vi "TLB Native Dynamic Events ver 0.22.vi"() -> ()   [LabVIEW 2018]
uses:
  Labview Training Phase 2/Enum Controls/States for Action Engine.ctl
  TLB Type Definitions/State Type Definitions.ctl
  TLB Type Definitions/Intruction Type Definitions.ctl
  TLB Type Definitions/Encoder cluster.ctl
  TLB Type Definitions/PING CLUSTER.ctl
  <vilib>/Studica/Studica Toolkit/NavX/NavX.lvlib
  <vilib>/Studica/Studica Toolkit/Background/DIO Channel.ctl
  Underlying VI's/NavX VI/navX type def.ctl
  <vilib>/Studica/Studica Toolkit/Background/I2C Channel.ctl
  TLB Type Definitions/Vision cluster.ctl
  <vilib>/NI_Real-Time Target Support.lvlib
  TLB Type Definitions/Stepper cluster.ctl
  Experimental VI's/Archived VI's/MOTOR CONTROL NO PID Type Def.ctl
  Underlying VI's/I2C Master VI/I2C MASTER Type Def.ctl
  Underlying VI's/I2C Master VI/I2C_MASTER_WRITE_NEW Type Def.ctl
  <vilib>/userdefined/High Color/IMAQdx.ctl
  Underlying VI's/I2C Master VI/Arduino_Interfacing.ctl
  TLB Type Definitions/Yaw Cluster.ctl
  TLB Type Definitions/Time cluster.ctl
  TLB Type Definitions/Y Stepper cluster.ctl
  Underlying VI's/Modified webcam FGV/Webcam AE.ctl
  Underlying VI's/Elasped Timer/Elapsed timer control.ctl
  Underlying VI's/Motor Control VI with PID/MOTOR CONTROL WITH PID AE DATA MODE TYPE DEF.ctl
  Underlying VI's/Motor Control VI with PID/MOTOR CONTROL WITH PID AE DIRECTION TYPE DEF.ctl
  TLB Type Definitions/IR Sensor Type Def.ctl
  <vilib>/myRIO/Common/Instrument Driver Framework/myRIO v1.0/AI/typedefs/AI Channels Enum.ctl
  <vilib>/myRIO/Common/Instrument Driver Framework/myRIO v1.0/AI/typedefs/AI Channels List.ctl
  TLB Type Definitions/Motor Speed Cluster.ctl
  Underlying VI's/IMAQ Create Reference AE/IMAQ Reference AE.ctl
  TLB Type Definitions/Line Sensor Cluster.ctl
  Underlying VI's/Line Sensor AE/Line Sensor AE Type Def.ctl
  <vilib>/Studica/Studica Toolkit/NavX/TypeDefs/Flags/Z900_navX_Flags_CalibrationStatusTypeDef.ctl
  <vilib>/Studica/Studica Toolkit/NavX/TypeDefs/Flags/Z900_navX_Flags_OpStatusTypeDef.ctl
panel:
  out "Front Wall detected":bool
  out "CPU 1 Usage":dbl
  out "CPU 0 Usage":dbl
  out "Line sensors":T1
  out "IR Sensors":T2
  out "Time up":T3
  out "NAVX Values":T4
  out "Stepper position values":T5
  out "Encoder values":T6
  out "Ultrasonic sensors":T7
  out "Stop?":bool
  out "Selected Task":T8=enum."Start Task 9"
  out "Object recognition mode":enum16{"Ball", "Soap", "Gel", "Pipe", "None"}(ring)
  out "Correcte stepper":u8
  out "Image Processing Error":errorcluster
  out "Object Detection":T9
  out "Status":T12 {"OP Status" items=["INITIALIZING", "SELFTEST_IN_PROGRESS", "ERROR", "IMU_AUTOCAL_IN_PROGRESS", "NORMAL"]; "Calibration Status" items=["IMU_CAL_STATE_MASK"=3, "IMU_CAL_STATE_INPROGRESS"=0, "IMU_CAL_STATE_ACCUMULATE"=1, "IMU_CAL_STATE_COMPLETE"=2]}
  out "General Errors":errorcluster
  in  "Red LED":bool
  out "Table obstruct":bool
  out "x-y":dbl
  out "Obstacle detected":bool
  out "Speed & distance":T13
  out "Task selection":u8
  out "NavX Readings":T14
  out "Arduino Data":T15
  out "TASK ENABLE":bool
  out "Rising Edge":bool
  in  "Green LED":bool
  out "State Logic":T16=enum."Startup"
  out "elements":T8[](array[typedef])
  in  "STOP TASK":bool
  in  "OK Button":bool
  in  "STOP":bool
  out "Queue Errors":errorcluster
  out "Action Queue Items":i32
  out "State Logic Queue Items":i32
  out "Action Queues items":string[](array[string])=["Hardware reset", "Software reset", ""]
  out "Action State":string
  # "VISION"
  # "TLB FRAMEWORK STATUS"
  # "System Health Status Update"
  # "Test Programme written by Calvin Loke    Dated: 28 Aug 2019\nTest Programme revised by Dr Alex See   Dated 30 Aug 2019\n\nRevision date: 20/03/2020\nProgramme version:   TLB Native Dynamic Events ver 0.19a"
  # "0: Task 1\n1: Task 2\n2: Task 3\n3: Task 4\n4: Task 5\n5: Task 6\n6: Task 7\n7: Task 8 Ball\n8: Task 8 Soap\n9: Task 8 Gel\n10: Task 8 Pipe\n11: Task 9 Blue\n12: Task 9 Black\n13: Task 9 Green\n14: Task 9 Red\n15: Task 9 Yellow"
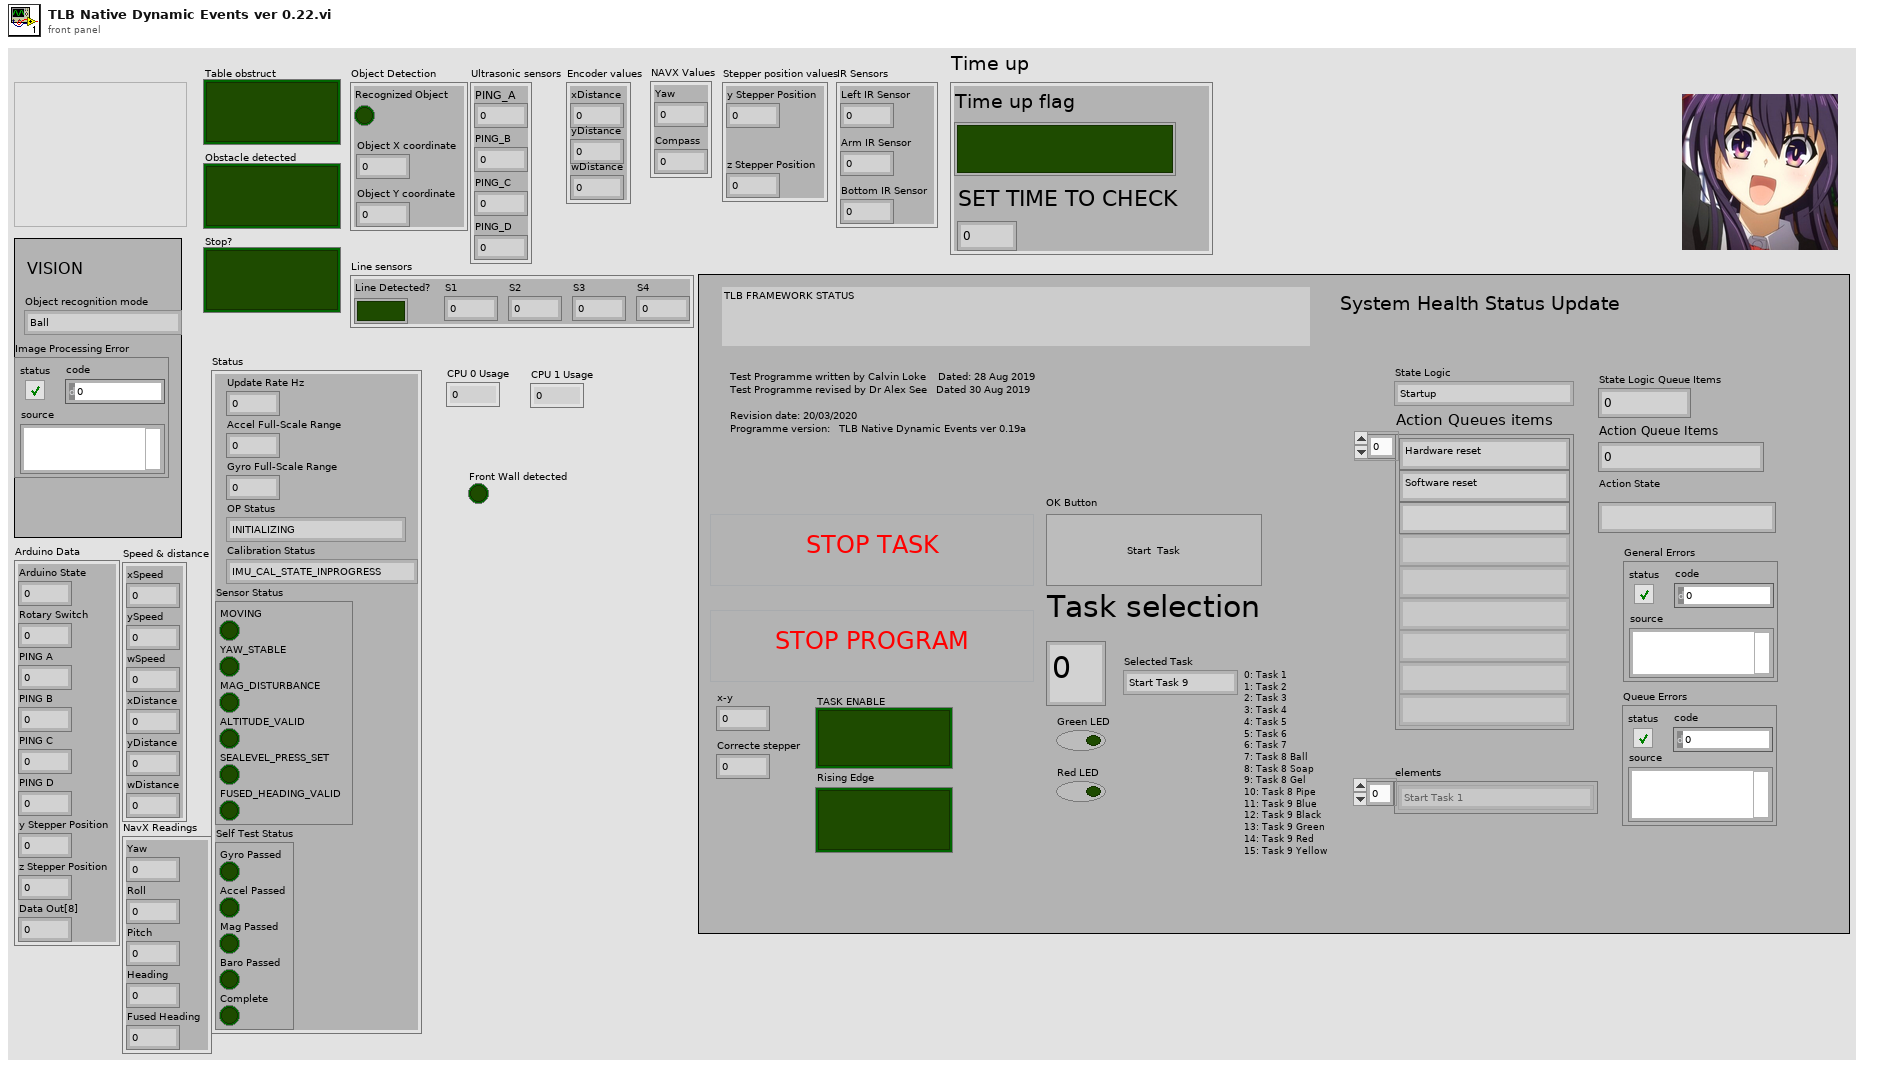
[diagram p1: front panel]
types:
  T1 = typedef "Line Sensor Cluster.ctl" = cluster{"Line Detected?":bool, "S1":dbl, "S2":dbl, "S3":dbl, "S4":dbl}
  T2 = typedef "IR Sensor Type Def.ctl" = cluster{"Left IR Sensor":dbl, "Arm IR Sensor":dbl, "Bottom IR Sensor":dbl}
  T3 = typedef "Time cluster.ctl" = cluster{"Time up flag":bool, "SET TIME TO CHECK":dbl}
  T4 = typedef "Yaw Cluster.ctl" = cluster{"Yaw":dbl, "Compass":dbl}
  T5 = typedef "Stepper cluster.ctl" = cluster{"y Stepper Position":u8, "z Stepper Position":u8}
  T6 = typedef "Encoder cluster.ctl" = cluster{"xDistance":dbl, "yDistance":dbl, "wDistance":dbl}
  T7 = typedef "PING CLUSTER.ctl" = cluster{"PING_A":u8, "PING_B":u8, "PING_C":u8, "PING_D":u8}
  T8 = typedef "Intruction Type Definitions.ctl" = enum16{"None", "Start Task 1", "Start Task 2", "Start Task 3", "Start Task 4", "Start Task 5", "Start Task 6", "Start Task 7", "Start Task 8 - BALL", "Start Task 8 - Gel", "Start Task 8 - Pipe", "Start Task 8 - Soap", "Start Task 9", "Start Task A", "Start Task B", "Exit"}
  T9 = typedef "Vision cluster.ctl" = cluster{"Recognized Object":bool, "Object X coordinate":dbl, "Object Y coordinate":dbl}
  T10 = typedef "NavX.lvlib/Z900_navX_Flags_OpStatusTypeDef.ctl" = u8
  T11 = typedef "NavX.lvlib/Z900_navX_Flags_CalibrationStatusTypeDef.ctl" = u8
  T12 = cluster{"Update Rate Hz":u8, "Accel Full-Scale Range":u8, "Gyro Full-Scale Range":u16, "OP Status":T10, "Calibration Status":T11, "Sensor Status":cluster{"MOVING":bool, "YAW_STABLE":bool, "MAG_DISTURBANCE":bool, "ALTITUDE_VALID":bool, "SEALEVEL_PRESS_SET":bool, "FUSED_HEADING_VALID":bool}, "Self Test Status":cluster{"Gyro Passed":bool, "Accel Passed":bool, "Mag Passed":bool, "Baro Passed":bool, "Complete":bool}}
  T13 = cluster{"xSpeed":dbl, "ySpeed":dbl, "wSpeed":dbl, "xDistance":dbl, "yDistance":dbl, "wDistance":dbl}
  T14 = cluster{"Yaw":dbl, "Roll":dbl, "Pitch":dbl, "Heading":dbl, "Fused Heading":dbl}
  T15 = cluster{"Arduino State":u8, "Rotary Switch":u8, "PING A":u8, "PING B":u8, "PING C":u8, "PING D":u8, "y Stepper Position":u8, "z Stepper Position":u8, "Data Out[8]":u8}
  T16 = typedef "State Type Definitions.ctl" = enum16{"None", "Startup", "Move to Angle", "True Stop", "Idle", "Shutdown", "Task 1A", "Task 1B", "Task 2:Raise Arm", "Task 2:Sensor Mode", "Task 2:Reverse Mode", "Task 3", "Task 4_A", "Task 4_B", "Task 4_C", "Task 4_D", "Task 5A", "Task 5B", "Task 5C", "Task 5D", "Task 5E: POSITION ARM", "Task 5F: ARM GRAB HEIGHT", "Task 5G: CLOSE CLAW", "Task 5H: RAISE ARM", "Task 6_A", "Task 6_B", "Task 7", "Task 8A: RAISE ARM", "Task 8B: MOVE TO BOX", "Task 8C: CAM BURST", "Task 8D: PROCESS IMAGE", "Task 8E: ROBOT ADJUST", "Task 8F: CAM BURST 2", "Task 8G: PROCESS IMAGE 2", "Task 8H: ARM ADJUST", "Task 8I: ARM GRAB HEIGHT", "Task 8J: CLOSE CLAW", "Task 8K: RAISE MY SWORD", "Task 9A: Raise Arm", "Task 9B: Rotate to Angle", "Task 9C: Detect Box", "Task 9D: MOVE FORWARD", "Task 9E: MOVE LEFT", "Task 9F: SCAN IMAGE", "Task 9G: PROCESS COLOUR", "Task 9H: MOVE RIGHT", "Task 9I: SCAN IMAGE", "Task 9J: PROCESS COLOUR", "Task 9K: ROTATE 90 CW", "Task 9L: MOVE FORWARD", "Task 9M: MOVE RIGHT", "Task 9N: SCAN IMAGE", "Task 9O: PROCESS COLOUR", "Task 9P: MOVE RIGHT", "Task 9Q: SCAN IMAGE", "Task 9R: PROCESS COLOUR", "Task A1: Raise Arm", "Task A2: Rotate to Angle", "Task A3: Move Forward", "Task A4: Rotate CW 90"}
  T17 = typedef "Motor Speed Cluster.ctl" = cluster{"ySpeed":dbl, "xSpeed":dbl, "wSpeed":dbl}
  T18 = typedef "Y Stepper cluster.ctl" = cluster{"yStepper desired":u8}
  T19 = typedef "DIO Channel.ctl" = enum16{"Not Connected", "A/DIO1", "A/DIO2", "A/DIO3", "A/DIO4", "A/DIO5", "A/DIO6", "A/DIO7", "A/DIO13", "B/DIO1", "B/DIO2", "B/DIO3", "B/DIO4", "B/DIO5", "B/DIO6", "B/DIO7", "B/DIO13", "C/DIO0", "C/DIO1", "C/DIO2", "C/DIO3", "C/DIO4", "C/DIO5", "C/DIO6", "C/DIO7"}
  T20 = cluster{"DIO Channel":T19, "FPGA VI Reference Out":refnum<k20>}
  T21 = typedef "States for Action Engine.ctl" = enum16{"Initialize", "Write", "Read"}
  T22 = typedef "NI_Real-Time Target Support.lvlib/RT CPU Load.ctl" = cluster{"Total (%)":dbl, "Time Critical (%)":dbl, "Timed Structures (%)":dbl, "High (%)":dbl, "Above Normal (%)":dbl, "Normal (%)":dbl, "Background (%)":dbl, "Idle (%)":dbl, "ISR (%)":dbl}
  T23 = cluster{"CPU loads[0]":T22, "CPU loads[1]":T22, "CPU loads[2]":T22, "CPU loads[3]":T22, "CPU loads[4]":T22, "CPU loads[5]":T22, "CPU loads[6]":T22, "CPU loads[7]":T22, "CPU loads[8]":T22}
  T24 = typedef "navX type def.ctl" = enum16{"Get i2C reference", "Read Values", "Zero Yaw"}
  T25 = typedef "Arduino_Interfacing.ctl" = enum16{"Initialize", "Write to Arduino", "Read From Arduino"}
  T26 = typedef "I2C Channel.ctl" = enum16{"Not Connected", "A", "B"}
  T27 = cluster{"I2C Ref Out":cluster{"I2C Channel":T26, "FPGA VI Reference Out":refnum<k20>}, "Connected":bool, "Slave Address (7-bit)":u8, "Registry":u8[]}
  T28 = typedef "State Type Definitions.ctl" = enum16{"None", "Startup", "Move to Angle", "True Stop", "Idle", "Shutdown", "Task 1", "Task 2:Raise Arm", "Task 2:Sensor Mode", "Task 2:Reverse Mode", "Task 3", "Task 4_A", "Task 4_B", "Task 4_C", "Task 4_D", "Task 5A: ARM CAM HEIGHT", "Task 5B: MOVE TO BOX", "Task 5C: CAM BURST", "Task 5D: PROCESS IMAGE", "Task 5E: POSITION ARM", "Task 5F: ARM GRAB HEIGHT", "Task 5G: CLOSE CLAW", "Task 5H: RAISE ARM", "Task 6_A", "Task 6_B", "Task 7", "Task 8A: RAISE ARM", "Task 8B: MOVE TO BOX", "Task 8C: CAM BURST", "Task 8D: PROCESS IMAGE", "Task 8E: ROBOT ADJUST", "Task 8F: CAM BURST 2", "Task 8G: PROCESS IMAGE 2", "Task 8H: ARM ADJUST", "Task 8I: ARM GRAB HEIGHT", "Task 8J: CLOSE CLAW", "Task 8K: RAISE MY SWORD", "Task 9A: Raise Arm", "Task 9B: Rotate to Angle", "Task 9C: Detect Box", "Task 9D: MOVE FORWARD", "Task 9E: MOVE LEFT", "Task 9F: SCAN IMAGE", "Task 9G: PROCESS COLOUR", "Task 9H: MOVE RIGHT", "Task 9I: SCAN IMAGE", "Task 9J: PROCESS COLOUR", "Task 9K: ROTATE 90 CW", "Task 9L: MOVE FORWARD", "Task 9M: MOVE RIGHT", "Task 9N: SCAN IMAGE", "Task 9O: PROCESS COLOUR", "Task 9P: MOVE RIGHT", "Task 9Q: SCAN IMAGE", "Task 9R: PROCESS COLOUR"}
  T29 = typedef "MOTOR CONTROL WITH PID AE DIRECTION TYPE DEF.ctl" = enum16{"y-axis movement", "x-axis movement", "rotation", "stop", "reset encoders"}
  T30 = typedef "MOTOR CONTROL WITH PID AE DATA MODE TYPE DEF.ctl" = enum16{"Init AE", "Write to AE", "Read from AE"}
  T31 = typedef "Line Sensor AE Type Def.ctl" = enum16{"INIT AE", "READ FROM LINE SENSORS"}
  T32 = typedef "IMAQ Reference AE.ctl" = enum16{"Initialize AE", "Get IMAQ Reference", "Dispose Processing Buffer"}
  T33 = typedef "Elapsed timer control.ctl" = enum16{"Start", "Pause", "Initialize"}
  T34 = typedef "I2C_MASTER_WRITE_NEW Type Def.ctl" = enum16{"Ultrasonic sensors", "Stepper origin", "zStepper 13.3k", "zStepper 13k", "zStepper 12k", "zStepper 11k", "zStepper 10k", "zStepper 9k", "zStepper 8k", "zStepper 7k", "zStepper 6k", "zStepper 5k", "zStepper 4k", "zStepper 3k", "zStepper 2k", "zStepper 1k", "zStepper 900", "zStepper 800", "zStepper 700", "zStepper 600", "zStepper 500", "zStepper 400", "zStepper 300", "zStepper 200", "zStepper 100", "zStepper 0", "yStepper control", "Open Claw", "Close Claw", "Soft Reset"}
  T35 = typedef "Webcam AE.ctl" = enum16{"Initialize Camera", "Open Camera", "Continuous Acquisition", "Close Camera", "Retrieve Image", "Dispose Camera Image Buffer"}
  T36 = typedef "IMAQdx.ctl" = refnum<k21>
  T37 = typedef "MOTOR CONTROL NO PID Type Def.ctl" = enum16{"Init", "Front Back", "Left Right", "Rotate", "Stop", "Latch"}
  T38 = typedef "AI Channels List.ctl" = T39[]
  T39 = typedef "AI Channels Enum.ctl" = enum16{"Not Connected", "AudioIn/Left", "AudioIn/Right", "C/AI0", "C/AI1", "A/AI0", "A/AI1", "A/AI2", "A/AI3", "A/AI4", "A/AI5", "A/AI6", "A/AI7", "B/AI0", "B/AI1", "B/AI2", "B/AI3", "B/AI4", "B/AI5", "B/AI6", "B/AI7", "AI/AI0", "AI/AI1", "AI/AI2", "AI/AI3", "A/AI0 (DIFF)", "A/AI1 (DIFF)", "A/AI2 (DIFF)", "A/AI3 (DIFF)", "B/AI0 (DIFF)", "B/AI1 (DIFF)", "B/AI2 (DIFF)", "B/AI3 (DIFF)"}
  T40 = cluster{"S1":dbl, "S2":dbl, "S3":dbl, "S4":dbl, "Array[4]":dbl, "Array[5]":dbl, "Array[6]":dbl, "Array[7]":dbl, "Array[8]":dbl}
  T41 = typedef "I2C MASTER Type Def.ctl" = enum16{"Last State", "Mode 0", "Mode 1", "Mode 2", "Mode 3", "Mode 4", "Mode 5", "Mode 6", "Mode 7", "Mode 8", "Mode 9", "Mode 10"}
  T42 = typedef "IMAQ Image.ctl" = refnum<image>
  T43 = cluster{"Number of Matches":i32, "Object detected?":bool}
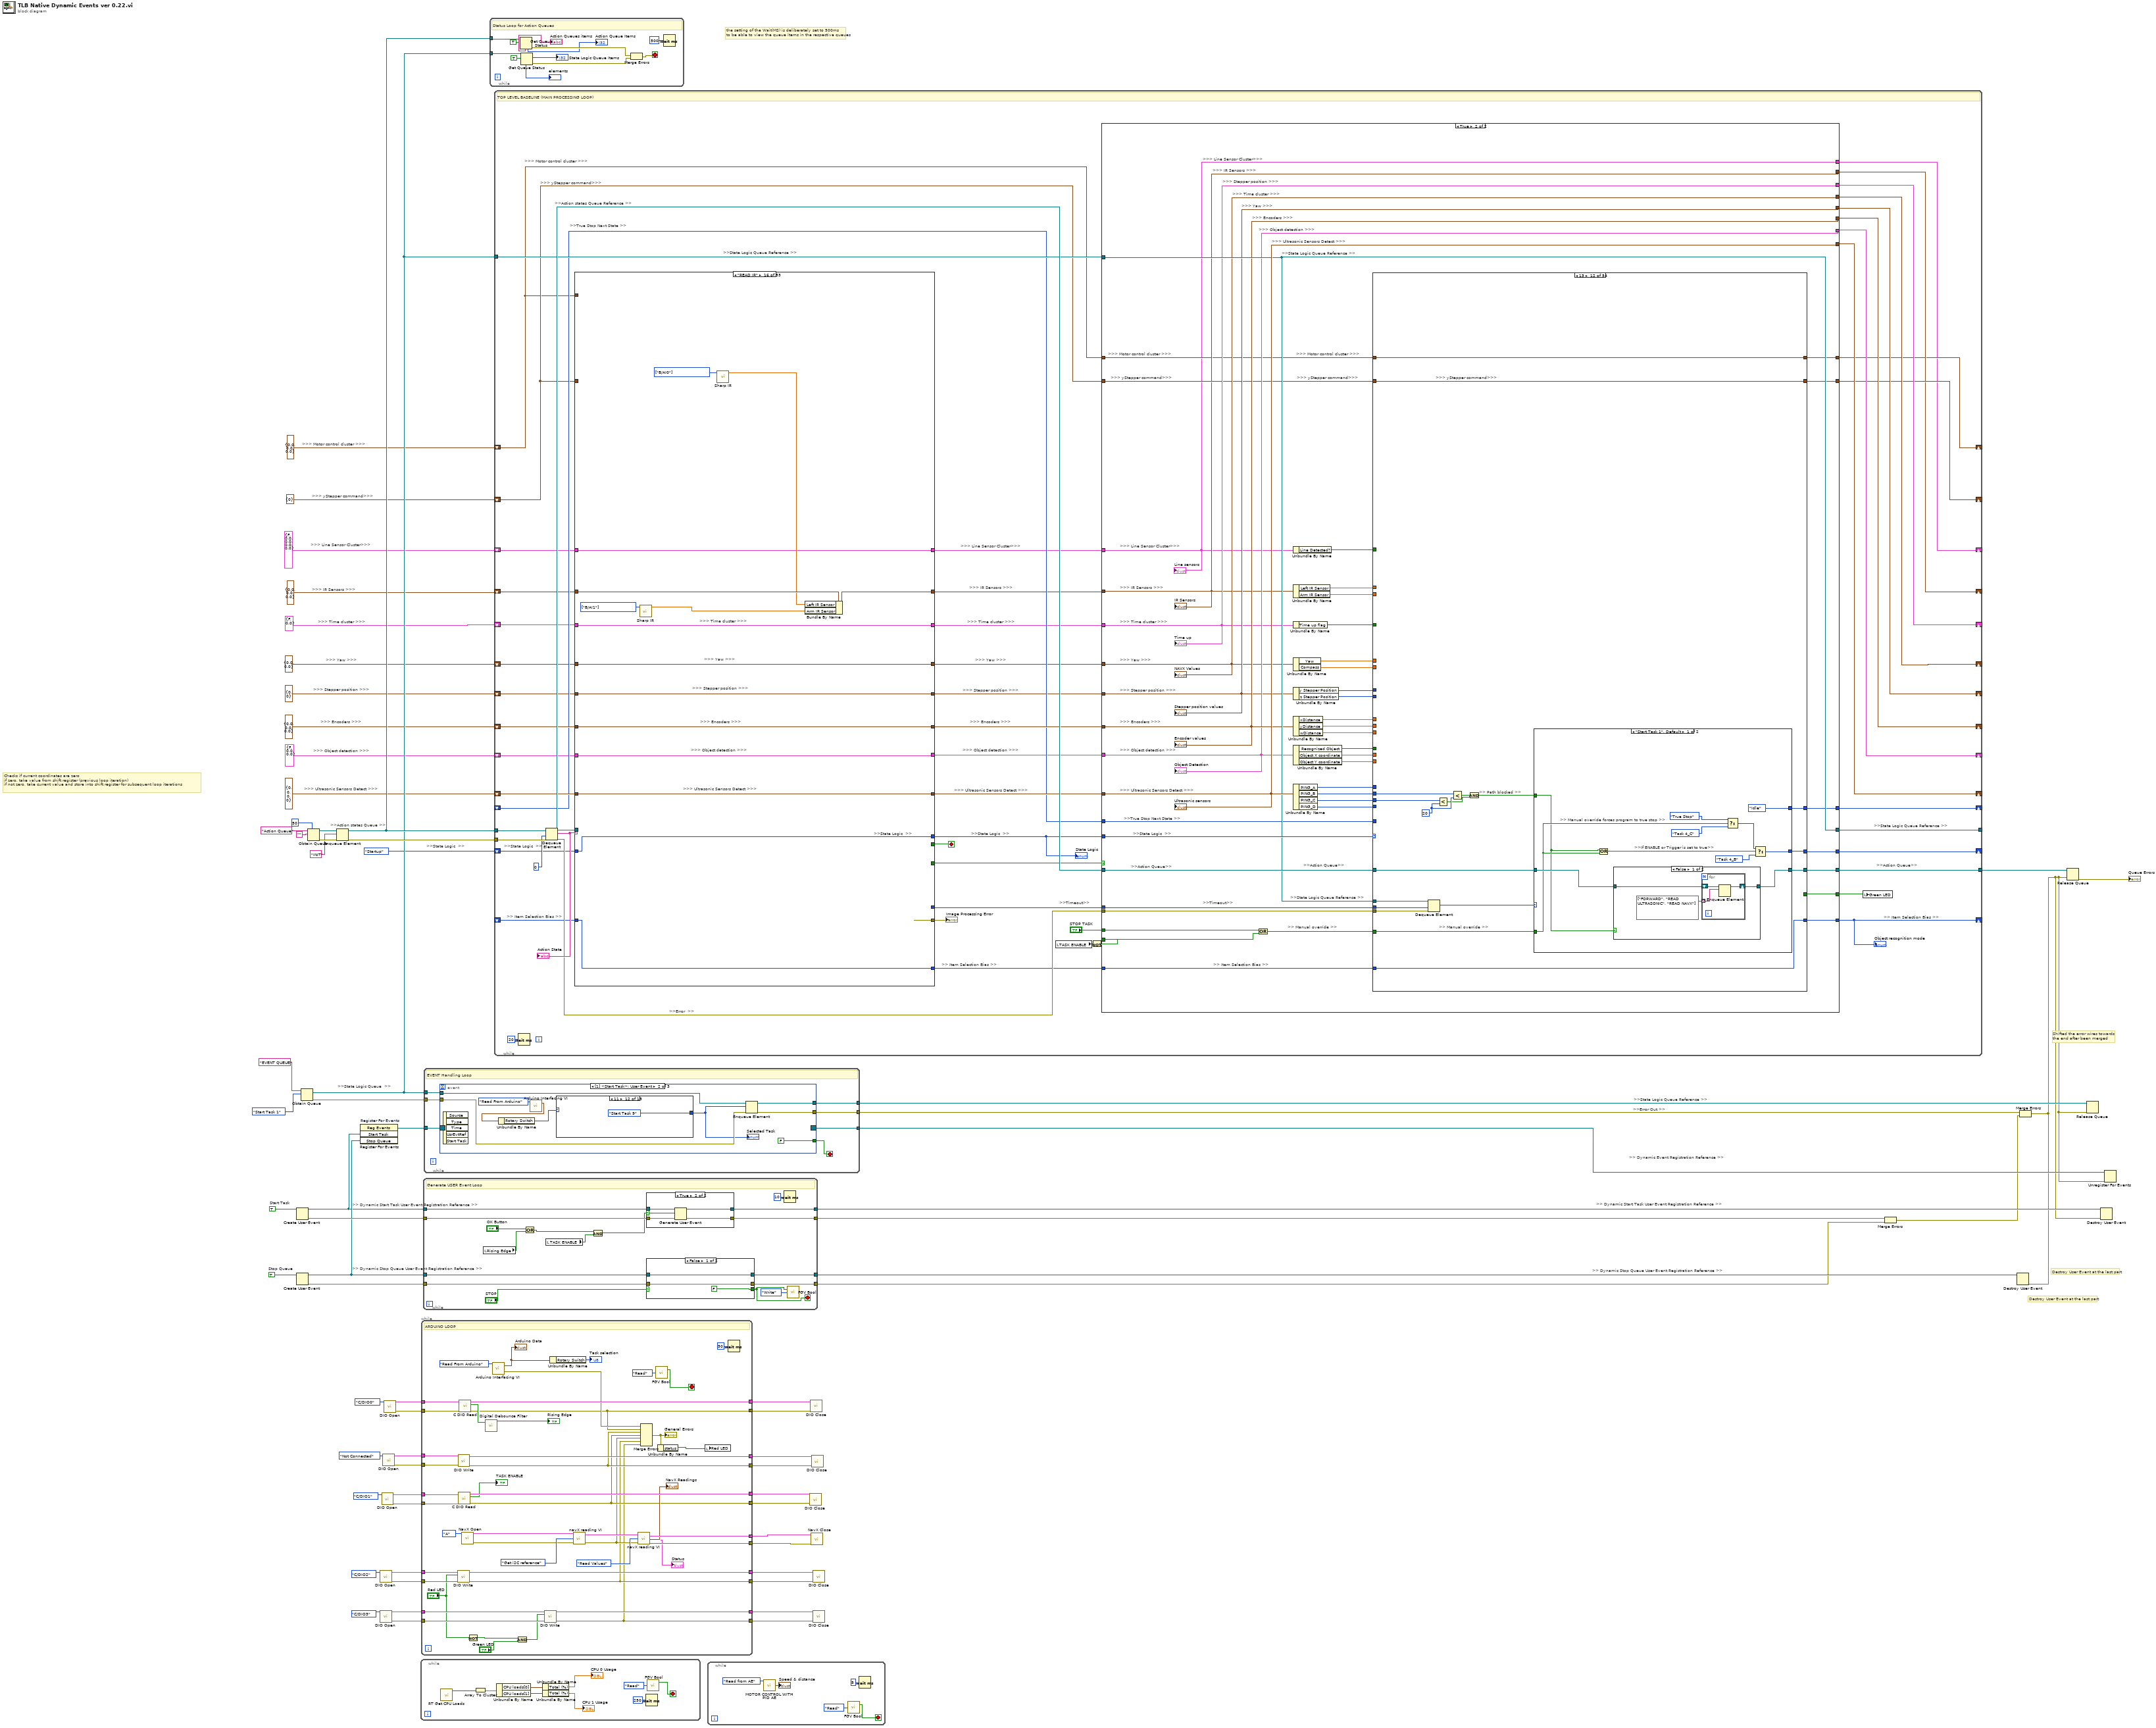
[diagram p0: block diagram]
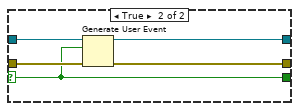
[diagram p2: hidden frame]
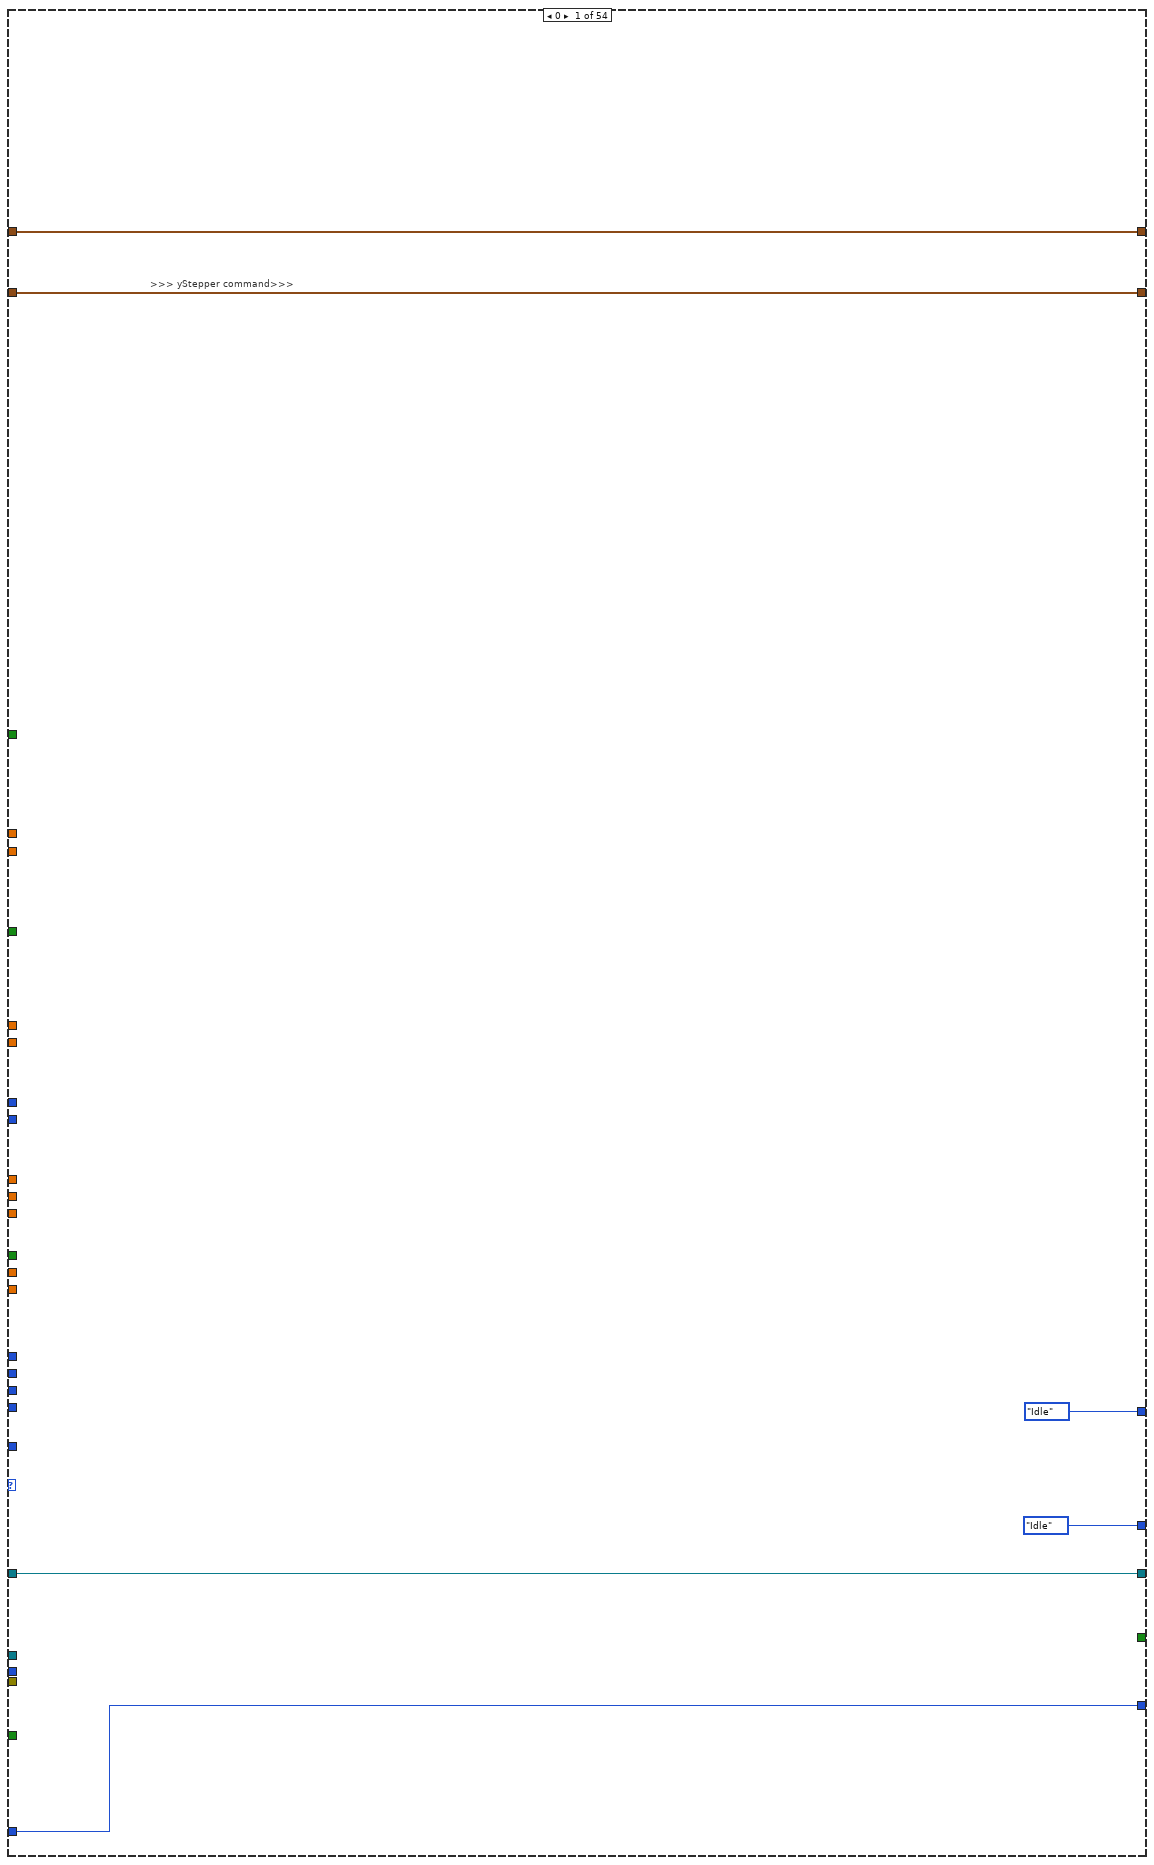
[diagram p5: hidden frame]
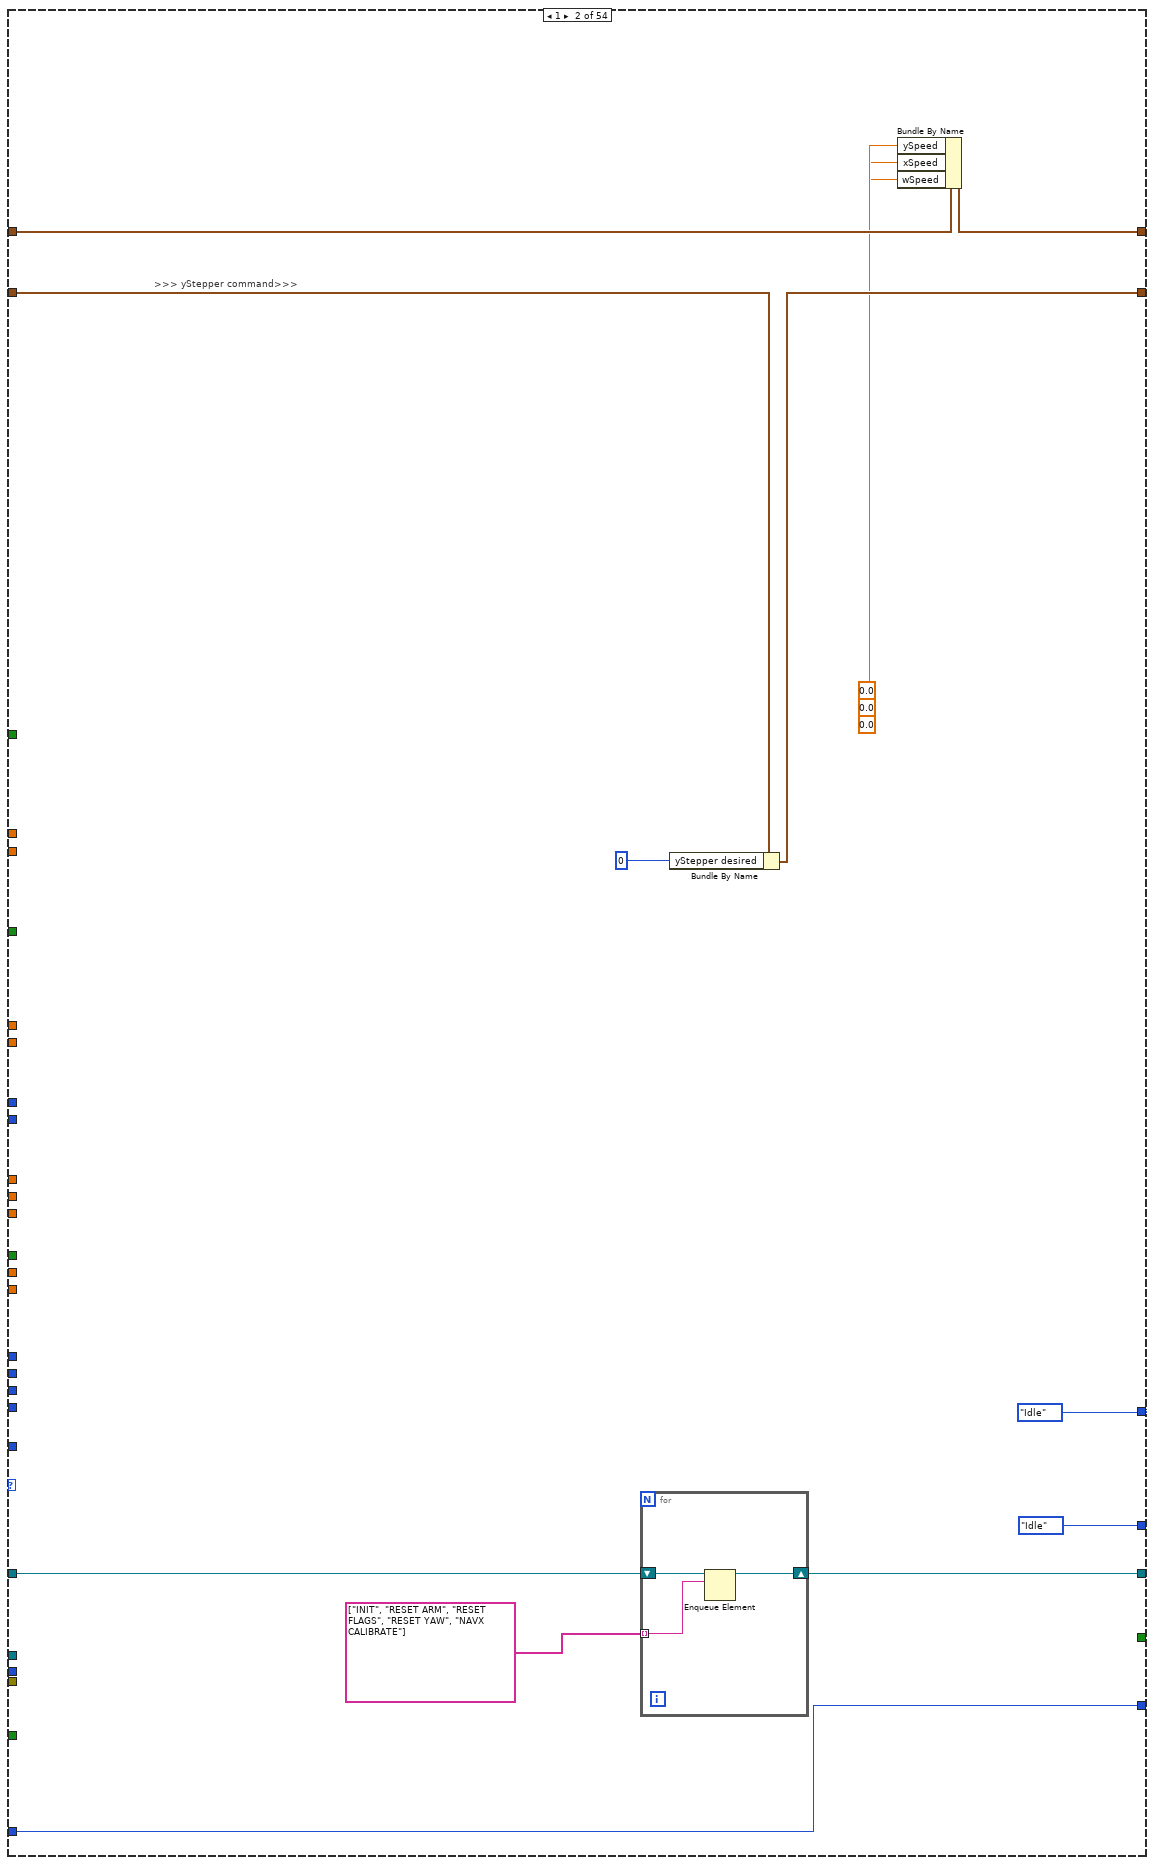
[diagram p6: hidden frame]
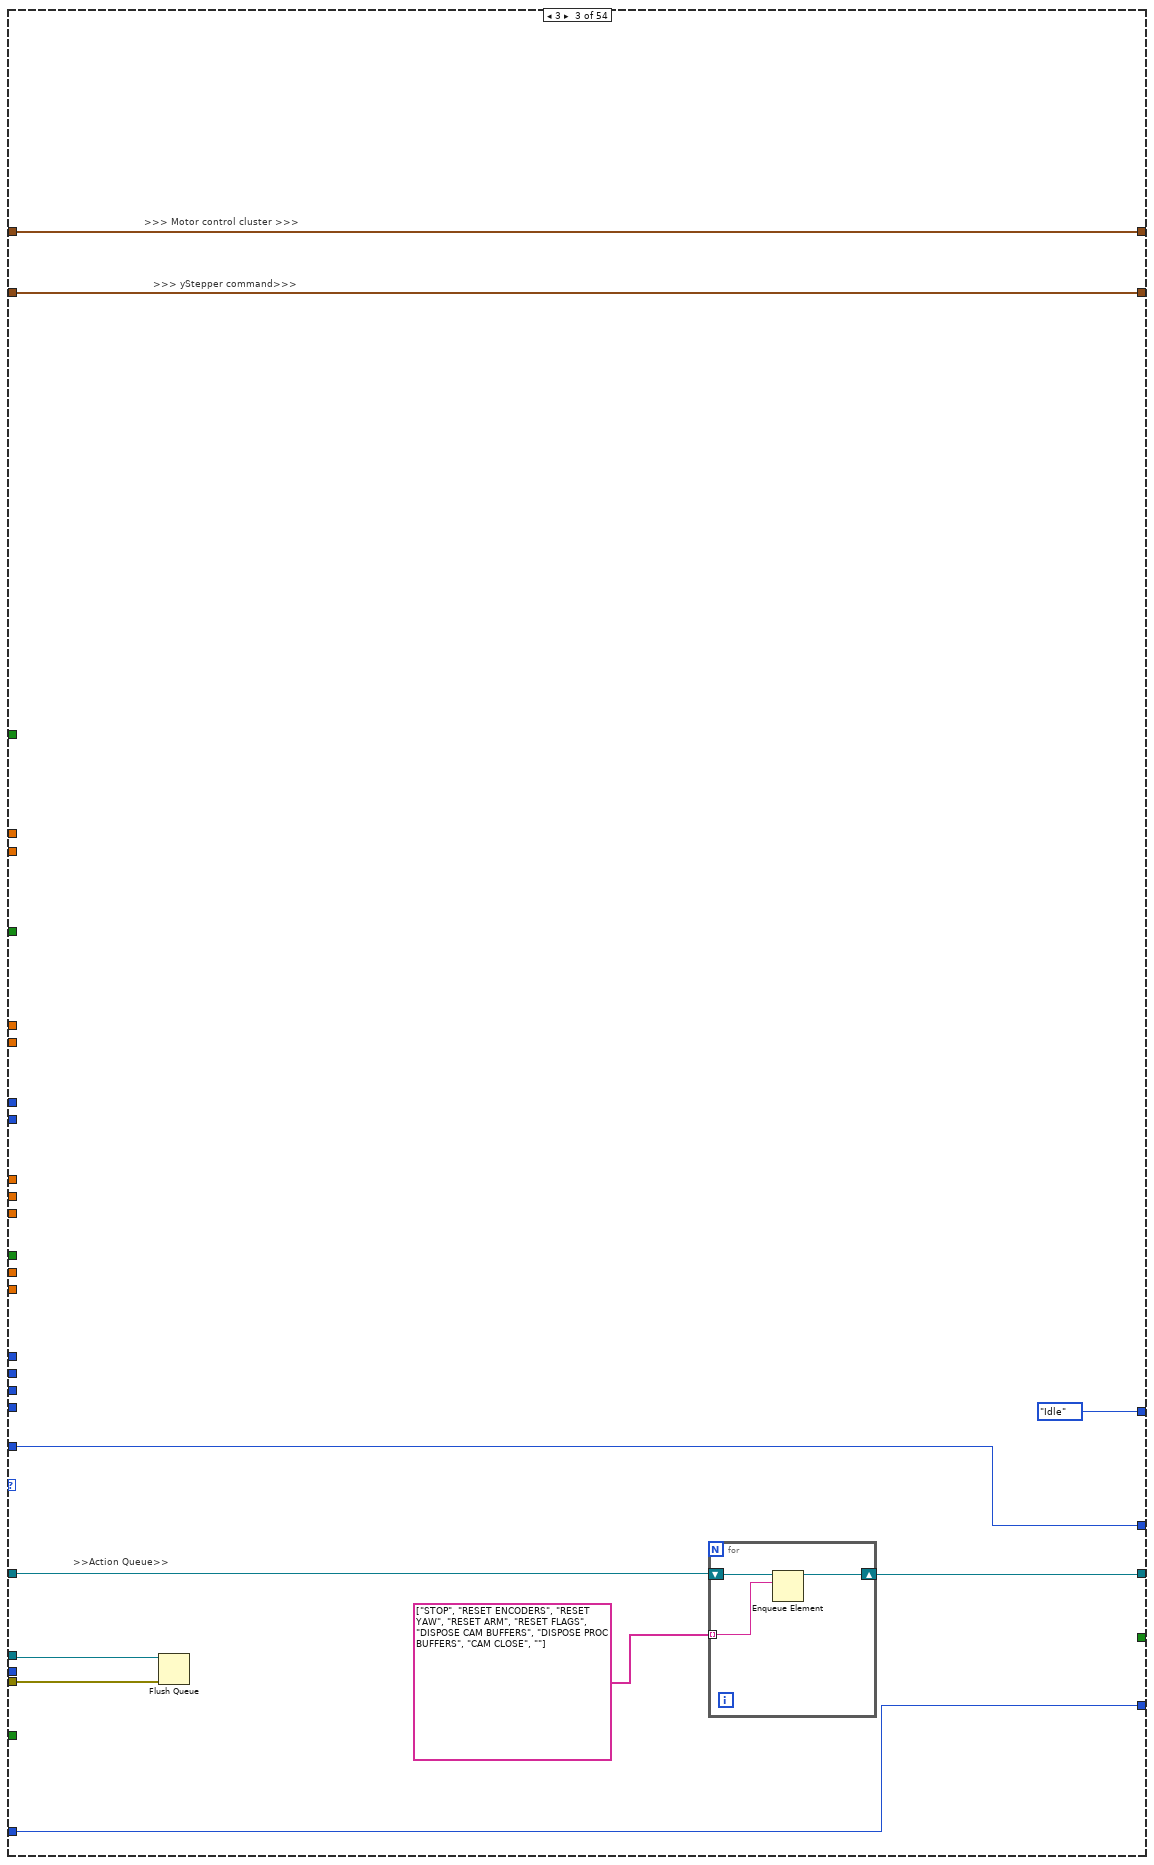
[diagram p7: hidden frame]
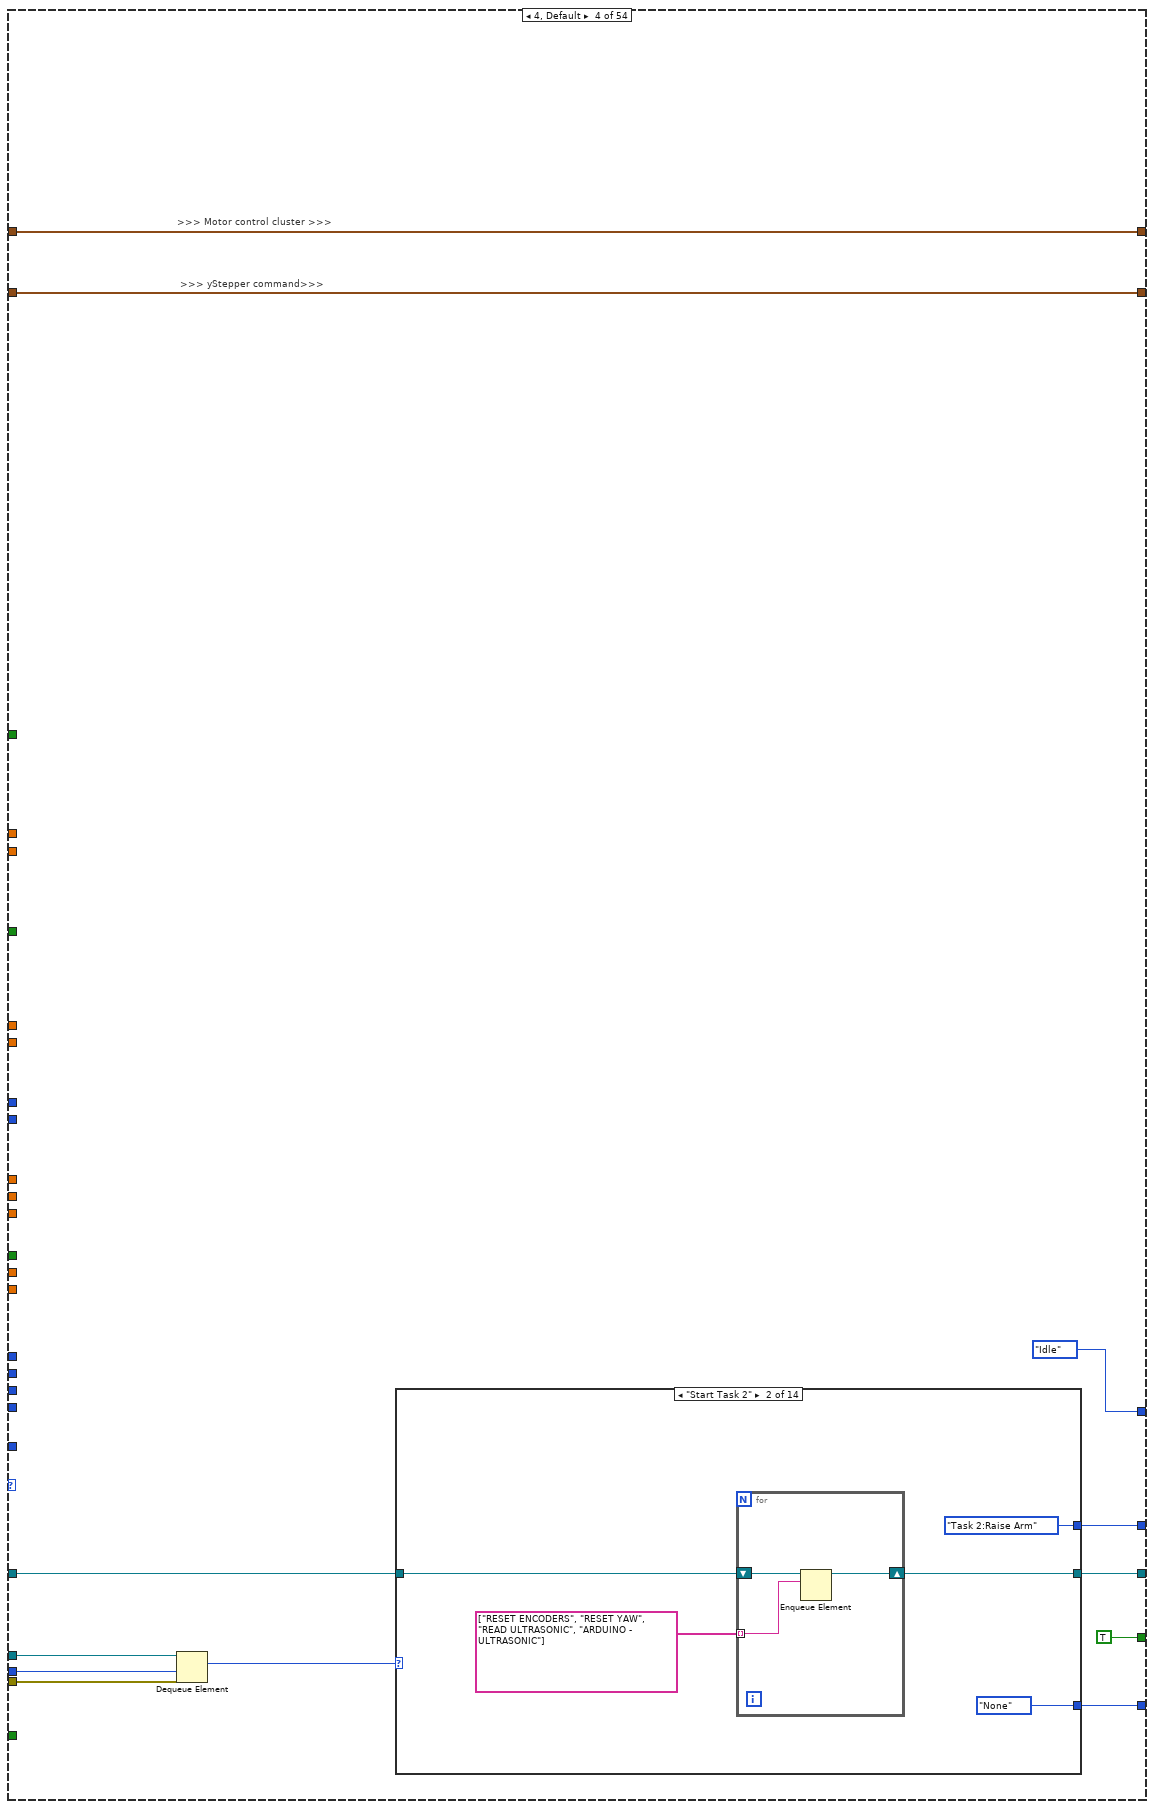
[diagram p8: hidden frame]
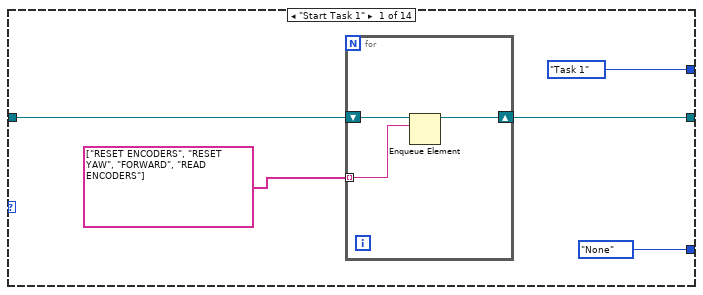
[diagram p9: hidden frame]
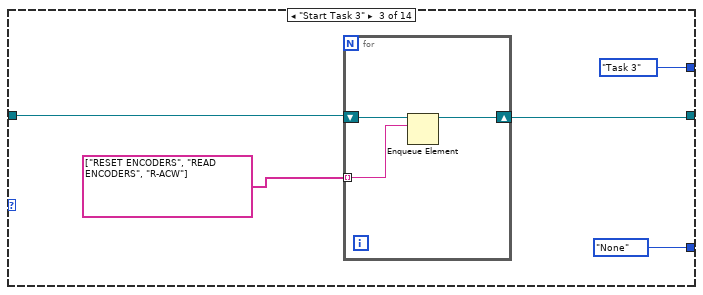
[diagram p10: hidden frame]
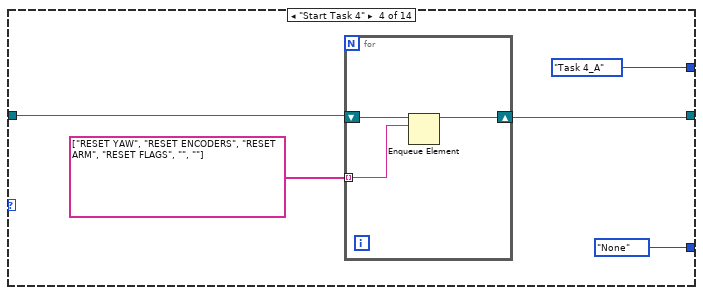
[diagram p11: hidden frame]
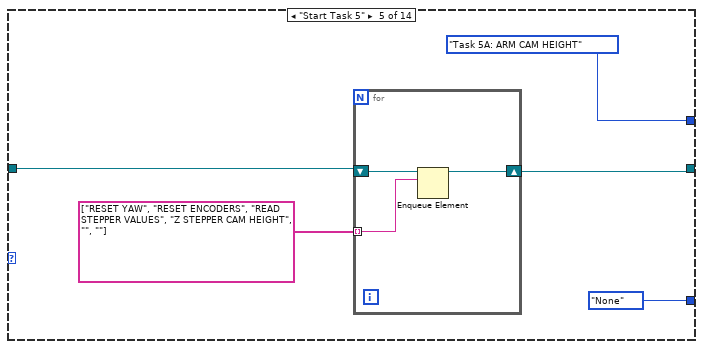
[diagram p12: hidden frame]
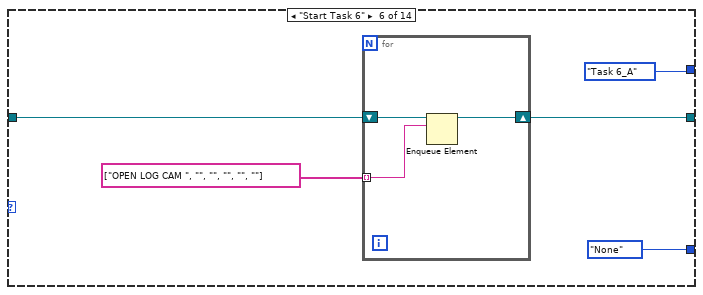
[diagram p13: hidden frame]
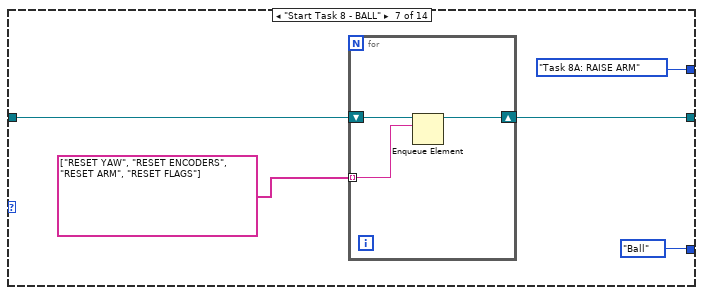
[diagram p14: hidden frame]
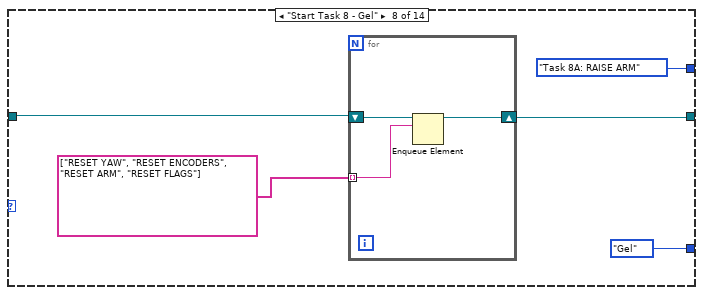
[diagram p15: hidden frame]
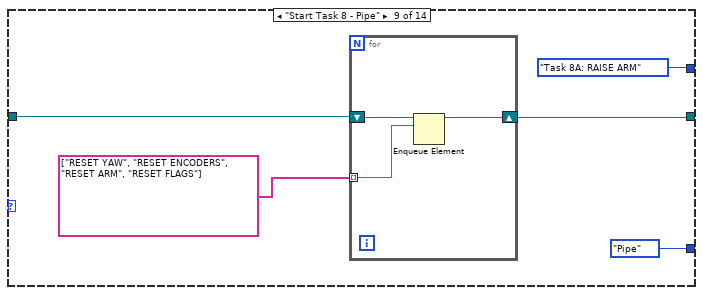
[diagram p16: hidden frame]
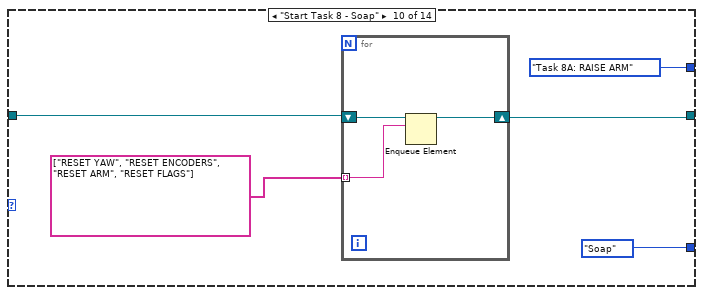
[diagram p17: hidden frame]
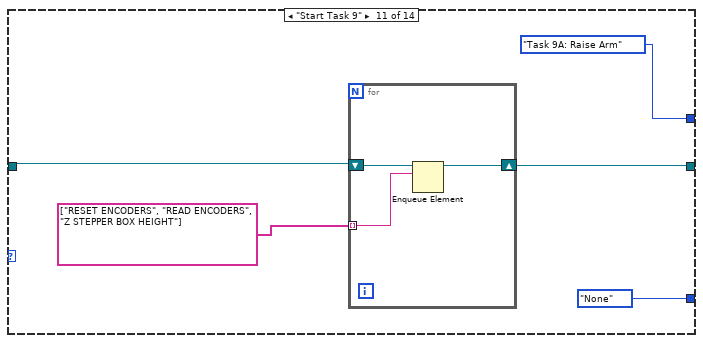
[diagram p18: hidden frame]
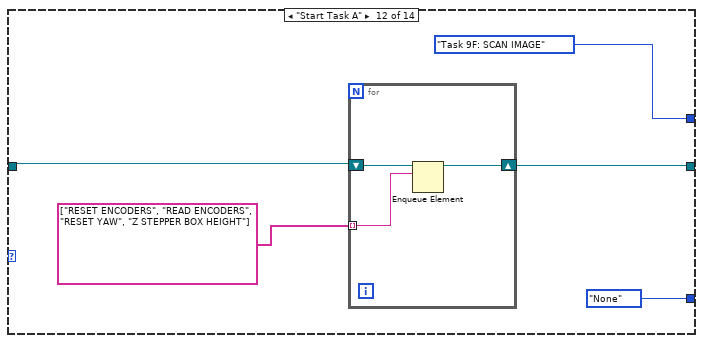
[diagram p19: hidden frame]
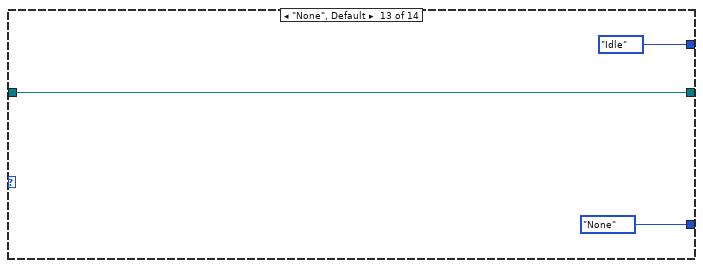
[diagram p20: hidden frame]
diagram:
  w68 = TRUE  # Stop Queue
  w67 = TRUE  # Start Task
  # ">>State Logic  >>"
  # ">>> Line Sensor Cluster>>>"
  # ">>> Motor control cluster >>>"
  # ">>> IR Sensors >>>"
  # "Checks if current coordinates are zero\nif zero, take value from shift register (previous loop iteration)\nif not zero, take current value and store into shift register for subsequent loop iterations"
  # ">>> yStepper command>>>"
  # ">>> Time cluster >>>"
  # ">>> Yaw >>>"
  # ">>> Stepper position >>>"
  # ">>> Encoders >>>"
  # ">>> Object detection >>>"
  # ">>> Ultrasonic Sensors Detect >>>"
  # "the setting of the Wait(MS) is deliberately set to 500ms\nto be able to view the queue items in the respective queues"
  # ">>Error Out >>"
  # ">> Dynamic Stop Queue User Event Registration Reference >>"
  # ">> Dynamic Start Task User Event Registration Reference >>"
  # ">> Dynamic Stop Queue User Event Registration Reference >>"
  # ">> Dynamic Start Task User Event Registration Reference >>"
  # ">> Dynamic Event Registration Reference >>"
  # ">>Action states Queue >>"
  # ">>State Logic Queue  >>"
  # ">>State Logic Queue Reference >>"
  # "Destroy User Event at the last part"
  # "Destroy User Event at the last part"
  # "Shifted the error wires towards\nthe end after been merged"
  n1 = Create User Event(user event datatype=w67) -> (user event=w59:refnum<user-event>, error out=w64:errorcluster)  [unwired: 1 in]
  n2 = Create User Event(user event datatype=w68) -> (user event=w60:refnum<user-event>, error out=w63:errorcluster)  [unwired: 1 in]
  n3 = Obtain Queue(name (unnamed)="EVENT QUEUE", element data type=Intruction_Type_Definitions."Start Task 1" ("Enum")) -> (queue out=w45:refnum<queue>, error out=w51:errorcluster)  [unwired: 3 in, 1 out]
  n4 = Obtain Queue(max queue size (-1, unlimited)=50, name (unnamed)="Action Queue", element data type="") -> (queue out=w54:refnum<queue>, error out=w50:errorcluster)  [unwired: 2 in, 1 out]
  n5 = Enqueue Element(queue=w54, element="INIT", error in (no error)=w50) -> (queue out=w46:refnum<queue>, error out=w49:errorcluster)  [unwired: 1 in, 1 out]
  n6 = register-events "Register For Events"(w59, w60) -> (reference out=w58:refnum<event-registration>)  [unwired: 2 in, 1 out]
  n7 = call <vilib>:"DIO Open.vi"("DIO Channel"=DIO_Channel."C/DIO2") -> ("error out"=w18:errorcluster, "DIO Info Out"=w19:T20)  [unwired: 9 in]
  n8 = call <vilib>:"DIO Open.vi"("DIO Channel"=DIO_Channel."C/DIO3") -> ("error out"=w13:errorcluster, "DIO Info Out"=w14:T20)  [unwired: 9 in]
  n9 = call <vilib>:"DIO Open.vi"("DIO Channel"=DIO_Channel."C/DIO1") -> ("error out"=w23:errorcluster, "DIO Info Out"=w24:T20)  [unwired: 9 in]
  n10 = call <vilib>:"DIO Open.vi"("DIO Channel"=DIO_Channel."Not Connected") -> ("error out"=w28:errorcluster, "DIO Info Out"=w30:T20)  [unwired: 9 in]
  n11 = call <vilib>:"DIO Open.vi"("DIO Channel"=DIO_Channel."C/DIO0") -> ("error out"=w33:errorcluster, "DIO Info Out"=w36:T20)  [unwired: 9 in]
  n12 = while {
    stop <- w75 stop-if-true
    n13 = call <vilib>:"RT Get CPU Loads.vi"() -> ("CPU loads"=w74:T22[])  [unwired: 10 in, 1 out]
    n14 = Array To Cluster(array=w74) -> (cluster=w73:T23)
    n15 = Unbundle By Name(w73) -> ("CPU loads[0]"=w72:T22, "CPU loads[1]"=w71:T22)
    n16 = Unbundle By Name(w72) -> ("Total (%)"=→"CPU 0 Usage":dbl)
    n17 = Unbundle By Name(w71) -> ("Total (%)"=→"CPU 1 Usage":dbl)
    n18 = Wait (ms)(milliseconds to wait=u32 250) -> ()  [unwired: 1 out]
    n19 = call "FGV Bool.vi"("Init/Read/Write State"=States_for_Action_Engine."Read") -> ("Output node"=w75:bool)  [unwired: 2 in, 1 out]
  }
  n20 = while {
    tunnel: w36 -> [w121]
    tunnel: [w120] -> w34
    tunnel: w33 -> [w119]
    tunnel: [w90] -> w32
    tunnel: w30 -> [w116]
    tunnel: [w115] -> w29
    tunnel: w28 -> [w114]
    tunnel: [w89] -> w27
    tunnel: [w113] -> w25
    tunnel: w24 -> [w112]
    tunnel: w23 -> [w111]
    tunnel: [w88] -> w22
    tunnel: w19 -> [w105]
    tunnel: w18 -> [w104]
    tunnel: [w103] -> w17
    tunnel: [w86] -> w16
    tunnel: w14 -> [w102]
    tunnel: w13 -> [w101]
    tunnel: [w100] -> w12
    tunnel: [w85] -> w11
    tunnel: [w97] -> w8
    tunnel: [w96] -> w9
    stop <- w123 stop-if-true
    # "ARDUINO LOOP"
    n21 = call <vilib>:"DIO Write.vi"("error in (no error)"=w104, "Input"="Red LED", "DIO Info In"=w105) -> ("error out"=w86:errorcluster, "DIO Info Out"=w103:T20)  [unwired: 7 in]
    n22 = call <vilib>:"DIO Write.vi"("error in (no error)"=w114, "DIO Info In"=w116) -> ("error out"=w89:errorcluster, "DIO Info Out"=w115:T20)  [unwired: 8 in]
    n23 = call <vilib>:"C DIO Read.vi"("error in (no error)"=w111, "DIO Info In in"=w112) -> ("error out"=w88:errorcluster, "IN"=→"TASK ENABLE":bool, "DIO Info In out"=w113:T20)  [unwired: 7 in]
    n24 = call <vilib>:"C DIO Read.vi"("error in (no error)"=w119, "DIO Info In in"=w121) -> ("error out"=w90:errorcluster, "IN"=w118:bool, "DIO Info In out"=w120:T20)  [unwired: 7 in]
    n25 = call <vilib>:"NavX Open.vi"("I2C Channel"=I2C_Channel."A") -> ("error out"=w107:errorcluster, "NavX Info"=w109:T27)  [unwired: 9 in]
    n26 = Not(x="Red LED") -> (.not. x?=w79:bool)
    n27 = call "Digital Debounce Filter.vi"("Boolean input"=w118) -> ("Rising Edge"=→"Rising Edge":bool)  [unwired: 1 in, 2 out]
    n28 = call "Arduino Interfacing VI.vi"("AE Mode"=Arduino_Interfacing."Read From Arduino") -> ("error out"=w91:errorcluster, "Arduino Data"=w93:T15)  [unwired: 3 in]
    "Arduino Data" <- w93
    n29 = And(x=w79, y="Green LED") -> (x .and. y?=w82:bool)
    n30 = call <vilib>:"DIO Write.vi"("error in (no error)"=w101, "Input"=w82, "DIO Info In"=w102) -> ("error out"=w85:errorcluster, "DIO Info Out"=w100:T20)  [unwired: 7 in]
    n31 = Unbundle By Name(w93) -> ("Rotary Switch"=→"Task selection":u8)
    n32 = call "navX reading VI.vi"("NavX Info In"=w109, "Mode"=navX_type_def."Get i2C reference", "error in (no error)"=w107) -> ("NavX Info Out"=w98:T27, "Error Out"=w87:errorcluster)  [unwired: 2 out]
    n33 = call "navX reading VI.vi"("NavX Info In"=w98, "Mode"=navX_type_def."Read Values", "error in (no error)"=w87) -> ("NavX Info Out"=w97:T27, "NavX Readings"=→"NavX Readings":T14, "Status"=→"Status":T12, "Error Out"=w96:errorcluster)
    n34 = Merge Errors(w91, w90, w89, w88, w87, w86, w85) -> (w83:errorcluster)
    "General Errors" <- w83
    n35 = call "FGV Bool.vi"("Init/Read/Write State"=States_for_Action_Engine."Read") -> ("Output node"=w123:bool)  [unwired: 2 in, 1 out]
    n36 = Unbundle By Name(w83) -> ("status"=w80:bool)
    n37 = local write "Red LED"(w80) -> ()
    n38 = Wait (ms)(milliseconds to wait=u32 50) -> ()  [unwired: 1 out]
  }
  n39 = while {
    tunnel: w59 -> [w141]
    tunnel: w60 -> [w140]
    tunnel: [w139] -> w66
    tunnel: [w138] -> w65
    tunnel: w64 -> [w137]
    tunnel: [w136] -> w62
    tunnel: w63 -> [w135]
    tunnel: [w134] -> w61
    stop <- w132 stop-if-true
    # "Generate USER Event Loop"
    n40 = local read "Rising Edge"() -> (w129:bool)
    n41 = Or(x="OK Button", y=w129) -> (x .or. y?=w128:bool)
    n42 = local read "TASK ENABLE"() -> (w127:bool)
    n43 = And(x=w128, y=w127) -> (x .and. y?=w126:bool)
    n44 = case shown="True" w126 {
      selector: w126 -> [_ w152]
      tunnel: w141 -> [w151 w156]
      tunnel: [w151 w155] -> w138
      tunnel: w137 -> [w150 w154]
      tunnel: [w150 w153] -> w136
      frame False {
      }
      frame True {
        n45 = Generate User Event(user event=w156, event data cluster=w152, error in=w154) -> (user event out=w155:refnum<user-event>, error out=w153:errorcluster)  [unwired: 1 in]
      }
    }
    n46 = case shown="False" "STOP" {
      selector: "STOP" -> [_ w145]
      tunnel: w140 -> [w144 w149]
      tunnel: [w144 w148] -> w139
      tunnel: w135 -> [w143 w147]
      tunnel: [w143 w146] -> w134
      tunnel: [FALSE w145] -> w132
      frame False {
      }
      frame True {
        n47 = Generate User Event(user event=w149, event data cluster=w145, error in=w147) -> (user event out=w148:refnum<user-event>, error out=w146:errorcluster)  [unwired: 1 in]
      }
    }
    n48 = Wait (ms)(milliseconds to wait=u32 10) -> ()  [unwired: 1 out]
    n49 = call "FGV Bool.vi"("Init/Read/Write State"=States_for_Action_Engine."Write", "Input Node"=w132) -> ()  [unwired: 1 in, 2 out]
  }
  n50 = while {
    tunnel: w58 -> [w163]
    tunnel: [w162] -> w57
    tunnel: w45 -> [w160]
    tunnel: [w159] -> w56
    tunnel: w51 -> [w158]
    tunnel: [w157] -> w48
    stop <- w161 stop-if-true
    # "EVENT Handling Loop"
    n51 = event shown="[1] <Start Task>: User Event" {
      selector: w163 -> [_ _ _]
      dyn-events: [_ _ _] -> w162
      timeout: _ -> [_ _ _]
      tunnel: [FALSE FALSE w197] -> w161
      tunnel: w160 -> [w168 w177 w195]
      tunnel: [w167 w176 w196] -> w159
      tunnel: w158 -> [w166 w175 w194]
      tunnel: [w165 w174 w193] -> w157
      event Timeout {
        n52 = event-data() -> ()  [unwired: 1 in, 3 out]
        n53 = Enqueue Element(queue=w168, element=Intruction_Type_Definitions."Start Task 1" ("Enum"), error in (no error)=w166) -> (queue out=w167:refnum<queue>, error out=w165:errorcluster)  [unwired: 1 in, 1 out]
      }
      event User Event {
        n54 = event-data() -> ()  [unwired: 1 in, 5 out]
        n55 = call "Arduino Interfacing VI.vi"("AE Mode"=Arduino_Interfacing."Read From Arduino") -> ("Arduino Data"=w171:T15)  [unwired: 3 in, 1 out]
        n56 = Unbundle By Name(w171) -> ("Rotary Switch"=w170:u8)
        n57 = case shown="11" w170 {
          tunnel: [Intruction_Type_Definitions."Start Task 1" ("Enum") Intruction_Type_Definitions."Start Task 2" ("Enum") Intruction_Type_Definitions."Start Task 3" ("Enum") Intruction_Type_Definitions."Start Task 4" ("Enum") Intruction_Type_Definitions."Start Task 5" ("Enum") Intruction_Type_Definitions."Start Task 6" ("Enum") Intruction_Type_Definitions."Start Task 7" ("Enum") Intruction_Type_Definitions."Start Task 8 - BALL" ("Enum") Intruction_Type_Definitions."Start Task 8 - Soap" ("Enum") Intruction_Type_Definitions."Start Task 8 - Gel" ("Enum") Intruction_Type_Definitions."Start Task 8 - Pipe" ("Enum") Intruction_Type_Definitions."Start Task 9" ("Enum") Intruction_Type_Definitions."None" ("Enum")] -> w173
          frame 0, Default {
          }
          frame 1 {
          }
          frame 2 {
          }
          frame 3 {
          }
          frame 4 {
          }
          frame 5 {
          }
          frame 6 {
          }
          frame 7 {
          }
          frame 8 {
          }
          frame 9 {
          }
          frame 10 {
          }
          frame 11 {
          }
          frame 12 {
          }
        }
        "Selected Task" <- w173
        n58 = Enqueue Element(queue=w177, element=w173, error in (no error)=w175) -> (queue out=w176:refnum<queue>, error out=w174:errorcluster)  [unwired: 1 in, 1 out]
      }
      event User Event {
        n59 = event-data() -> ("Stop Queue"=w197:bool)  [unwired: 1 in, 4 out]
        n60 = Enqueue Element At Opposite End(queue=w195, element=Intruction_Type_Definitions."Exit" ("Enum"), error in (no error)=w194) -> (queue out=w196:refnum<queue>, error out=w193:errorcluster)  [unwired: 1 in, 1 out]
      }
    }
  }
  n61 = while {
    tunnel: w46 -> [w207]
    tunnel: w45 -> [w204]
    stop <- w201 stop-if-true
    # "Status Loop for Action Queues"
    n62 = Get Queue Status(queue=w207, return elements? (F)=TRUE) -> (error out=w203:errorcluster, # elements in queue=→"Action Queue Items":i32, elements=→"Action Queues items":string[])  [unwired: 1 in, 5 out]
    n63 = Get Queue Status(queue=w204, return elements? (F)=TRUE) -> (# pending remove=→"State Logic Queue Items":i32, error out=w202:errorcluster, elements=→"elements":T8[])  [unwired: 1 in, 5 out]
    n64 = Merge Errors(w203, w202) -> (w201:errorcluster)
    n65 = Wait (ms)(milliseconds to wait=u32 500) -> ()  [unwired: 1 out]
  }
  n66 = while {
    tunnel: w45 -> [w251]
    tunnel: w46 -> [w263]
    tunnel: w49 -> [w261]
    tunnel: [w260] -> _
    tunnel: [w259] -> w39
    shift-right: [w252] -> _
    shift-left: T7 {"PING_A"=0, "PING_B"=0, "PING_C"=0, "PING_D"=0} -> [w254]
    shift-right: [w245] -> _
    shift-left: State_Type_Definitions."Startup" ("Enum") -> [w248]
    shift-right: [w241] -> _
    shift-left: T6 {"xDistance"=0.0, "yDistance"=0.0, "wDistance"=0.0} -> [w243]
    shift-right: [w238] -> _
    shift-left: _ -> [w237]
    shift-right: [w234] -> _
    shift-left: T9 {"Recognized Object"=FALSE, "Object X coordinate"=0.0, "Object Y coordinate"=0.0} -> [w236]
    shift-right: [w231] -> _
    shift-left: T5 {"y Stepper Position"=0, "z Stepper Position"=0} -> [w233]
    shift-right: [w228] -> _
    shift-left: T4 {"Yaw"=0.0, "Compass"=0.0} -> [w230]
    shift-right: [w225] -> _
    shift-left: T3 {"Time up flag"=FALSE, "SET TIME TO CHECK"=0.0} -> [w227]
    shift-right: [w223] -> _
    shift-left: T18 {"yStepper desired"=0} -> [w224]
    shift-right: [w219] -> _
    shift-left: T2 {"Left IR Sensor"=0.0, "Arm IR Sensor"=0.0, "Bottom IR Sensor"=0.0} -> [w221]
    shift-right: [w217] -> _
    shift-left: T17 {"ySpeed"=0.0, "xSpeed"=0.0, "wSpeed"=0.0} -> [w218]
    shift-right: [w214] -> _
    shift-left: T1 {"Line Detected?"=FALSE, "S1"=0.0, "S2"=0.0, "S3"=0.0, "S4"=0.0} -> [w216]
    shift-right: [w212] -> _
    shift-left: _ -> [w211]
    stop <- w250 stop-if-true
    # ">>Action Queue>>"
    # ">>State Logic Queue Reference >>"
    # ">>> Line Sensor Cluster>>>"
    # ">>> IR Sensors >>>"
    # ">>> Time cluster >>>"
    # ">>> Object detection >>>"
    # ">>> Yaw >>>"
    # ">>> Ultrasonic Sensors Detect >>>"
    # ">>> Encoders >>>"
    # ">>> Stepper position >>>"
    # ">>State Logic  >>"
    # ">> Item Selection Bias >>"
    # ">> Item Selection Bias >>"
    # ">> Item Selection Bias >>"
    # ">>State Logic  >>"
    # ">>> Motor control cluster >>>"
    # ">>> yStepper command>>>"
    # ">>True Stop Next State >>"
    # ">>Error  >>"
    # ">>Timeout>>"
    # ">>Action states Queue Reference >>"
    # ">>State Logic Queue Reference >>"
    # "TOP LEVEL BASELINE (MAIN PROCESSING LOOP)"
    n67 = Wait (ms)(milliseconds to wait=u32 20) -> ()  [unwired: 1 out]
    n68 = Dequeue Element(queue=w263, timeout in ms (-1)=0, error in (no error)=w261) -> (queue out=w255:refnum<queue>, element=w262:string, error out=w256:errorcluster)  [unwired: 1 out]
    "Action State" <- w262
    n69 = case shown="\"READ IR\"" w262 {
      tunnel: [_ _ _ _ _ _ _ _ _ _ _ _ _ _ _ _ _ _ _ _ 0 w3028 _ _ _ _ _ _ _ _ _ _ _ _ _ _ _ _ _ _ _ _ _ _ _ _ _ _ _ _ _ _ _] -> w258
      tunnel: w255 -> [_ _ _ _ _ _ _ _ _ _ _ _ _ _ _ _ _ _ _ _ _ _ _ _ _ _ _ _ _ _ _ _ _ _ _ _ _ _ _ _ _ _ _ _ _ _ _ _ _ _ _ _ _]
      tunnel: w254 -> [w2724 w2735 w2749 w2762 w2781 w2795 w2808 w2821 w2836 w2850 w2863 w2872 w2889 w2905 w2919 w2931 w2954 w2963 w2992 w3004 w3017 w3029 w3040 w3052 w3069 w3103 w3139 w3152 w3162 w3173 w3185 w3199 w3214 w3225 w3236 w3255 w3265 w3280 w3289 w3301 w3313 w3325 w3334 w3351 w3360 w3378 w3386 w3400 w3414 w3428 w3442 w3456 w3469]
      tunnel: [w2724 w2735 w2749 w2762 w2781 w2795 w2808 w2821 w2836 w2850 w2863 w2872 w2889 w2906 w2919 w2931 w2954 w2963 w2993 w3004 w3017 w3029 w3040 w3052 w3069 w3102 w3138 w3152 w3162 w3173 w3185 w3199 w3214 w3225 w3236 w3255 w3265 w3280 w3289 w3301 w3313 w3325 w3334 w3351 w3360 w3378 w3386 w3400 w3414 w3428 w3442 w3456 w3469] -> w253
      tunnel: [TRUE TRUE _ _ _ _ _ _ _ _ _ _ _ _ _ _ _ _ _ _ _ _ _ _ _ _ _ _ _ _ _ _ _ _ _ _ _ _ _ _ _ _ _ _ _ _ _ _ _ _ _ _ _] -> w250
      tunnel: w248 -> [w2722 w2733 w2748 w2761 w2780 w2794 w2807 w2820 w2835 w2849 w2862 w2871 w2888 w2904 w2918 w2929 w2947 w2962 w2991 w3003 w3014 w3026 w3039 w3051 w3068 w3101 w3137 w3151 w3161 w3172 w3177 w3198 w3213 w3224 w3235 w3254 w3264 w3274 w3288 w3300 w3312 w3324 w3333 w3342 w3359 w3377 w3385 w3399 w3413 w3427 w3441 w3455 w3468]
      tunnel: [_ _ _ _ _ _ _ _ _ _ _ _ _ _ _ _ _ _ _ _ _ TRUE _ _ _ _ _ _ _ _ _ _ _ _ _ _ _ _ _ _ _ _ _ _ _ _ _ _ _ _ _ _ _] -> w247
      tunnel: [w2722 w2733 w2748 w2761 w2780 w2794 w2807 w2820 w2835 w2849 w2862 w2871 w2888 w2904 w2918 w2929 w2947 w2962 w2991 w3003 w3014 w3026 w3039 w3051 w3068 w3101 w3137 w3151 w3161 w3172 w3177 w3198 w3213 w3224 w3235 w3254 w3264 w3274 w3288 w3300 w3312 w3324 w3333 w3342 w3359 w3377 w3385 w3399 w3413 w3427 w3441 w3455 w3468] -> w246
      tunnel: w243 -> [w2721 w2732 w2747 w2764 w2779 w2793 w2806 w2819 w2834 w2848 w2861 w2873 w2887 w2903 w2920 w2933 w2949 w2964 w2990 w3005 w3013 w3025 w3041 w3053 w3064 w3092 w3127 w3150 w3164 w3174 w3182 w3200 w3215 w3226 w3237 w3256 w3267 w3278 w3291 w3303 w3315 w3327 w3336 w3346 w3362 w3380 w3388 w3402 w3416 w3430 w3444 w3458 w3471]
      tunnel: [w2721 w2732 w2747 w2764 w2779 w2793 w2806 w2819 w2834 w2848 w2861 w2873 w2886 w2903 w2920 w2933 w2949 w2964 w2989 w3005 w3013 w3025 w3041 w3053 w3064 w3091 w3126 w3150 w3164 w3174 w3182 w3200 w3215 w3226 w3237 w3256 w3267 w3278 w3291 w3303 w3315 w3327 w3336 w3346 w3362 w3380 w3388 w3402 w3416 w3430 w3444 w3458 w3471] -> w242
      tunnel: w236 -> [w2720 w2731 w2746 w2763 w2778 w2792 w2805 w2818 w2833 w2847 w2859 w2870 w2885 w2902 w2913 w2932 w2948 w2961 w2981 w3002 w3012 w3024 w3038 w3050 w3067 w3096 w3132 w3148 w3163 w3171 w3183 w3197 w3212 w3220 w3234 w3250 w3266 w3279 w3290 w3302 w3314 w3326 w3335 w3345 w3361 w3379 w3387 w3401 w3415 w3429 w3443 w3457 w3470]
      tunnel: [w2720 w2731 w2746 w2763 w2778 w2792 w2805 w2818 w2833 w2847 w2859 w2870 w2885 w2902 w2913 w2932 w2948 w2961 w2980 w3002 w3012 w3024 w3038 w3050 w3066 w3095 w3131 w3148 w3163 w3171 w3183 w3197 w3212 w3220 w3234 w3249 w3266 w3279 w3290 w3302 w3314 w3326 w3335 w3345 w3361 w3379 w3387 w3401 w3415 w3429 w3443 w3457 w3470] -> w235
      tunnel: w233 -> [w2719 w2730 w2745 w2765 w2777 w2791 w2804 w2817 w2832 w2846 w2858 w2869 w2884 w2901 w2921 w2934 w2950 w2960 w2986 w3001 w3011 w3023 w3037 w3049 w3063 w3087 w3122 w3147 w3160 w3170 w3181 w3196 w3211 w3223 w3233 w3257 w3268 w3277 w3287 w3299 w3311 w3323 w3337 w3347 w3363 w3376 w3389 w3403 w3417 w3431 w3445 w3459 w3472]
      tunnel: [w2719 w2730 w2745 w2765 w2777 w2791 w2804 w2817 w2832 w2846 w2858 w2869 w2884 w2901 w2921 w2934 w2950 w2960 w2985 w3001 w3011 w3023 w3037 w3049 w3063 w3086 w3121 w3147 w3160 w3170 w3181 w3196 w3211 w3223 w3233 w3257 w3268 w3277 w3287 w3299 w3311 w3323 w3337 w3347 w3363 w3375 w3389 w3403 w3417 w3431 w3445 w3459 w3472] -> w232
      tunnel: w230 -> [w2718 w2729 w2743 w2766 w2775 w2789 w2802 w2816 w2830 w2844 w2857 w2868 w2883 w2894 w2916 w2935 w2951 w2959 w2976 w3000 w3010 w3022 w3036 w3048 w3062 w3083 w3118 w3146 w3157 w3169 w3180 w3195 w3210 w3222 w3232 w3258 w3269 w3276 w3286 w3296 w3308 w3320 w3338 w3348 w3364 w3370 w3390 w3404 w3418 w3432 w3446 w3460 w3473]
      tunnel: [w2718 w2729 w2743 w2766 w2775 w2789 w2802 w2816 w2830 w2844 w2857 w2868 w2883 w2894 w2915 w2935 w2951 w2959 w2975 w3000 w3010 w3022 w3036 w3048 w3062 w3082 w3117 w3146 w3157 w3169 w3180 w3195 w3210 w3222 w3232 w3258 w3269 w3276 w3286 w3296 w3308 w3320 w3338 w3348 w3364 w3370 w3390 w3404 w3418 w3432 w3446 w3460 w3473] -> w229
      tunnel: w227 -> [w2716 w2728 w2744 w2767 w2776 w2790 w2803 w2815 w2831 w2845 w2856 w2867 w2882 w2893 w2912 w2936 w2952 w2958 w2972 w2997 w3009 w3021 w3035 w3047 w3061 w3080 w3115 w3144 w3156 w3168 w3179 w3194 w3209 w3221 w3231 w3259 w3270 w3275 w3285 w3295 w3307 w3319 w3339 w3349 w3365 w3369 w3384 w3398 w3412 w3426 w3440 w3454 w3467]
      tunnel: [w2716 w2728 w2744 w2767 w2776 w2790 w2803 w2815 w2831 w2845 w2856 w2867 w2882 w2893 w2912 w2936 w2952 w2958 w2972 w2997 w3009 w3021 w3035 w3047 w3060 w3079 w3114 w3144 w3156 w3168 w3179 w3194 w3209 w3221 w3231 w3259 w3270 w3275 w3285 w3295 w3307 w3319 w3339 w3349 w3365 w3369 w3384 w3396 w3410 w3424 w3438 w3452 w3466] -> w226
      tunnel: w224 -> [_ _ _ _ _ _ _ _ _ _ _ _ _ _ _ _ _ _ _ _ _ _ _ _ _ _ _ _ _ _ _ _ _ _ _ _ _ _ _ _ _ _ _ _ w3356 _ _ _ _ _ _ _ _]
      tunnel: [w2715 w2727 w2738 w2757 w2770 w2784 w2798 w2811 w2826 w2839 w2853 w2866 w2876 w2892 w2909 w2927 w2953 w2957 w2969 w2996 w3008 w3020 w3034 w3044 w3054 w3073 w3106 w3143 w3155 w3167 w3184 w3188 w3203 w3218 w3229 w3243 w3262 w3281 w3284 w3294 w3306 w3318 w3330 w3350 w3354 w3368 w3383 w3393 w3407 w3421 w3435 w3449 w3463] -> w220
      tunnel: w221 -> [w2715 w2727 w2738 w2757 w2770 w2784 w2798 w2811 w2826 w2839 w2853 w2866 w2876 w2892 w2909 w2928 w2953 w2957 w2969 w2996 w3008 w3020 w3034 w3044 w3054 w3074 w3107 w3143 w3155 w3167 w3184 w3188 w3203 w3218 w3229 w3243 w3262 w3281 w3284 w3294 w3306 w3318 w3330 w3350 w3354 w3368 w3383 w3393 w3407 w3421 w3435 w3449 w3463]
      tunnel: w218 -> [_ _ _ _ _ _ _ _ w2825 _ _ _ _ _ _ _ _ _ _ _ _ _ _ _ _ _ _ _ _ _ _ _ _ _ _ _ _ _ _ _ _ _ _ _ _ _ _ _ _ _ _ _ _]
      tunnel: w216 -> [w2714 w2726 w2737 w2751 w2769 w2783 w2797 w2810 w2823 w2838 w2852 w2865 w2875 w2891 w2908 w2923 w2946 w2956 w2967 w2995 w3007 w3019 w3033 w3043 w3057 w3076 w3110 w3142 w3154 w3166 w3176 w3187 w3202 w3217 w3228 w3240 w3261 w3272 w3283 w3293 w3305 w3317 w3329 w3341 w3353 w3367 w3382 w3392 w3406 w3420 w3434 w3448 w3462]
      tunnel: [w2714 w2726 w2737 w2751 w2769 w2783 w2797 w2810 w2823 w2838 w2852 w2865 w2875 w2891 w2908 w2923 w2945 w2956 w2967 w2995 w3007 w3019 w3033 w3043 w3056 w3075 w3109 w3142 w3154 w3166 w3176 w3187 w3202 w3217 w3228 w3240 w3261 w3272 w3283 w3293 w3305 w3317 w3329 w3341 w3353 w3367 w3382 w3392 w3406 w3420 w3434 w3448 w3462] -> w215
      tunnel: [_ _ _ _ _ _ _ _ _ _ _ _ _ _ _ _ _ _ _ _ _ _ _ _ _ _ _ _ _ _ _ _ _ _ _ w3239 _ _ _ _ _ _ _ _ _ _ _ _ _ _ _ _ _] -> w213
      tunnel: w211 -> [w2713 w2725 w2736 w2750 w2768 w2782 w2796 w2809 w2822 w2837 w2851 w2864 w2874 w2890 w2907 w2922 w2937 w2955 w2965 w2994 w3006 w3018 w3032 w3042 w3058 w3077 w3111 w3141 w3153 w3165 w3175 w3186 w3201 w3216 w3227 w3238 w3260 w3271 w3282 w3292 w3304 w3316 w3328 w3340 w3352 w3366 w3381 w3391 w3405 w3419 w3433 w3447 w3461]
      tunnel: [w2713 w2725 w2736 w2750 w2768 w2782 w2796 w2809 w2822 w2837 w2851 w2864 w2874 w2890 w2907 w2922 w2937 w2955 w2965 w2994 w3006 w3018 w3032 w3042 w3058 w3077 w3111 w3141 w3153 w3165 w3175 w3186 w3201 w3216 w3227 w3238 w3260 w3271 w3282 w3292 w3304 w3316 w3328 w3340 w3352 w3366 w3381 w3391 w3405 w3419 w3433 w3447 w3461] -> w210
      frame "Exit" {
        # ">>State Logic  >>"
        # ">>> Time cluster >>>"
        # ">>> Yaw >>>"
        # ">>> Stepper position >>>"
        # ">>> Encoders >>>"
        # ">>> Object detection >>>"
        # ">>> Ultrasonic Sensors Detect >>>"
        n70 = call "Imaq Dispose"("All Images? (No)"=TRUE) -> ()  [unwired: 5 in, 1 out]
      }
      frame "----Movement States----" {
        # ">>State Logic  >>"
        # ">>> Time cluster >>>"
        # ">>> Yaw >>>"
        # ">>> Stepper position >>>"
        # ">>> Encoders >>>"
        # ">>> Object detection >>>"
        # ">>> Ultrasonic Sensors Detect >>>"
      }
      frame "FORWARD" {
        # ">>State Logic  >>"
        # ">>> Time cluster >>>"
        # ">>> Yaw >>>"
        # ">>> Stepper position >>>"
        # ">>> Encoders >>>"
        # ">>> Object detection >>>"
        # ">>> Ultrasonic Sensors Detect >>>"
        n71 = Unbundle By Name(w2743) -> ("Yaw"=w2739:dbl)
        n72 = call "MOTOR CONTROL WITH PID AE.vi"("Yaw"=w2739, "Speed"=30.0, "Direction"=MOTOR_CONTROL_WITH_PID_AE_DIRECTION_TYPE_DEF."y-axis movement", "AE Mode"=MOTOR_CONTROL_WITH_PID_AE_DATA_MODE_TYPE_DEF."Write to AE") -> ()  [unwired: 1 out]
      }
      frame "FORWARD - IR ASSIST" {
        # ">>State Logic  >>"
        # ">>> Time cluster >>>"
        # ">>> Yaw >>>"
        # ">>> Stepper position >>>"
        # ">>> Encoders >>>"
        # ">>> Object detection >>>"
        # ">>> Ultrasonic Sensors Detect >>>"
        n73 = Unbundle By Name(w2757) -> ("Left IR Sensor"=w2756:dbl)
        n74 = Subtract(x=w2756, y=20.0) -> (x-y=w2754:dbl)
        n75 = Multiply(x=w2754, y=0.25) -> (x*y=w2752:dbl)
        n76 = call "MOTOR CONTROL WITH PID AE.vi"("Yaw"=w2752, "Speed"=30.0, "Direction"=MOTOR_CONTROL_WITH_PID_AE_DIRECTION_TYPE_DEF."y-axis movement", "AE Mode"=MOTOR_CONTROL_WITH_PID_AE_DATA_MODE_TYPE_DEF."Write to AE") -> ()  [unwired: 1 out]
      }
      frame "LEFT" {
        # ">>State Logic  >>"
        # ">>> Time cluster >>>"
        # ">>> Yaw >>>"
        # ">>> Stepper position >>>"
        # ">>> Encoders >>>"
        # ">>> Object detection >>>"
        # ">>> Ultrasonic Sensors Detect >>>"
        n77 = Unbundle By Name(w2775) -> ("Yaw"=w2772:dbl)
        n78 = call "MOTOR CONTROL WITH PID AE.vi"("Yaw"=w2772, "Speed"=-20.0, "Direction"=MOTOR_CONTROL_WITH_PID_AE_DIRECTION_TYPE_DEF."x-axis movement", "AE Mode"=MOTOR_CONTROL_WITH_PID_AE_DATA_MODE_TYPE_DEF."Write to AE") -> ()  [unwired: 1 out]
      }
      frame "RIGHT" {
        # ">>> Time cluster >>>"
        # ">>> Yaw >>>"
        # ">>> Stepper position >>>"
        # ">>> Encoders >>>"
        # ">>> Object detection >>>"
        # ">>> Ultrasonic Sensors Detect >>>"
        n79 = Unbundle By Name(w2789) -> ("Yaw"=w2785:dbl)
        n80 = call "MOTOR CONTROL WITH PID AE.vi"("Yaw"=w2785, "Speed"=20.0, "Direction"=MOTOR_CONTROL_WITH_PID_AE_DIRECTION_TYPE_DEF."x-axis movement", "AE Mode"=MOTOR_CONTROL_WITH_PID_AE_DATA_MODE_TYPE_DEF."Write to AE") -> ()  [unwired: 1 out]
      }
      frame "R-ACW" {
        # ">>> IR Sensors >>>"
        # ">>> Time cluster >>>"
        # ">>> Yaw >>>"
        # ">>> Stepper position >>>"
        # ">>> Encoders >>>"
        # ">>> Object detection >>>"
        # ">>> Ultrasonic Sensors Detect >>>"
        n81 = call "MOTOR CONTROL WITH PID AE.vi"("Speed"=10.0, "Direction"=MOTOR_CONTROL_WITH_PID_AE_DIRECTION_TYPE_DEF."rotation", "AE Mode"=MOTOR_CONTROL_WITH_PID_AE_DATA_MODE_TYPE_DEF."Write to AE") -> ()  [unwired: 1 in, 1 out]
      }
      frame "R-CW" {
        (unwired) -0.2 ("Speed")
        # ">>> Time cluster >>>"
        # ">>> Yaw >>>"
        # ">>> Stepper position >>>"
        # ">>> Encoders >>>"
        # ">>> Object detection >>>"
        # ">>> Ultrasonic Sensors Detect >>>"
        n82 = call "MOTOR CONTROL WITH PID AE.vi"("Speed"=-10.0, "Direction"=MOTOR_CONTROL_WITH_PID_AE_DIRECTION_TYPE_DEF."rotation", "AE Mode"=MOTOR_CONTROL_WITH_PID_AE_DATA_MODE_TYPE_DEF."Write to AE") -> ()  [unwired: 1 in, 1 out]
      }
      frame "X AXIS - SLOW" {
        # ">>> Line Sensor Cluster>>>"
        # ">>> IR Sensors >>>"
        # ">>> Time cluster >>>"
        # ">>> Yaw >>>"
        # ">>> Stepper position >>>"
        # ">>> Encoders >>>"
        # ">>> Object detection >>>"
        # ">>> Ultrasonic Sensors Detect >>>"
        n83 = Unbundle By Name(w2825) -> ("xSpeed"=w2824:dbl)
        n84 = Unbundle By Name(w2830) -> ("Yaw"=w2827:dbl)
        n85 = call "MOTOR CONTROL WITH PID AE.vi"("Yaw"=w2827, "Speed"=w2824, "Direction"=MOTOR_CONTROL_WITH_PID_AE_DIRECTION_TYPE_DEF."x-axis movement", "AE Mode"=MOTOR_CONTROL_WITH_PID_AE_DATA_MODE_TYPE_DEF."Write to AE") -> ()  [unwired: 1 out]
      }
      frame "REVERSE" {
        # ">>> Time cluster >>>"
        # ">>> Yaw >>>"
        # ">>> Stepper position >>>"
        # ">>> Encoders >>>"
        # ">>> Object detection >>>"
        # ">>> Ultrasonic Sensors Detect >>>"
        n86 = Unbundle By Name(w2844) -> ("Yaw"=w2840:dbl)
        n87 = call "MOTOR CONTROL WITH PID AE.vi"("Yaw"=w2840, "Speed"=-50.0, "Direction"=MOTOR_CONTROL_WITH_PID_AE_DIRECTION_TYPE_DEF."y-axis movement", "AE Mode"=MOTOR_CONTROL_WITH_PID_AE_DATA_MODE_TYPE_DEF."Write to AE") -> ()  [unwired: 1 out]
      }
      frame "STOP" {
        n88 = Wait (ms)(milliseconds to wait=u32 100) -> ()  [unwired: 1 out]
        n89 = call "MOTOR CONTROL WITH PID AE.vi"("Direction"=MOTOR_CONTROL_WITH_PID_AE_DIRECTION_TYPE_DEF."stop", "AE Mode"=MOTOR_CONTROL_WITH_PID_AE_DATA_MODE_TYPE_DEF."Write to AE") -> ()  [unwired: 2 in, 1 out]
      }
      frame "----SENSOR READING---- " {
      }
      frame "READ ENCODERS" {
        # ">>> Time cluster >>>"
        # ">>> Yaw >>>"
        # ">>> Stepper position >>>"
        # ">>> Object detection >>>"
        # ">>> Current encoder distance >>>"
        # ">>> Ultrasonic Sensors Detect >>>"
        n90 = call "MOTOR CONTROL WITH PID AE.vi"("AE Mode"=MOTOR_CONTROL_WITH_PID_AE_DATA_MODE_TYPE_DEF."Read from AE") -> ("Speed & distance"=w2880:T13)  [unwired: 3 in]
        n91 = Unbundle By Name(w2880) -> ("xDistance"=w2879:dbl, "yDistance"=w2878:dbl, "wDistance"=w2877:dbl)
        n92 = Bundle By Name(cluster=w2887, "xDistance"=w2879, "yDistance"=w2878, "wDistance"=w2877) -> (w2886:T6)
      }
      frame "READ ULTRASONIC" {
        (unwired) navX_type_def."Read Values" ("Mode")
        (unwired) MOTOR_CONTROL_NO_PID_Type_Def."Latch" ("Direction")
        # ">>> Line Sensor Cluster>>>"
        # ">>> IR Sensors >>>"
        # ">>State Logic  >>"
        # ">>> Time cluster >>>"
        # ">>> Ultrasonic Sensors Detect >>>"
        # ">>> Object detection >>>"
        # ">>> Encoders >>>"
        # ">>> Stepper position >>>"
        # ">>> Yaw >>>"
        n93 = call "Arduino Interfacing VI.vi"("AE Mode"=Arduino_Interfacing."Read From Arduino") -> ("Arduino Data"=w2899:T15)  [unwired: 3 in, 1 out]
        n94 = Unbundle By Name(w2899) -> ("PING A"=w2898:u8, "PING B"=w2897:u8, "PING C"=w2896:u8, "PING D"=w2895:u8)
        n95 = Bundle By Name(cluster=w2905, "PING_A"=w2898, "PING_B"=w2897, "PING_C"=w2896, "PING_D"=w2895) -> (w2906:T7)
      }
      frame "READ NAVX" {
        # ">> Item Selection Bias >>"
        # ">>State Logic  >>"
        # ">>> Line Sensor Cluster>>>"
        # ">>> IR Sensors >>>"
        # ">>> Time cluster >>>"
        # ">>> Yaw >>>"
        # ">>> Ultrasonic Sensors Detect >>>"
        # ">>> Object detection >>>"
        # ">>> Encoders >>>"
        # ">>> Stepper position >>>"
        n96 = call "navX reading VI.vi"("Mode"=navX_type_def."Read Values") -> ("NavX Readings"=w2911:T14)  [unwired: 2 in, 3 out]
        n97 = Unbundle By Name(w2911) -> ("Heading"=w2910:dbl)
        n98 = Unbundle By Name(w2911) -> ("Yaw"=w2914:dbl)
        n99 = Bundle By Name(cluster=w2916, "Yaw"=w2914, "Compass"=w2910) -> (w2915:T4)
      }
      frame "READ IR" {
        w2925 = T38 [enum."B/AI1"] items=["Not Connected", "AudioIn/Left", "AudioIn/Right", "C/AI0", "C/AI1", "A/AI0", "A/AI1", "A/AI2", "A/AI3", "A/AI4", "A/AI5", "A/AI6", "A/AI7", "B/AI0", "B/AI1", "B/AI2", "B/AI3", "B/AI4", "B/AI5", "B/AI6", "B/AI7", "AI/AI0", "AI/AI1", "AI/AI2", "AI/AI3", "A/AI0 (DIFF)", "A/AI1 (DIFF)", "A/AI2 (DIFF)", "A/AI3 (DIFF)", "B/AI0 (DIFF)", "B/AI1 (DIFF)", "B/AI2 (DIFF)", "B/AI3 (DIFF)"] ("AI Channel")
        w2930 = T38 [enum."B/AI0"] items=["Not Connected", "AudioIn/Left", "AudioIn/Right", "C/AI0", "C/AI1", "A/AI0", "A/AI1", "A/AI2", "A/AI3", "A/AI4", "A/AI5", "A/AI6", "A/AI7", "B/AI0", "B/AI1", "B/AI2", "B/AI3", "B/AI4", "B/AI5", "B/AI6", "B/AI7", "AI/AI0", "AI/AI1", "AI/AI2", "AI/AI3", "A/AI0 (DIFF)", "A/AI1 (DIFF)", "A/AI2 (DIFF)", "A/AI3 (DIFF)", "B/AI0 (DIFF)", "B/AI1 (DIFF)", "B/AI2 (DIFF)", "B/AI3 (DIFF)"] ("AI Channel")
        # ">>State Logic  >>"
        # ">>> Time cluster >>>"
        # ">>> Ultrasonic Sensors Detect >>>"
        # ">>> Object detection >>>"
        # ">>> Encoders >>>"
        # ">>> Stepper position >>>"
        # ">>> Yaw >>>"
        n100 = call <vilib>:"Sharp IR.vi"("AI Channel"=w2925) -> ("Sharp IR Distance"=w2924:dbl)  [unwired: 8 in, 2 out]
        n101 = call <vilib>:"Sharp IR.vi"("AI Channel"=w2930) -> ("Sharp IR Distance"=w2926:dbl)  [unwired: 8 in, 2 out]
        n102 = Bundle By Name(cluster=w2928, "Left IR Sensor"=w2926, "Arm IR Sensor"=w2924) -> (w2927:T2)
      }
      frame "READ LINE SENSOR" {
        # ">>> IR Sensors >>>"
        # ">>> Line Sensor Cluster>>>"
        # ">>State Logic  >>"
        # ">>> Time cluster >>>"
        # ">>> Object detection >>>"
        # ">>> Yaw >>>"
        # ">>> Ultrasonic Sensors Detect >>>"
        # ">>> Encoders >>>"
        # ">>> Stepper position >>>"
        n103 = call "Line Sensor AE.vi"("AE State"=Line_Sensor_AE_Type_Def."READ FROM LINE SENSORS") -> ("Line Detected?"=w2943:bool, "Line Sensor Raw Values"=w2942:T40)
        n104 = Unbundle By Name(w2942) -> ("S1"=w2941:dbl, "S2"=w2940:dbl, "S3"=w2939:dbl, "S4"=w2938:dbl)
        n105 = Bundle By Name(cluster=w2946, "Line Detected?"=w2943, "S1"=w2941, "S2"=w2940, "S3"=w2939, "S4"=w2938) -> (w2945:T1)
      }
      frame "----SYSTEM MODES----" {
        (unwired) I2C_MASTER_Type_Def."Last State" ("Arduino Mode")
        # ">>> Object detection >>>"
        # ">>> Yaw >>>"
        # ">>> Ultrasonic Sensors Detect >>>"
        # ">>> Encoders >>>"
        # ">>> Stepper position >>>"
      }
      frame "INIT" {
        w2987 = u8 0
        w2988 = 0.0
        # ">>> IR Sensors >>>"
        # ">>> IR Sensors >>>"
        # ">>> Line Sensor Cluster>>>"
        # ">>> Time cluster >>>"
        # ">>> Object detection >>>"
        # ">>> Yaw >>>"
        # ">>> Ultrasonic Sensors Detect >>>"
        # ">>> Encoders >>>"
        # ">>> Stepper position >>>"
        # ">>State Logic  >>"
        n106 = call "Arduino Interfacing VI.vi"("AE Mode"=Arduino_Interfacing."Initialize") -> ()  [unwired: 3 in, 2 out]
        n107 = call "FGV Bool.vi"("Init/Read/Write State"=States_for_Action_Engine."Initialize") -> ()  [unwired: 2 in, 2 out]
        n108 = call "Elasped Timer.vi"("Action"=Elapsed_timer_control."Initialize") -> ()  [unwired: 7 in, 4 out]
        n109 = call "MOTOR CONTROL WITH PID AE.vi"("AE Mode"=MOTOR_CONTROL_WITH_PID_AE_DATA_MODE_TYPE_DEF."Init AE") -> ()  [unwired: 3 in, 1 out]
        n110 = call "IMAQ Reference AE.vi"("IMAQ AE States"=IMAQ_Reference_AE."Initialize AE") -> ()  [unwired: 1 in, 2 out]
        n111 = call "Line Sensor AE.vi"("AE State"=Line_Sensor_AE_Type_Def."INIT AE") -> ()  [unwired: 2 out]
        n112 = Bundle By Name(cluster=w2981, "Recognized Object"=FALSE, "Object X coordinate"=0.0, "Object Y coordinate"=0.0) -> (w2980:T9)
        n113 = Bundle By Name(cluster=w2986, "y Stepper Position"=u8 0, "z Stepper Position"=u8 0) -> (w2985:T5)
        n114 = Bundle By Name(cluster=w2990, "xDistance"=w2988, "yDistance"=w2988, "wDistance"=w2988) -> (w2989:T6)
        n115 = Bundle By Name(cluster=w2992, "PING_A"=w2987, "PING_B"=w2987, "PING_C"=w2987, "PING_D"=w2987) -> (w2993:T7)
        n116 = Bundle By Name(cluster=w2976, "Yaw"=0.0) -> (w2975:T4)
      }
      frame "ARDUINO - ULTRASONIC" {
        # ">>> Time cluster >>>"
        # ">>> Line Sensor Cluster>>>"
        # ">>> Object detection >>>"
        # ">>> Yaw >>>"
        # ">>> Ultrasonic Sensors Detect >>>"
        # ">>> Encoders >>>"
        # ">>> Stepper position >>>"
        # ">>State Logic  >>"
        n117 = call "Arduino Interfacing VI.vi"("Data to Write"=I2C_MASTER_WRITE_NEW_Type_Def."Ultrasonic sensors", "AE Mode"=Arduino_Interfacing."Write to Arduino") -> ()  [unwired: 2 in, 2 out]
      }
      frame "NAVX CALIBRATE" {
        # ">>> Object detection >>>"
        # ">>> Yaw >>>"
        # ">>> Ultrasonic Sensors Detect >>>"
        # ">>> Encoders >>>"
        # ">>> Stepper position >>>"
        # ">>State Logic  >>"
        # "Adds a 15 second delay to the startup process \nfor the NavX to calibrate"
        n118 = Wait (ms)(milliseconds to wait=u32 1000) -> ()  [unwired: 1 out]
      }
      frame "NO ACTION", Default {
        (unwired) u8 0 ("y Stepper value")
        (unwired) TRUE ("Latch")
        (unwired) navX_type_def."Read Values" ("Mode")
        (unwired) MOTOR_CONTROL_NO_PID_Type_Def."Latch" ("Direction")
        # ">>> Object detection >>>"
        # ">>> Yaw >>>"
        # ">>> Ultrasonic Sensors Detect >>>"
        # ">>> Encoders >>>"
        # ">>> Stepper position >>>"
        # ">>State Logic  >>"
        n119 = case shown="4" w3026 {
          tunnel: [0 100] -> w3028
          frame 1, Default {
          }
          frame 4 {
          }
        }
      }
      frame "----RESET CASES----" {
        (unwired) I2C_MASTER_Type_Def."Last State" ("Arduino Mode")
        # ">>> Object detection >>>"
        # ">>> Yaw >>>"
        # ">>> Ultrasonic Sensors Detect >>>"
        # ">>> Encoders >>>"
        # ">>> Stepper position >>>"
        # ">>State Logic  >>"
      }
      frame "RESET ENCODERS" {
        # ">>> Object detection >>>"
        # ">>> Yaw >>>"
        # ">>> Ultrasonic Sensors Detect >>>"
        # ">>> Encoders >>>"
        # ">>> Stepper position >>>"
        # ">>State Logic  >>"
        n120 = call "MOTOR CONTROL WITH PID AE.vi"("Direction"=MOTOR_CONTROL_WITH_PID_AE_DIRECTION_TYPE_DEF."reset encoders", "AE Mode"=MOTOR_CONTROL_WITH_PID_AE_DATA_MODE_TYPE_DEF."Write to AE") -> ()  [unwired: 2 in, 1 out]
      }
      frame "RESET FLAGS" {
        # ">>> Line Sensor Cluster>>>"
        # ">>> IR Sensors >>>"
        # ">>> Time cluster >>>"
        # ">>> Object detection >>>"
        # ">>> Yaw >>>"
        # ">>> Ultrasonic Sensors Detect >>>"
        # ">>> Encoders >>>"
        # ">>> Stepper position >>>"
        # ">>> Line Sensor Cluster>>>"
        # ">>> IR Sensors >>>"
        # ">>> Time cluster >>>"
        # ">>> Object detection >>>"
        # ">>> Yaw >>>"
        # ">>> Ultrasonic Sensors Detect >>>"
        # ">>> Encoders >>>"
        # ">>> Stepper position >>>"
        # "Resets BOOLEAN FLAGS only"
        n121 = Wait (ms)(milliseconds to wait=u32 20) -> ()  [unwired: 1 out]
        n122 = Bundle By Name(cluster=w3067, "Recognized Object"=FALSE) -> (w3066:T9)
        n123 = Bundle By Name(cluster=w3057, "Line Detected?"=FALSE) -> (w3056:T1)
        n124 = Bundle By Name(cluster=w3061, "Time up flag"=FALSE) -> (w3060:T3)
      }
      frame "RESET SENSOR VALUES" {
        w3071 = 0.0 ("S4")
        w3072 = 0.0 ("S4")
        # "Resets SENSOR VALUES only"
        # ">>> Line Sensor Cluster>>>"
        # ">>> IR Sensors >>>"
        # ">>> Time cluster >>>"
        # ">>> Object detection >>>"
        # ">>> Yaw >>>"
        # ">>> Ultrasonic Sensors Detect >>>"
        # ">>> Encoders >>>"
        # ">>> Stepper position >>>"
        # ">>> Line Sensor Cluster>>>"
        # ">>> IR Sensors >>>"
        # ">>> Time cluster >>>"
        # ">>> Object detection >>>"
        # ">>> Yaw >>>"
        # ">>> Ultrasonic Sensors Detect >>>"
        # ">>> Encoders >>>"
        # ">>> Stepper position >>>"
        # "Resets any software variables\nand/or non-critical states"
        n125 = Wait (ms)(milliseconds to wait=u32 20) -> ()  [unwired: 1 out]
        n126 = Bundle By Name(cluster=w3080, "SET TIME TO CHECK"=0.0) -> (w3079:T3)
        n127 = Bundle By Name(cluster=w3096, "Object X coordinate"=0.0, "Object Y coordinate"=0.0) -> (w3095:T9)
        n128 = Bundle By Name(cluster=w3087, "y Stepper Position"=u8 0, "z Stepper Position"=u8 0) -> (w3086:T5)
        n129 = Bundle By Name(cluster=w3074, "Left IR Sensor"=w3071, "Arm IR Sensor"=w3071) -> (w3073:T2)
        n130 = Bundle By Name(cluster=w3092, "xDistance"=0.0, "yDistance"=0.0, "wDistance"=0.0) -> (w3091:T6)
        n131 = Bundle By Name(cluster=w3103, "PING_A"=u8 0, "PING_B"=u8 0, "PING_C"=u8 0, "PING_D"=u8 0) -> (w3102:T7)
        n132 = Bundle By Name(cluster=w3083, "Yaw"=0.0) -> (w3082:T4)
        n133 = Bundle By Name(cluster=w3076, "S1"=w3072, "S2"=w3072, "S3"=w3072, "S4"=w3072) -> (w3075:T1)
      }
      frame "RESET ALL SENSORS" {
        w3105 = 0.0 ("SET TIME TO CHECK")
        # ">>> Line Sensor Cluster>>>"
        # ">>> IR Sensors >>>"
        # ">>> Time cluster >>>"
        # ">>> Object detection >>>"
        # ">>> Yaw >>>"
        # ">>> Ultrasonic Sensors Detect >>>"
        # ">>> Encoders >>>"
        # ">>> Stepper position >>>"
        # ">>> Line Sensor Cluster>>>"
        # ">>> IR Sensors >>>"
        # ">>> Time cluster >>>"
        # ">>> Object detection >>>"
        # ">>> Yaw >>>"
        # ">>> Ultrasonic Sensors Detect >>>"
        # ">>> Encoders >>>"
        # ">>> Stepper position >>>"
        # "Resets ALL SENSOR PARAMTERS"
        n134 = Wait (ms)(milliseconds to wait=u32 20) -> ()  [unwired: 1 out]
        n135 = Bundle By Name(cluster=w3115, "Time up flag"=FALSE, "SET TIME TO CHECK"=0.0) -> (w3114:T3)
        n136 = Bundle By Name(cluster=w3132, "Recognized Object"=FALSE, "Object X coordinate"=0.0, "Object Y coordinate"=0.0) -> (w3131:T9)
        n137 = Bundle By Name(cluster=w3122, "y Stepper Position"=u8 0, "z Stepper Position"=u8 0) -> (w3121:T5)
        n138 = Bundle By Name(cluster=w3110, "Line Detected?"=FALSE) -> (w3109:T1)
        n139 = Bundle By Name(cluster=w3107, "Left IR Sensor"=w3105, "Arm IR Sensor"=w3105) -> (w3106:T2)
        n140 = Bundle By Name(cluster=w3127, "xDistance"=0.0, "yDistance"=0.0, "wDistance"=0.0) -> (w3126:T6)
        n141 = Bundle By Name(cluster=w3139, "PING_A"=u8 0, "PING_B"=u8 0, "PING_C"=u8 0, "PING_D"=u8 0) -> (w3138:T7)
        n142 = Bundle By Name(cluster=w3118, "Yaw"=0.0) -> (w3117:T4)
      }
      frame "RESET YAW" {
        n143 = Wait (ms)(milliseconds to wait=u32 100) -> ()  [unwired: 1 out]
        n144 = call "navX reading VI.vi"("Mode"=navX_type_def."Zero Yaw") -> ()  [unwired: 2 in, 4 out]
      }
      frame "RESET ARM" {
        n145 = call "Arduino Interfacing VI.vi"("Data to Write"=I2C_MASTER_WRITE_NEW_Type_Def."Soft Reset", "AE Mode"=Arduino_Interfacing."Write to Arduino") -> ()  [unwired: 2 in, 2 out]
      }
      frame "--------CAM STATES-------" {
      }
      frame "OPEN IMAQ REF" {
        # ">>> Line Sensor Cluster>>>"
        # ">>State Logic  >>"
        # ">>> Time cluster >>>"
        # ">>> Object detection >>>"
        # ">>> Yaw >>>"
        # ">>> Ultrasonic Sensors Detect >>>"
        # ">>> Encoders >>>"
        # ">>> Stepper position >>>"
        # ">>> IR Sensors >>>"
        n146 = call "IMAQ Reference AE.vi"("IMAQ AE States"=IMAQ_Reference_AE."Initialize AE") -> ()  [unwired: 1 in, 2 out]
      }
      frame "OPEN LOG CAM" {
        n147 = call "Webcam AE.vi"("Session In"=T36 "cam0", "Camera states"=Webcam_AE."Initialize Camera") -> ("error out"=w3191:errorcluster, "Session Out"=w3190:T36)  [unwired: 1 in, 1 out]
        n148 = call "Webcam AE.vi"("error in (no error)"=w3191, "Session In"=w3190, "Camera states"=Webcam_AE."Open Camera") -> ()  [unwired: 3 out]
      }
      frame "OPEN LIFE CAM" {
        n149 = call "Webcam AE.vi"("Session In"=T36 "cam1", "Camera states"=Webcam_AE."Initialize Camera") -> ("error out"=w3206:errorcluster, "Session Out"=w3205:T36)  [unwired: 1 in, 1 out]
        n150 = call "Webcam AE.vi"("error in (no error)"=w3206, "Session In"=w3205, "Camera states"=Webcam_AE."Open Camera") -> ()  [unwired: 3 out]
      }
      frame "CAM ACQ" {
        # ">>State Logic  >>"
        # ">>> Time cluster >>>"
        # ">>> Yaw >>>"
        # ">>> Stepper position >>>"
        # ">>> Encoders >>>"
        # ">>> Object detection >>>"
        # ">>> Ultrasonic Sensors Detect >>>"
        n151 = call "Webcam AE.vi"("Camera states"=Webcam_AE."Continuous Acquisition") -> ()  [unwired: 2 in, 3 out]
      }
      frame "CAM CLOSE" {
        # ">>State Logic  >>"
        # ">>> Time cluster >>>"
        # ">>> Yaw >>>"
        # ">>> Stepper position >>>"
        # ">>> Encoders >>>"
        # ">>> Object detection >>>"
        # ">>> Ultrasonic Sensors Detect >>>"
        n152 = call "Webcam AE.vi"("Camera states"=Webcam_AE."Close Camera") -> ()  [unwired: 2 in, 3 out]
      }
      frame "PROCESS IMAGE" {
        # ">>> Line Sensor Cluster>>>"
        # ">>> IR Sensors >>>"
        # ">> Item Selection Bias >>"
        # ">> Item Selection Bias >>"
        # ">>State Logic  >>"
        # ">>> Time cluster >>>"
        # ">>> Yaw >>>"
        # ">>> Stepper position >>>"
        # ">>> Encoders >>>"
        # ">>> Object detection >>>"
        # ">>> Ultrasonic Sensors Detect >>>"
        n153 = call "Webcam AE.vi"("Camera states"=Webcam_AE."Retrieve Image") -> ("error out"=w3251:errorcluster, "Image Out"=w3252:T42)  [unwired: 2 in, 1 out]
        n154 = call "IMAQ Reference AE.vi"("IMAQ AE States"=IMAQ_Reference_AE."Get IMAQ Reference") -> ("Image Out"=w3241:T42)  [unwired: 1 in, 1 out]
        n155 = call "Object Detection SubVI.vi"("Error In"=w3251, "Mode"=w3238, "Image Dest"=w3241, "Image in"=w3252) -> ("Error out"=w3239:errorcluster, "Object Center Coordinates"=w3248:cluster{"x":sgl, "y":sgl}, "Object detection cluster"=w3244:T43)  [unwired: 1 out]
        n156 = Unbundle By Name(w3244) -> ("Object detected?"=w3245:bool)
        n157 = Unbundle By Name(w3248) -> ("x"=w3247:sgl, "y"=w3246:sgl)
        n158 = Bundle By Name(cluster=w3250, "Recognized Object"=w3245, "Object X coordinate"=w3247, "Object Y coordinate"=w3246) -> (w3249:T9)
      }
      frame "DISPOSE CAM BUFFERS" {
        # ">> Item Selection Bias >>"
        # ">>> Line Sensor Cluster>>>"
        # ">>> IR Sensors >>>"
        # ">>State Logic  >>"
        # ">>> Time cluster >>>"
        # ">>> Yaw >>>"
        # ">>> Stepper position >>>"
        # ">>> Encoders >>>"
        # ">>> Object detection >>>"
        # ">>> Ultrasonic Sensors Detect >>>"
        n159 = call "Webcam AE.vi"("Camera states"=Webcam_AE."Dispose Camera Image Buffer") -> ()  [unwired: 2 in, 3 out]
      }
      frame "DISPOSE PROC BUFFERS" {
        # ">>> Line Sensor Cluster>>>"
        # ">>State Logic  >>"
        # ">>> IR Sensors >>>"
        # ">>> Time cluster >>>"
        # ">>> Object detection >>>"
        # ">>> Yaw >>>"
        # ">>> Ultrasonic Sensors Detect >>>"
        # ">>> Encoders >>>"
        # ">>> Stepper position >>>"
        n160 = call "IMAQ Reference AE.vi"("IMAQ AE States"=IMAQ_Reference_AE."Dispose Processing Buffer") -> ()  [unwired: 1 in, 2 out]
      }
      frame "-----ARM ACTIONS-----" {
      }
      frame "CLOSE CLAW" {
        n161 = call "Arduino Interfacing VI.vi"("Data to Write"=I2C_MASTER_WRITE_NEW_Type_Def."Close Claw", "AE Mode"=Arduino_Interfacing."Write to Arduino") -> ()  [unwired: 2 in, 2 out]
      }
      frame "OPEN CLAW" {
        n162 = call "Arduino Interfacing VI.vi"("Data to Write"=I2C_MASTER_WRITE_NEW_Type_Def."Open Claw", "AE Mode"=Arduino_Interfacing."Write to Arduino") -> ()  [unwired: 2 in, 2 out]
      }
      frame "Z STEPPER CAM HEIGHT" {
        n163 = call "Arduino Interfacing VI.vi"("Data to Write"=I2C_MASTER_WRITE_NEW_Type_Def."zStepper 6k", "AE Mode"=Arduino_Interfacing."Write to Arduino") -> ()  [unwired: 2 in, 2 out]
      }
      frame "Z STEPPER GRAB HEIGHT" {
        # ">>State Logic  >>"
        # ">>> Time cluster >>>"
        # ">>> Yaw >>>"
        # ">>> Stepper position >>>"
        # ">>> Encoders >>>"
        # ">>> Object detection >>>"
        # ">>> Ultrasonic Sensors Detect >>>"
        n164 = call "Arduino Interfacing VI.vi"("Data to Write"=I2C_MASTER_WRITE_NEW_Type_Def."zStepper 100", "AE Mode"=Arduino_Interfacing."Write to Arduino") -> ()  [unwired: 2 in, 2 out]
      }
      frame "Z STEPPER BOX HEIGHT" {
        # ">>> IR Sensors >>>"
        # ">>> Time cluster >>>"
        # ">>> Yaw >>>"
        # ">>> Stepper position >>>"
        # ">>> Encoders >>>"
        # ">>> Object detection >>>"
        # ">>> Ultrasonic Sensors Detect >>>"
        n165 = call "Arduino Interfacing VI.vi"("Data to Write"=I2C_MASTER_WRITE_NEW_Type_Def."zStepper 4k", "AE Mode"=Arduino_Interfacing."Write to Arduino") -> ()  [unwired: 2 in, 2 out]
      }
      frame "Y STEPPER CONTROL" {
        # ">>State Logic  >>"
        # ">>> yStepper command>>>"
        # ">>> Time cluster >>>"
        # ">>> Yaw >>>"
        # ">>> Stepper position >>>"
        # ">>> Encoders >>>"
        # ">>> Object detection >>>"
        # ">>> Ultrasonic Sensors Detect >>>"
        n166 = Unbundle By Name(w3356) -> ("yStepper desired"=w3355:u8)
        n167 = call "Arduino Interfacing VI.vi"("y Stepper value"=w3355, "Data to Write"=I2C_MASTER_WRITE_NEW_Type_Def."yStepper control", "AE Mode"=Arduino_Interfacing."Write to Arduino") -> ()  [unwired: 1 in, 2 out]
      }
      frame "READ STEPPER VALUES" {
        # ">>State Logic  >>"
        # ">>> Time cluster >>>"
        # ">>> Yaw >>>"
        # ">>> Stepper position >>>"
        # ">>> Encoders >>>"
        # ">>> Object detection >>>"
        # ">>> Ultrasonic Sensors Detect >>>"
        n168 = call "Arduino Interfacing VI.vi"("AE Mode"=Arduino_Interfacing."Read From Arduino") -> ("Arduino Data"=w3373:T15)  [unwired: 3 in, 1 out]
        n169 = Unbundle By Name(w3373) -> ("y Stepper Position"=w3372:u8, "z Stepper Position"=w3371:u8)
        n170 = Bundle By Name(cluster=w3376, "y Stepper Position"=w3372, "z Stepper Position"=w3371) -> (w3375:T5)
      }
      frame " -----TIMING-----" {
        # ">>State Logic  >>"
        # ">>> Time cluster >>>"
        # ">>> Yaw >>>"
        # ">>> Stepper position >>>"
        # ">>> Encoders >>>"
        # ">>> Object detection >>>"
        # ">>> Ultrasonic Sensors Detect >>>"
      }
      frame "SET TIMER 1" {
        # ">>State Logic  >>"
        # ">>> Time cluster >>>"
        # ">>> Yaw >>>"
        # ">>> Stepper position >>>"
        # ">>> Encoders >>>"
        # ">>> Object detection >>>"
        # ">>> Ultrasonic Sensors Detect >>>"
        n171 = call "Elasped Timer.vi"("Time Setting"=1.0, "Action"=Elapsed_timer_control."Initialize") -> ()  [unwired: 6 in, 4 out]
        n172 = Bundle By Name(cluster=w3398, "Time up flag"=FALSE) -> (w3396:T3)
      }
      frame "SET TIMER 2" {
        # ">>State Logic  >>"
        # ">>> Time cluster >>>"
        # ">>> Yaw >>>"
        # ">>> Stepper position >>>"
        # ">>> Encoders >>>"
        # ">>> Object detection >>>"
        # ">>> Ultrasonic Sensors Detect >>>"
        n173 = call "Elasped Timer.vi"("Time Setting"=2.0, "Action"=Elapsed_timer_control."Initialize") -> ()  [unwired: 6 in, 4 out]
        n174 = Bundle By Name(cluster=w3412, "Time up flag"=FALSE) -> (w3410:T3)
      }
      frame "SET TIMER 3" {
        # ">>State Logic  >>"
        # ">>> Time cluster >>>"
        # ">>> Yaw >>>"
        # ">>> Stepper position >>>"
        # ">>> Encoders >>>"
        # ">>> Object detection >>>"
        # ">>> Ultrasonic Sensors Detect >>>"
        n175 = call "Elasped Timer.vi"("Time Setting"=3.0, "Action"=Elapsed_timer_control."Initialize") -> ()  [unwired: 6 in, 4 out]
        n176 = Bundle By Name(cluster=w3426, "Time up flag"=FALSE) -> (w3424:T3)
      }
      frame "SET TIMER 4" {
        # ">>State Logic  >>"
        # ">>> Time cluster >>>"
        # ">>> Yaw >>>"
        # ">>> Stepper position >>>"
        # ">>> Encoders >>>"
        # ">>> Object detection >>>"
        # ">>> Ultrasonic Sensors Detect >>>"
        n177 = call "Elasped Timer.vi"("Time Setting"=4.0, "Action"=Elapsed_timer_control."Initialize") -> ()  [unwired: 6 in, 4 out]
        n178 = Bundle By Name(cluster=w3440, "Time up flag"=FALSE) -> (w3438:T3)
      }
      frame "SET TIMER 5" {
        # ">>State Logic  >>"
        # ">>> Time cluster >>>"
        # ">>> Yaw >>>"
        # ">>> Stepper position >>>"
        # ">>> Encoders >>>"
        # ">>> Object detection >>>"
        # ">>> Ultrasonic Sensors Detect >>>"
        n179 = call "Elasped Timer.vi"("Time Setting"=5.0, "Action"=Elapsed_timer_control."Initialize") -> ()  [unwired: 6 in, 4 out]
        n180 = Bundle By Name(cluster=w3454, "Time up flag"=FALSE) -> (w3452:T3)
      }
      frame "START TIMER" {
        # ">>State Logic  >>"
        # ">>> Time cluster >>>"
        # ">>> Yaw >>>"
        # ">>> Stepper position >>>"
        # ">>> Encoders >>>"
        # ">>> Object detection >>>"
        # ">>> Ultrasonic Sensors Detect >>>"
        n181 = call "Elasped Timer.vi"("Action"=Elapsed_timer_control."Start") -> ("Time Out?!"=w3464:bool)  [unwired: 7 in, 3 out]
        n182 = Bundle By Name(cluster=w3467, "Time up flag"=w3464) -> (w3466:T3)
      }
    }
    "State Logic" <- w246
    "Image Processing Error" <- w213
    n183 = local read "TASK ENABLE"() -> (w240:bool)
    n184 = Not(x=w240) -> (.not. x?=w239:bool)
    n185 = case shown="True" w247 {
      tunnel: w251 -> [w278 w318]
      tunnel: w255 -> [w274 w320]
      tunnel: [w278 w318] -> w260
      tunnel: [w274 w321] -> w259
      tunnel: w256 -> [_ w316]
      tunnel: w258 -> [_ w317]
      tunnel: w253 -> [w277 w323]
      tunnel: [w277 w323] -> w252
      tunnel: "STOP TASK" -> [_ w306]
      tunnel: w246 -> [w276 w322]
      tunnel: [w276 w319] -> w245
      tunnel: w242 -> [w275 w312]
      tunnel: [w275 w312] -> w241
      tunnel: w239 -> [_ w307]
      tunnel: [w273 w304] -> w238
      tunnel: w237 -> [w273 w303]
      tunnel: w235 -> [w272 w300]
      tunnel: [w272 w300] -> w234
      tunnel: w232 -> [w271 w296]
      tunnel: [w271 w296] -> w231
      tunnel: w229 -> [w270 w294]
      tunnel: [w270 w294] -> w228
      tunnel: w226 -> [w269 w292]
      tunnel: [w269 w292] -> w225
      tunnel: w224 -> [w268 w291]
      tunnel: [w268 w290] -> w223
      tunnel: [_ w288] -> w222
      tunnel: w220 -> [w267 w286]
      tunnel: [w267 w286] -> w219
      tunnel: w218 -> [w266 w285]
      tunnel: [w266 w284] -> w217
      tunnel: w215 -> [w265 w281]
      tunnel: [w265 w281] -> w214
      tunnel: [w264 w280] -> w212
      tunnel: w210 -> [w264 w279]
      frame False {
        # ">> Item Selection Bias >>"
        # ">>State Logic Queue Reference >>"
        # ">>Action states Queue Reference >>"
        # ">>True Stop Next State >>"
        # ">>State Logic  >>"
        # ">>> IR Sensors >>>"
        # ">>> Line Sensor Cluster>>>"
        # ">>> Line Sensor Cluster>>>"
        # ">>> Motor control cluster >>>"
        # ">>> yStepper command>>>"
        # ">>> Motor control cluster >>>"
        # ">>> yStepper command>>>"
        # ">>> Motor control cluster >>>"
        # ">>> IR Sensors >>>"
        # ">>> IR Sensors >>>"
        # ">>> yStepper command>>>"
        # ">>> Time cluster >>>"
        # ">>> Yaw >>>"
        # ">>> Stepper position >>>"
        # ">>> Encoders >>>"
        # ">>> Object detection >>>"
        # ">>> Ultrasonic Sensors Detect >>>"
        # ">>> Time cluster >>>"
        # ">>> Yaw >>>"
        # ">>> Stepper position >>>"
        # ">>> Encoders >>>"
        # ">>> Object detection >>>"
        # ">>> Ultrasonic Sensors Detect >>>"
      }
      frame True {
        # ">> Item Selection Bias >>"
        # ">>> IR Sensors >>>"
        # ">>> Line Sensor Cluster>>>"
        # ">>> Line Sensor Cluster>>>"
        # ">>> Motor control cluster >>>"
        # ">>> yStepper command>>>"
        # ">>> IR Sensors >>>"
        # ">>> Motor control cluster >>>"
        # ">>State Logic Queue Reference >>"
        # ">>Timeout>>"
        # ">>> yStepper command>>>"
        # ">>> Time cluster >>>"
        # ">>> Object detection >>>"
        # ">>> Yaw >>>"
        # ">>> Ultrasonic Sensors Detect >>>"
        # ">>> Encoders >>>"
        # ">>> Stepper position >>>"
        # ">>State Logic  >>"
        # ">>True Stop Next State >>"
        # ">>Action Queue>>"
        # ">> Manual override >>"
        # ">>> Time cluster >>>"
        # ">>> Yaw >>>"
        # ">>> Stepper position >>>"
        # ">>> Encoders >>>"
        # ">>> Object detection >>>"
        # ">>> Ultrasonic Sensors Detect >>>"
        # ">>Action Queue>>"
        # ">>State Logic Queue Reference >>"
        n186 = Or(x=w306, y=w307) -> (x .or. y?=w305:bool)
        n187 = Unbundle By Name(w281) -> ("Line Detected?"=w282:bool)
        n188 = Unbundle By Name(w286) -> ("Left IR Sensor"=w287:dbl, "Arm IR Sensor"=w283:dbl)
        n189 = Unbundle By Name(w292) -> ("Time up flag"=w293:bool)
        n190 = Unbundle By Name(w294) -> ("Yaw"=w295:dbl, "Compass"=w289:dbl)
        n191 = Unbundle By Name(w296) -> ("y Stepper Position"=w298:u8, "z Stepper Position"=w297:u8)
        n192 = Unbundle By Name(w312) -> ("xDistance"=w309:dbl, "yDistance"=w310:dbl, "wDistance"=w311:dbl)
        n193 = Unbundle By Name(w300) -> ("Recognized Object"=w299:bool, "Object X coordinate"=w302:dbl, "Object Y coordinate"=w301:dbl)
        n194 = Unbundle By Name(w323) -> ("PING_A"=w315:u8, "PING_B"=w314:u8, "PING_C"=w313:u8, "PING_D"=w308:u8)
        n195 = case shown="13" w322 {
          tunnel: [w328 w340 w354 w365 w483 w498 w535 w589 w632 w680 w724 w779 w827 w868 w929 w975 w1016 w1065 w1108 w1161 w1199 w1251 w1295 w1339 w1369 w1387 w1433 w1474 w1523 w1576 w1615 w1664 w1707 w1760 w1798 w1850 w1886 w1935 w1978 w2031 w2075 w2120 w2172 w2213 w2261 w2300 w2342 w2397 w2451 w2489 w2535 w2584 w2625 w2669] -> w321
          tunnel: w320 -> [w328 w343 w355 w368 w485 w499 w544 w587 w636 w681 w730 w772 w830 w875 w919 w978 w1022 w1064 w1111 w1151 w1205 w1241 w1290 w1330 w1369 w1377 w1436 w1480 w1522 w1575 w1621 w1663 w1710 w1750 w1804 w1840 w1890 w1942 w1983 w2036 w2080 w2124 w2170 w2214 w2262 w2302 w2352 w2407 w2450 w2493 w2541 w2583 w2629 w2673]
          tunnel: [State_Type_Definitions."Idle" ("Enum") State_Type_Definitions."Idle" ("Enum") w350 w367 State_Type_Definitions."Shutdown" ("Enum") w500 w542 w590 w633 w679 w725 w778 w828 w870 w928 w976 w1023 w1066 w1110 w1160 w1206 w1250 w1296 w1331 State_Type_Definitions."Idle" ("Enum") w1386 w1434 w1481 w1524 w1577 w1622 w1665 w1709 w1759 w1805 w1849 w1887 w1936 w1979 w2032 w2076 w2121 w2173 w2212 w2260 w2301 w2347 w2408 w2452 w2490 w2536 w2585 w2626 w2670] -> w319
          tunnel: w318 -> [_ _ w353 w371 _ w505 w538 w586 w637 w688 w729 w776 w831 w874 w926 w973 w1021 w1062 w1112 w1158 w1204 w1248 w1293 w1338 _ w1384 w1431 w1479 w1520 w1573 w1620 w1661 w1711 w1757 w1803 w1847 w1894 w1941 w1986 w2039 w2083 w2127 w2169 w2215 w2255 w2303 w2351 w2406 w2449 w2497 w2540 w2582 w2633 w2674]
          tunnel: w317 -> [_ _ _ w370 _ w504 w537 w585 w638 w687 w728 w775 w824 w873 w925 w972 w1020 w1061 w1113 w1157 w1203 w1247 w1292 w1336 _ w1383 w1430 w1478 w1519 w1572 w1619 w1660 w1712 w1756 w1802 w1846 w1889 w1940 w1985 w2038 w2082 w2123 w2168 w2216 w2256 w2304 w2350 w2405 w2448 w2496 w2539 w2581 w2632 w2675]
          tunnel: w316 -> [_ _ w352 w366 _ w503 w536 w584 w639 w686 w727 w774 w823 w872 w927 w974 w1019 w1060 w1114 w1159 w1202 w1249 w1291 w1337 _ w1385 w1432 w1477 w1518 w1571 w1618 w1659 w1713 w1758 w1801 w1848 w1893 w1939 w1984 w2037 w2081 w2126 w2167 w2217 w2257 w2305 w2349 w2404 w2447 w2495 w2538 w2580 w2631 w2676]
          tunnel: w305 -> [_ _ _ _ _ w497 w543 w583 w640 w683 w723 w777 w829 w876 w920 w979 w1017 w1063 w1115 w1152 w1200 w1242 w1294 w1334 _ w1378 w1437 w1475 w1521 w1574 w1616 w1662 w1714 w1751 w1799 w1841 w1892 w1934 w1982 w2035 w2079 w2125 w2166 w2218 w2258 w2306 w2348 w2403 w2446 w2494 w2537 w2579 w2630 w2677]
          tunnel: w315 -> [_ _ _ _ _ _ _ _ _ _ _ _ _ _ _ _ _ _ _ _ _ _ _ _ _ _ _ _ _ _ _ _ _ _ _ _ _ _ _ _ _ _ _ _ _ _ _ _ _ _ _ _ _ _]
          tunnel: w314 -> [_ _ _ _ _ _ _ w582 _ _ _ w768 w812 w866 _ w965 _ _ _ _ _ _ _ _ _ _ w1423 _ _ _ _ _ _ _ _ _ _ _ _ w2026 _ _ _ _ _ _ _ w2401 _ _ _ _ _ _]
          tunnel: w313 -> [_ _ _ _ _ _ _ w581 _ _ _ w769 w813 w867 _ w966 _ _ _ _ _ _ _ _ _ _ w1424 _ _ _ _ _ _ _ _ _ _ _ _ w2025 _ _ _ _ _ _ _ w2402 _ _ _ _ _ _]
          tunnel: w311 -> [_ _ _ _ _ _ _ _ _ w685 _ _ _ _ _ _ _ _ _ _ _ _ _ _ _ _ _ _ _ _ _ _ _ _ _ _ _ _ _ _ _ _ _ _ _ _ w2345 _ _ _ _ _ _ _]
          tunnel: w310 -> [_ _ _ _ _ w496 _ _ w631 _ _ _ _ w871 _ _ _ _ _ _ _ _ _ _ _ _ _ _ _ _ _ _ _ _ _ _ _ _ _ _ _ _ _ _ _ _ _ w2393 _ _ _ _ _ _]
          tunnel: w309 -> [_ _ _ _ _ _ _ _ _ _ _ _ w818 _ _ _ _ _ _ _ _ _ _ _ _ _ _ _ _ w1562 _ _ _ _ _ _ _ _ _ _ _ _ _ w2207 _ _ _ _ _ _ _ w2578 _ _]
          tunnel: w308 -> [_ _ _ _ _ _ _ _ _ _ _ _ _ _ _ _ _ _ _ _ _ _ _ _ _ _ _ _ _ _ _ _ _ _ _ _ _ _ _ _ _ _ _ _ _ _ _ _ _ _ _ _ _ _]
          tunnel: [State_Type_Definitions."Idle" ("Enum") State_Type_Definitions."Idle" ("Enum") State_Type_Definitions."Idle" ("Enum") State_Type_Definitions."Idle" ("Enum") State_Type_Definitions."Shutdown" ("Enum") w493 w541 w588 w634 w676 w722 w771 w826 w869 w930 w977 w1015 w1067 w1109 w1162 w1198 w1252 w1297 w1332 w1371 w1388 w1435 w1473 w1525 w1578 w1614 w1666 w1708 w1761 w1797 w1851 w1888 w1937 w1981 w2034 w2078 w2122 w2171 w2211 w2259 w2299 w2346 w2409 w2453 w2491 w2534 w2586 w2627 w2671] -> w304
          tunnel: w303 -> [_ _ w350 _ _ _ _ _ _ _ _ _ _ _ _ _ _ _ _ _ _ _ _ _ w1371 _ _ _ _ _ _ _ _ _ _ _ _ _ _ _ _ _ _ _ _ _ _ _ _ _ _ _ _ _]
          tunnel: w299 -> [_ _ _ _ _ _ _ _ _ _ _ _ _ _ _ _ _ _ _ _ _ _ _ w1333 _ _ _ _ _ _ _ _ _ _ _ _ _ _ _ _ _ _ _ _ _ _ _ _ _ _ _ _ _ _]
          tunnel: w302 -> [_ _ _ _ _ _ _ _ _ _ _ _ _ _ _ _ _ _ _ _ _ _ _ _ _ _ _ _ _ w1568 _ _ _ _ _ _ _ _ _ _ _ _ _ _ _ _ _ _ _ _ _ _ _ _]
          tunnel: w301 -> [_ _ _ _ _ _ _ _ _ _ _ _ _ _ _ _ _ _ w1104 _ _ _ _ _ _ _ _ _ _ _ _ _ w1703 _ _ _ _ _ _ _ _ _ _ _ _ _ _ _ _ _ _ _ _ _]
          tunnel: w298 -> [_ _ _ _ _ _ _ _ _ _ _ _ _ _ _ _ _ _ w1103 _ _ _ _ _ _ _ _ _ _ _ _ _ w1702 _ _ _ _ _ _ _ _ _ _ _ _ _ _ _ _ _ _ _ _ _]
          tunnel: w297 -> [_ _ _ _ _ _ w540 _ _ _ w720 _ _ _ w923 _ _ _ _ w1155 _ w1245 w1289 _ _ w1381 _ _ _ _ _ _ _ w1754 _ w1844 w1891 _ _ _ _ _ _ _ _ _ _ _ _ _ _ _ _ _]
          tunnel: w295 -> [_ _ _ _ _ _ _ _ _ _ _ _ _ _ _ _ _ _ _ _ _ _ _ _ _ _ _ _ _ _ _ _ _ _ _ _ _ _ _ _ _ _ _ _ _ _ _ _ _ _ _ _ _ _]
          tunnel: w293 -> [_ _ _ _ _ _ _ _ _ _ _ _ _ _ _ _ w1013 w1057 _ _ w1196 _ _ _ _ _ _ w1471 w1515 _ w1612 w1656 _ _ w1795 _ _ _ _ _ _ w2116 _ _ w2254 w2298 _ _ _ w2492 w2533 _ w2628 w2672]
          tunnel: w291 -> [w326 w338 w349 w363 w481 w492 w539 w580 w635 w675 w721 w770 w822 w865 w918 w970 w1014 w1058 w1106 w1150 w1197 w1240 w1286 w1329 w1372 w1376 w1428 w1472 w1516 w1569 w1613 w1657 w1705 w1749 w1796 w1839 w1885 w1938 w1980 w2033 w2077 w2119 w2165 w2220 w2264 w2308 w2354 w2411 w2455 w2499 w2543 w2591 w2635 w2679]
          tunnel: [w326 w337 w349 w363 w481 w492 w539 w580 w635 w675 w721 w770 w822 w865 w918 w970 w1014 w1058 w1105 w1150 w1197 w1240 w1286 w1329 w1372 w1376 w1428 w1472 w1516 w1569 w1613 w1657 w1704 w1749 w1796 w1839 w1885 w1938 w1980 w2033 w2077 w2119 w2165 w2220 w2264 w2308 w2354 w2411 w2455 w2499 w2543 w2591 w2635 w2679] -> w290
          tunnel: w289 -> [_ _ _ _ _ _ _ _ _ _ _ _ _ _ _ _ _ _ _ _ _ _ _ _ _ _ _ _ _ _ _ _ _ _ _ _ _ w1933 _ _ _ _ _ _ _ _ _ _ _ _ _ _ _ _]
          tunnel: [_ _ _ TRUE _ _ _ _ _ _ _ _ _ _ _ _ _ _ _ _ _ _ _ _ _ _ _ _ _ _ _ _ _ _ _ _ _ _ _ _ _ _ _ _ _ _ _ _ _ _ _ _ _ _] -> w288
          tunnel: w287 -> [_ _ _ _ _ _ _ _ _ _ _ _ _ _ _ _ _ _ _ _ _ _ _ _ _ _ _ _ _ _ _ _ _ _ _ _ _ _ _ _ _ _ _ _ _ _ _ _ _ _ _ _ _ _]
          tunnel: w285 -> [w325 w335 w348 w361 w480 w491 w534 w579 w628 w674 w717 w763 w811 w864 w917 w963 w1012 w1056 w1100 w1149 w1195 w1239 w1285 w1328 w1373 w1375 w1421 w1470 w1514 w1565 w1611 w1655 w1699 w1748 w1794 w1838 w1884 w1929 w1977 w2030 w2074 w2118 w2164 w2222 w2266 w2310 w2356 w2413 w2457 w2501 w2545 w2593 w2637 w2681]
          tunnel: [w325 w334 w348 w361 w480 w491 w534 w579 w628 w674 w717 w763 w811 w864 w917 w963 w1012 w1056 w1100 w1149 w1195 w1239 w1285 w1328 w1373 w1375 w1421 w1470 w1514 w1564 w1611 w1655 w1699 w1748 w1794 w1838 w1884 w1929 w1977 w2030 w2074 w2118 w2164 w2222 w2266 w2310 w2356 w2413 w2457 w2501 w2545 w2593 w2637 w2681] -> w284
          tunnel: w283 -> [_ _ _ _ _ _ _ _ _ _ _ _ _ _ _ _ _ _ _ _ _ _ _ _ _ _ _ _ _ _ _ _ _ _ _ _ _ _ _ w2028 _ _ w2163 _ _ _ _ w2399 _ _ _ _ _ _]
          tunnel: w282 -> [_ _ _ _ _ _ _ _ _ _ _ _ _ _ _ _ _ _ _ _ _ _ _ _ _ _ _ _ _ _ _ _ _ _ _ _ _ _ w1976 _ w2072 _ _ w2209 _ _ _ _ w2445 _ _ w2577 _ _]
          tunnel: [w324 w330 w347 w360 w479 w490 w533 w578 w627 w673 w716 w762 w810 w863 w916 w962 w1011 w1055 w1099 w1148 w1194 w1238 w1284 w1327 w1368 w1374 w1420 w1469 w1513 w1557 w1610 w1654 w1698 w1747 w1793 w1837 w1883 w1928 w1975 w2027 w2073 w2117 w2160 w2221 w2265 w2309 w2355 w2412 w2456 w2500 w2544 w2592 w2636 w2680] -> w280
          tunnel: w279 -> [w324 w330 w347 _ w479 w490 w533 w578 w627 w673 w716 w762 w810 w863 w916 w962 w1011 w1055 w1099 w1148 w1194 w1238 w1284 w1327 w1368 w1374 w1420 w1469 w1513 w1557 w1610 w1654 w1698 w1747 w1793 w1837 w1883 w1928 w1975 w2027 w2073 w2117 w2160 w2221 w2265 w2309 w2355 w2412 w2456 w2500 w2544 w2592 w2636 w2680]
          frame 0 {
            # ">>> yStepper command>>>"
          }
          frame 1 {
            # ">>> yStepper command>>>"
            n196 = for {
              shift-right: [w346] -> w340
              shift-left: w343 -> [w345]
              tunnel: string[] ["INIT", "RESET ARM", "RESET FLAGS", "RESET YAW", "NAVX CALIBRATE"] -> [w344] mode=indexing
              n197 = Enqueue Element(queue=w345, element=w344) -> (queue out=w346:refnum<queue>)  [unwired: 2 in, 2 out]
            }
            n198 = Bundle By Name(cluster=w338, "yStepper desired"=u8 0) -> (w337:T18)
            n199 = Bundle By Name(cluster=w335, "ySpeed"=0.0, "xSpeed"=0.0, "wSpeed"=0.0) -> (w334:T17)
          }
          frame 3 {
            # ">>Action Queue>>"
            # ">>> Motor control cluster >>>"
            # ">>> yStepper command>>>"
            n200 = Flush Queue(queue=w353, error in (no error)=w352) -> ()  [unwired: 3 out]
            n201 = for {
              shift-right: [w359] -> w354
              shift-left: w355 -> [w358]
              tunnel: string[] ["STOP", "RESET ENCODERS", "RESET YAW", "RESET ARM", "RESET FLAGS", "DISPOSE CAM BUFFERS", "DISPOSE PROC BUFFERS", "CAM CLOSE", ""] -> [w357] mode=indexing
              n202 = Enqueue Element(queue=w358, element=w357) -> (queue out=w359:refnum<queue>)  [unwired: 2 in, 2 out]
            }
          }
          frame 4, Default {
            # ">>> Motor control cluster >>>"
            # ">>> yStepper command>>>"
            n203 = Dequeue Element(queue=w371, timeout in ms (-1)=w370, error in (no error)=w366) -> (element=w369:T8)  [unwired: 3 out]
            n204 = case shown="\"Start Task 2\"" w369 {
              tunnel: [w374 w382 w390 w398 w406 w414 w422 w430 w438 w445 w455 w463 w470 w473] -> w365
              tunnel: w368 -> [w375 w383 w391 w399 w407 w415 w423 w431 w439 w446 w454 w462 w470 w474]
              tunnel: [State_Type_Definitions."Task 1" ("Enum") State_Type_Definitions."Task 2:Raise Arm" ("Enum") State_Type_Definitions."Task 3" ("Enum") State_Type_Definitions."Task 4_A" ("Enum") State_Type_Definitions."Task 5A: ARM CAM HEIGHT" ("Enum") State_Type_Definitions."Task 6_A" ("Enum") State_Type_Definitions."Task 8A: RAISE ARM" ("Enum") State_Type_Definitions."Task 8A: RAISE ARM" ("Enum") State_Type_Definitions."Task 8A: RAISE ARM" ("Enum") State_Type_Definitions."Task 8A: RAISE ARM" ("Enum") State_Type_Definitions."Task 9A: Raise Arm" ("Enum") State_Type_Definitions."Task 9F: SCAN IMAGE" ("Enum") State_Type_Definitions."Idle" ("Enum") State_Type_Definitions."Shutdown" ("Enum")] -> w367
              tunnel: [enum16{"Ball", "Soap", "Gel", "Pipe", "None"}."None" ("Object recognition mode") enum16{"Ball", "Soap", "Gel", "Pipe", "None"}."None" ("Object recognition mode") enum16{"Ball", "Soap", "Gel", "Pipe", "None"}."None" ("Object recognition mode") enum16{"Ball", "Soap", "Gel", "Pipe", "None"}."None" ("Object recognition mode") enum16{"Ball", "Soap", "Gel", "Pipe", "None"}."None" ("Object recognition mode") enum16{"Ball", "Soap", "Gel", "Pipe", "None"}."None" ("Object recognition mode") enum16{"Ball", "Soap", "Gel", "Pipe", "None"}."Ball" ("Object recognition mode") enum16{"Ball", "Soap", "Gel", "Pipe", "None"}."Gel" ("Object recognition mode") enum16{"Ball", "Soap", "Gel", "Pipe", "None"}."Pipe" ("Object recognition mode") enum16{"Ball", "Soap", "Gel", "Pipe", "None"}."Soap" ("Object recognition mode") enum16{"Ball", "Soap", "Gel", "Pipe", "None"}."None" ("Object recognition mode") enum16{"Ball", "Soap", "Gel", "Pipe", "None"}."None" ("Object recognition mode") enum16{"Ball", "Soap", "Gel", "Pipe", "None"}."None" ("Object recognition mode") enum16{"Ball", "Soap", "Gel", "Pipe", "None"}."None" ("Object recognition mode")] -> w360
              frame "Start Task 1" {
                n205 = for {
                  shift-right: [w379] -> w374
                  shift-left: w375 -> [w378]
                  tunnel: string[] ["RESET ENCODERS", "RESET YAW", "FORWARD", "READ ENCODERS"] -> [w377] mode=indexing
                  n206 = Enqueue Element(queue=w378, element=w377) -> (queue out=w379:refnum<queue>)  [unwired: 2 in, 2 out]
                }
              }
              frame "Start Task 2" {
                n207 = for {
                  shift-right: [w387] -> w382
                  shift-left: w383 -> [w386]
                  tunnel: string[] ["RESET ENCODERS", "RESET YAW", "READ ULTRASONIC", "ARDUINO - ULTRASONIC"] -> [w385] mode=indexing
                  n208 = Enqueue Element(queue=w386, element=w385) -> (queue out=w387:refnum<queue>)  [unwired: 2 in, 2 out]
                }
              }
              frame "Start Task 3" {
                n209 = for {
                  shift-right: [w395] -> w390
                  shift-left: w391 -> [w394]
                  tunnel: string[] ["RESET ENCODERS", "READ ENCODERS", "R-ACW"] -> [w393] mode=indexing
                  n210 = Enqueue Element(queue=w394, element=w393) -> (queue out=w395:refnum<queue>)  [unwired: 2 in, 2 out]
                }
              }
              frame "Start Task 4" {
                n211 = for {
                  shift-right: [w403] -> w398
                  shift-left: w399 -> [w402]
                  tunnel: string[] ["RESET YAW", "RESET ENCODERS", "RESET ARM", "RESET FLAGS", "", ""] -> [w401] mode=indexing
                  n212 = Enqueue Element(queue=w402, element=w401) -> (queue out=w403:refnum<queue>)  [unwired: 2 in, 2 out]
                }
              }
              frame "Start Task 5" {
                n213 = for {
                  shift-right: [w411] -> w406
                  shift-left: w407 -> [w410]
                  tunnel: string[] ["RESET YAW", "RESET ENCODERS", "READ STEPPER VALUES", "Z STEPPER CAM HEIGHT", "", ""] -> [w409] mode=indexing
                  n214 = Enqueue Element(queue=w410, element=w409) -> (queue out=w411:refnum<queue>)  [unwired: 2 in, 2 out]
                }
              }
              frame "Start Task 6" {
                n215 = for {
                  shift-right: [w419] -> w414
                  shift-left: w415 -> [w418]
                  tunnel: string[] ["OPEN LOG CAM ", "", "", "", "", ""] -> [w417] mode=indexing
                  n216 = Enqueue Element(queue=w418, element=w417) -> (queue out=w419:refnum<queue>)  [unwired: 2 in, 2 out]
                }
              }
              frame "Start Task 8 - BALL" {
                n217 = for {
                  shift-right: [w427] -> w422
                  shift-left: w423 -> [w426]
                  tunnel: string[] ["RESET YAW", "RESET ENCODERS", "RESET ARM", "RESET FLAGS"] -> [w425] mode=indexing
                  n218 = Enqueue Element(queue=w426, element=w425) -> (queue out=w427:refnum<queue>)  [unwired: 2 in, 2 out]
                }
              }
              frame "Start Task 8 - Gel" {
                n219 = for {
                  shift-right: [w435] -> w430
                  shift-left: w431 -> [w434]
                  tunnel: string[] ["RESET YAW", "RESET ENCODERS", "RESET ARM", "RESET FLAGS"] -> [w433] mode=indexing
                  n220 = Enqueue Element(queue=w434, element=w433) -> (queue out=w435:refnum<queue>)  [unwired: 2 in, 2 out]
                }
              }
              frame "Start Task 8 - Pipe" {
                n221 = for {
                  shift-right: [w443] -> w438
                  shift-left: w439 -> [w442]
                  tunnel: string[] ["RESET YAW", "RESET ENCODERS", "RESET ARM", "RESET FLAGS"] -> [w441] mode=indexing
                  n222 = Enqueue Element(queue=w442, element=w441) -> (queue out=w443:refnum<queue>)  [unwired: 2 in, 2 out]
                }
              }
              frame "Start Task 8 - Soap" {
                n223 = for {
                  shift-right: [w451] -> w445
                  shift-left: w446 -> [w450]
                  tunnel: string[] ["RESET YAW", "RESET ENCODERS", "RESET ARM", "RESET FLAGS"] -> [w449] mode=indexing
                  n224 = Enqueue Element(queue=w450, element=w449) -> (queue out=w451:refnum<queue>)  [unwired: 2 in, 2 out]
                }
              }
              frame "Start Task 9" {
                n225 = for {
                  shift-right: [w459] -> w455
                  shift-left: w454 -> [w458]
                  tunnel: string[] ["RESET ENCODERS", "READ ENCODERS", "Z STEPPER BOX HEIGHT"] -> [w457] mode=indexing
                  n226 = Enqueue Element(queue=w458, element=w457) -> (queue out=w459:refnum<queue>)  [unwired: 2 in, 2 out]
                }
              }
              frame "Start Task A" {
                n227 = for {
                  shift-right: [w467] -> w463
                  shift-left: w462 -> [w466]
                  tunnel: string[] ["RESET ENCODERS", "READ ENCODERS", "RESET YAW", "Z STEPPER BOX HEIGHT"] -> [w465] mode=indexing
                  n228 = Enqueue Element(queue=w466, element=w465) -> (queue out=w467:refnum<queue>)  [unwired: 2 in, 2 out]
                }
              }
              frame "None", Default {
              }
              frame "Exit" {
                n229 = for {
                  shift-right: [w478] -> w473
                  shift-left: w474 -> [w477]
                  tunnel: string[] ["STOP", "RESET ENCODERS", "RESET YAW", "EXIT"] -> [w476] mode=indexing
                  n230 = Enqueue Element(queue=w477, element=w476) -> (queue out=w478:refnum<queue>)  [unwired: 2 in, 2 out]
                }
              }
            }
          }
          frame 5 {
            # ">> Item Selection Bias >>"
            # ">>> yStepper command>>>"
            n231 = for {
              shift-right: [w489] -> w483
              shift-left: w485 -> [w488]
              tunnel: string[] ["INIT", "RESET ENCODERS", "RESET FLAGS", "CAM CLOSE", "DISPOSE BUFFERS", "EXIT", ""] -> [w487] mode=indexing
              n232 = Enqueue Element(queue=w488, element=w487) -> (queue out=w489:refnum<queue>)  [unwired: 2 in, 2 out]
            }
          }
          frame 6 {
            # ">>> yStepper command>>>"
            # "Use 250"
            n233 = Dequeue Element(queue=w505, timeout in ms (-1)=w504, error in (no error)=w503) -> (element=w502:T8)  [unwired: 3 out]
            n234 = Greater?(x=w496, y=265.0) -> (0:w494:bool)
            n235 = Or(x=w494, y=w497) -> (x .or. y?=w501:bool)
            n236 = case shown="\"Start Task 1\", Default" w502 {
              tunnel: w501 -> [w508 _]
              tunnel: [w512 State_Type_Definitions."True Stop" ("Enum")] -> w500
              tunnel: w499 -> [w509 w527]
              tunnel: [w507 w526] -> w498
              tunnel: [State_Type_Definitions."Idle" ("Enum") State_Type_Definitions."Shutdown" ("Enum")] -> w493
              frame "Start Task 1", Default {
                n237 = case shown="True" w508 {
                  tunnel: w509 -> [w515 w521]
                  tunnel: [w514 w519] -> w507
                  frame False {
                    n238 = for {
                      shift-right: [w517] -> w514
                      shift-left: w515 -> [w518]
                      tunnel: string[] ["READ ENCODERS", "READ NAVX", "FORWARD"] ("element") -> [w516] mode=indexing
                      n239 = Enqueue Element(queue=w518, element=w516) -> (queue out=w517:refnum<queue>)  [unwired: 2 in, 2 out]
                    }
                  }
                  frame True {
                    n240 = for {
                      shift-right: [w523] -> w519
                      shift-left: w521 -> [w524]
                      tunnel: string[] ["RESET YAW", "RESET ENCODERS", "STOP", ""] -> [w522] mode=indexing
                      n241 = Enqueue Element(queue=w524, element=w522) -> (queue out=w523:refnum<queue>)  [unwired: 2 in, 2 out]
                    }
                  }
                }
                n242 = Select(t=State_Type_Definitions."True Stop" ("Enum"), s=w508, f=State_Type_Definitions."Task 1" ("Enum")) -> (s? t:f=w512:u16)
              }
              frame "Exit" {
                n243 = for {
                  shift-right: [w531] -> w526
                  shift-left: w527 -> [w532]
                  tunnel: string[] ["STOP", "RESET ENCODERS", "RESET YAW", ""] -> [w530] mode=indexing
                  n244 = Enqueue Element(queue=w532, element=w530) -> (queue out=w531:refnum<queue>)  [unwired: 2 in, 2 out]
                }
              }
            }
          }
          frame 8 {
            # ">> Stepper height reeached >>"
            # ">>> yStepper command>>>"
            # ">> Manual override >>"
            n245 = Dequeue Element(queue=w538, timeout in ms (-1)=w537, error in (no error)=w536) -> (element=w547:T8)  [unwired: 3 out]
            n246 = Equal?(x=w540, y=u8 60) -> (x = y?=w545:bool)
            n247 = case shown="\"Start Task 1\", Default" w547 {
              tunnel: [w558 State_Type_Definitions."True Stop" ("Enum")] -> w542
              tunnel: [w556 w573] -> w535
              tunnel: w544 -> [w555 _]
              tunnel: w543 -> [w549 _]
              tunnel: [State_Type_Definitions."Idle" ("Enum") State_Type_Definitions."Shutdown" ("Enum")] -> w541
              tunnel: w545 -> [w548 _]
              frame "Start Task 1", Default {
                # ">> WIill proceed to part ii if not manual override >>"
                # ">>If ENABLE or Trigger is set to true>>"
                n248 = Or(x=w548, y=w549) -> (x .or. y?=w550:bool)
                n249 = case shown="True" w548 {
                  tunnel: [w561 w567] -> w556
                  tunnel: w555 -> [w560 w566]
                  frame False {
                    n250 = for {
                      shift-right: [w563] -> w561
                      shift-left: w560 -> [w564]
                      tunnel: string[] ["Z STEPPER CAM HEIGHT", "READ STEPPER VALUES"] ("element") -> [w562] mode=indexing
                      n251 = Enqueue Element(queue=w564, element=w562) -> (queue out=w563:refnum<queue>)  [unwired: 2 in, 2 out]
                    }
                  }
                  frame True {
                    n252 = for {
                      shift-right: [w569] -> w567
                      shift-left: w566 -> [w570]
                      tunnel: string[] ["ARDUINO - ULTRASONIC", "READ ULTRASONIC", "", "", "", ""] -> [w568] mode=indexing
                      n253 = Enqueue Element(queue=w570, element=w568) -> (queue out=w569:refnum<queue>)  [unwired: 2 in, 2 out]
                    }
                  }
                }
                n254 = Select(t=State_Type_Definitions."True Stop" ("Enum"), s=w549, f=State_Type_Definitions."Task 2:Sensor Mode" ("Enum")) -> (s? t:f=w552:T16)
                n255 = Select(t=w552, s=w550, f=State_Type_Definitions."Task 2:Raise Arm" ("Enum")) -> (s? t:f=w558:T16)
              }
              frame "Exit" {
                n256 = for {
                  shift-right: [w576] -> w573
                  shift-left: _ -> [w577]
                  tunnel: string[] ["STOP", "RESET ENCODERS", "RESET YAW", ""] -> [w575] mode=indexing
                  n257 = Enqueue Element(queue=w577, element=w575) -> (queue out=w576:refnum<queue>)  [unwired: 2 in, 2 out]
                }
              }
            }
          }
          frame 9 {
            w594 = u8 20 ("y")
            # ">>> yStepper command>>>"
            # ">>Object detected>>"
            n258 = Dequeue Element(queue=w586, timeout in ms (-1)=w585, error in (no error)=w584) -> (element=w595:T8)  [unwired: 3 out]
            n259 = Less?(x=w582, y=w594) -> (x < y?=w593:bool)
            n260 = Less?(x=w581, y=w594) -> (x < y?=w592:bool)
            n261 = Or(x=w593, y=w592) -> (x .or. y?=w591:bool)
            "Obstacle detected" <- w591
            n262 = case shown="\"Start Task 1\", Default" w595 {
              tunnel: w591 -> [w598 _]
              tunnel: [w605 State_Type_Definitions."True Stop" ("Enum")] -> w590
              tunnel: w583 -> [w597 _]
              tunnel: w587 -> [w604 w621]
              tunnel: [w603 w622] -> w589
              tunnel: [State_Type_Definitions."Idle" ("Enum") State_Type_Definitions."Shutdown" ("Enum")] -> w588
              frame "Start Task 1", Default {
                n263 = case shown="False" w598 {
                  tunnel: w604 -> [w608 w615]
                  tunnel: [w609 w614] -> w603
                  frame False {
                    n264 = for {
                      tunnel: string[] ["READ ULTRASONIC", "STOP"] ("element") -> [w610] mode=indexing
                      shift-right: [w612] -> w609
                      shift-left: w608 -> [w611]
                      n265 = Enqueue Element(queue=w611, element=w610) -> (queue out=w612:refnum<queue>)  [unwired: 2 in, 2 out]
                    }
                  }
                  frame True {
                    n266 = for {
                      shift-right: [w617] -> w614
                      shift-left: w615 -> [w618]
                      tunnel: string[] ["RESET ENCODERS", "READ NAVX", "READ ENCODERS"] -> [w616] mode=indexing
                      n267 = Enqueue Element(queue=w618, element=w616) -> (queue out=w617:refnum<queue>)  [unwired: 2 in, 2 out]
                    }
                  }
                }
                n268 = Or(x=w598, y=w597) -> (x .or. y?=w596:bool)
                n269 = Select(t=State_Type_Definitions."True Stop" ("Enum"), s=w597, f=State_Type_Definitions."Task 2:Reverse Mode" ("Enum")) -> (s? t:f=w599:T16)
                n270 = Select(t=w599, s=w596, f=State_Type_Definitions."Task 2:Sensor Mode" ("Enum")) -> (s? t:f=w605:T16)
              }
              frame "Exit" {
                n271 = for {
                  shift-right: [w625] -> w622
                  shift-left: w621 -> [w626]
                  tunnel: string[] ["STOP", "RESET ENCODERS", "RESET YAW", "ARDUINO MODE 0"] -> [w624] mode=indexing
                  n272 = Enqueue Element(queue=w626, element=w624) -> (queue out=w625:refnum<queue>)  [unwired: 2 in, 2 out]
                }
              }
            }
          }
          frame 10 {
            # ">>> yStepper command>>>"
            n273 = Dequeue Element(queue=w637, timeout in ms (-1)=w638, error in (no error)=w639) -> (element=w641:T8)  [unwired: 3 out]
            n274 = Less?(x=w631, y=-50.0) -> (x < y?=w629:bool)
            n275 = case shown="\"Start Task 1\", Default" w641 {
              tunnel: [w651 State_Type_Definitions."True Stop" ("Enum")] -> w633
              tunnel: w640 -> [w644 _]
              tunnel: w636 -> [w650 w667]
              tunnel: [w649 w668] -> w632
              tunnel: [State_Type_Definitions."Idle" ("Enum") State_Type_Definitions."Shutdown" ("Enum")] -> w634
              tunnel: w629 -> [w642 _]
              frame "Start Task 1", Default {
                n276 = case shown="True" w642 {
                  tunnel: w650 -> [w654 w661]
                  tunnel: [w655 w660] -> w649
                  frame False {
                    n277 = for {
                      tunnel: string[] ["READ ENCODERS", "REVERSE", "READ NAVX"] ("element") -> [w656] mode=indexing
                      shift-right: [w658] -> w655
                      shift-left: w654 -> [w657]
                      n278 = Enqueue Element(queue=w657, element=w656) -> (queue out=w658:refnum<queue>)  [unwired: 2 in, 2 out]
                    }
                  }
                  frame True {
                    n279 = for {
                      shift-right: [w663] -> w660
                      shift-left: w661 -> [w664]
                      tunnel: string[] ["STOP", "ARDUINO - ULTRASONIC", "READ ULTRASONIC", "RESET ENCODERS"] -> [w662] mode=indexing
                      n280 = Enqueue Element(queue=w664, element=w662) -> (queue out=w663:refnum<queue>)  [unwired: 2 in, 2 out]
                    }
                  }
                }
                n281 = Or(x=w642, y=w644) -> (x .or. y?=w643:bool)
                n282 = Select(t=State_Type_Definitions."True Stop" ("Enum"), s=w644, f=State_Type_Definitions."Task 2:Sensor Mode" ("Enum")) -> (s? t:f=w645:T16)
                n283 = Select(t=w645, s=w643, f=State_Type_Definitions."Task 2:Reverse Mode" ("Enum")) -> (s? t:f=w651:T16)
              }
              frame "Exit" {
                n284 = for {
                  shift-right: [w671] -> w668
                  shift-left: w667 -> [w672]
                  tunnel: string[] ["STOP", "RESET ENCODERS", "RESET YAW", "ARDUINO MODE 0"] -> [w670] mode=indexing
                  n285 = Enqueue Element(queue=w672, element=w670) -> (queue out=w671:refnum<queue>)  [unwired: 2 in, 2 out]
                }
              }
            }
          }
          frame 11 {
            # ">>> Motor control cluster >>>"
            # ">>> yStepper command>>>"
            n286 = Dequeue Element(queue=w688, timeout in ms (-1)=w687, error in (no error)=w686) -> (element=w677:T8)  [unwired: 3 out]
            n287 = Less?(x=w685, y=-160.0) -> (x < y?=w682:bool)
            n288 = Or(x=w682, y=w683) -> (x .or. y?=w678:bool)
            n289 = case shown="\"Start Task 1\", Default" w677 {
              tunnel: w678 -> [w691 _]
              tunnel: [w695 State_Type_Definitions."True Stop" ("Enum")] -> w679
              tunnel: w681 -> [w692 w711]
              tunnel: [w690 w710] -> w680
              tunnel: [State_Type_Definitions."Idle" ("Enum") State_Type_Definitions."Shutdown" ("Enum")] -> w676
              frame "Start Task 1", Default {
                n290 = case shown="False" w691 {
                  tunnel: w692 -> [w698 w704]
                  tunnel: [w697 w702] -> w690
                  frame False {
                    n291 = for {
                      shift-right: [w700] -> w697
                      shift-left: w698 -> [w701]
                      tunnel: string[] ["READ ENCODERS", "R-CW"] ("element") -> [w699] mode=indexing
                      n292 = Enqueue Element(queue=w701, element=w699) -> (queue out=w700:refnum<queue>)  [unwired: 2 in, 2 out]
                    }
                  }
                  frame True {
                    n293 = for {
                      shift-right: [w706] -> w702
                      shift-left: w704 -> [w707]
                      tunnel: string[] ["RESET YAW", "RESET ENCODERS", "STOP", "ARDUINO MODE 0"] -> [w705] mode=indexing
                      n294 = Enqueue Element(queue=w707, element=w705) -> (queue out=w706:refnum<queue>)  [unwired: 2 in, 2 out]
                    }
                  }
                }
                n295 = Select(t=State_Type_Definitions."True Stop" ("Enum"), s=w691, f=State_Type_Definitions."Task 3" ("Enum")) -> (s? t:f=w695:T16)
              }
              frame "Exit" {
                n296 = for {
                  shift-right: [w714] -> w710
                  shift-left: w711 -> [w715]
                  tunnel: string[] ["STOP", "RESET ENCODERS", "RESET YAW", ""] -> [w713] mode=indexing
                  n297 = Enqueue Element(queue=w715, element=w713) -> (queue out=w714:refnum<queue>)  [unwired: 2 in, 2 out]
                }
              }
            }
          }
          frame 12 {
            # ">> Stepper height reeached >>"
            # ">>> yStepper command>>>"
            # ">> Manual override >>"
            n298 = Dequeue Element(queue=w729, timeout in ms (-1)=w728, error in (no error)=w727) -> (element=w726:T8)  [unwired: 3 out]
            n299 = Equal?(x=w720, y=u8 60) -> (x = y?=w718:bool)
            n300 = case shown="\"Start Task 1\", Default" w726 {
              tunnel: [w741 State_Type_Definitions."True Stop" ("Enum")] -> w725
              tunnel: [w739 w757] -> w724
              tunnel: w730 -> [w738 w754]
              tunnel: w723 -> [w732 _]
              tunnel: [State_Type_Definitions."Idle" ("Enum") State_Type_Definitions."Shutdown" ("Enum")] -> w722
              tunnel: w718 -> [w731 _]
              frame "Start Task 1", Default {
                # ">> WIill proceed to part ii if not manual override >>"
                # ">>If ENABLE or Trigger is set to true>>"
                n301 = Or(x=w731, y=w732) -> (x .or. y?=w733:bool)
                n302 = case shown="False" w731 {
                  tunnel: [w744 w750] -> w739
                  tunnel: w738 -> [w743 w749]
                  frame False {
                    n303 = for {
                      shift-right: [w746] -> w744
                      shift-left: w743 -> [w747]
                      tunnel: string[] ["Z STEPPER CAM HEIGHT", "READ STEPPER VALUES"] ("element") -> [w745] mode=indexing
                      n304 = Enqueue Element(queue=w747, element=w745) -> (queue out=w746:refnum<queue>)  [unwired: 2 in, 2 out]
                    }
                  }
                  frame True {
                    n305 = for {
                      shift-right: [w752] -> w750
                      shift-left: w749 -> [w753]
                      tunnel: string[] ["ARDUINO - ULTRASONIC", "READ ULTRASONIC", "FORWARD", "", "", ""] -> [w751] mode=indexing
                      n306 = Enqueue Element(queue=w753, element=w751) -> (queue out=w752:refnum<queue>)  [unwired: 2 in, 2 out]
                    }
                  }
                }
                n307 = Select(t=State_Type_Definitions."True Stop" ("Enum"), s=w732, f=State_Type_Definitions."Task 4_B" ("Enum")) -> (s? t:f=w735:T16)
                n308 = Select(t=w735, s=w733, f=State_Type_Definitions."Task 4_A" ("Enum")) -> (s? t:f=w741:T16)
              }
              frame "Exit" {
                n309 = for {
                  shift-right: [w760] -> w757
                  shift-left: w754 -> [w761]
                  tunnel: string[] ["STOP", "RESET ENCODERS", "RESET YAW", ""] -> [w759] mode=indexing
                  n310 = Enqueue Element(queue=w761, element=w759) -> (queue out=w760:refnum<queue>)  [unwired: 2 in, 2 out]
                }
              }
            }
          }
          frame 13 {
            w767 = u8 20
            # ">> Path blocked >>"
            # ">>> yStepper command>>>"
            # ">> Manual override >>"
            n311 = Dequeue Element(queue=w776, timeout in ms (-1)=w775, error in (no error)=w774) -> (element=w773:T8)  [unwired: 3 out]
            n312 = Less?(x=w769, y=w767) -> (x < y?=w764:bool)
            n313 = Less?(x=w768, y=w767) -> (x < y?=w765:bool)
            n314 = And(x=w765, y=w764) -> (x .and. y?=w766:bool)
            n315 = case shown="\"Start Task 1\", Default" w773 {
              tunnel: [w790 State_Type_Definitions."True Stop" ("Enum")] -> w778
              tunnel: [w788 w805] -> w779
              tunnel: w772 -> [w787 _]
              tunnel: w777 -> [w781 _]
              tunnel: [State_Type_Definitions."Idle" ("Enum") State_Type_Definitions."Shutdown" ("Enum")] -> w771
              tunnel: w766 -> [w780 _]
              frame "Start Task 1", Default {
                # ">> Manual override forces program to true stop >>"
                # ">>If ENABLE or Trigger is set to true>>"
                n316 = Or(x=w780, y=w781) -> (x .or. y?=w786:bool)
                n317 = case shown="False" w780 {
                  tunnel: [w793 w798] -> w788
                  tunnel: w787 -> [w792 w797]
                  frame False {
                    n318 = for {
                      shift-right: [w795] -> w793
                      shift-left: w792 -> [w796]
                      tunnel: string[] ["FORWARD", "READ ULTRASONIC", "READ NAVX"] ("element") -> [w794] mode=indexing
                      n319 = Enqueue Element(queue=w796, element=w794) -> (queue out=w795:refnum<queue>)  [unwired: 2 in, 2 out]
                    }
                  }
                  frame True {
                    n320 = for {
                      shift-right: [w801] -> w798
                      shift-left: w797 -> [w802]
                      tunnel: string[] ["STOP", "RESET YAW", "RESET ENCODERS", "RESET FLAGS"] -> [w800] mode=indexing
                      n321 = Enqueue Element(queue=w802, element=w800) -> (queue out=w801:refnum<queue>)  [unwired: 2 in, 2 out]
                    }
                  }
                }
                n322 = Select(t=State_Type_Definitions."True Stop" ("Enum"), s=w781, f=State_Type_Definitions."Task 4_C" ("Enum")) -> (s? t:f=w783:T16)
                n323 = Select(t=w783, s=w786, f=State_Type_Definitions."Task 4_B" ("Enum")) -> (s? t:f=w790:T16)
              }
              frame "Exit" {
                n324 = for {
                  shift-right: [w808] -> w805
                  shift-left: _ -> [w809]
                  tunnel: string[] ["STOP", "RESET ENCODERS", "RESET YAW", ""] -> [w807] mode=indexing
                  n325 = Enqueue Element(queue=w809, element=w807) -> (queue out=w808:refnum<queue>)  [unwired: 2 in, 2 out]
                }
              }
            }
          }
          frame 14 {
            w821 = u8 20
            # ">> xDistance travelled>>"
            # ">> Path NOT blocked >>"
            # ">>> yStepper command>>>"
            # ">> Manual override >>"
            n326 = Dequeue Element(queue=w831, timeout in ms (-1)=w824, error in (no error)=w823) -> (element=w825:T8)  [unwired: 3 out]
            n327 = Greater?(x=w813, y=w821) -> (0:w819:bool)
            n328 = Greater?(x=w818, y=80.0) -> (0:w816:bool)
            n329 = Greater?(x=w812, y=w821) -> (0:w820:bool)
            n330 = And(x=w820, y=w819) -> (x .and. y?=w815:bool)
            n331 = And(x=w816, y=w815) -> (x .and. y?=w814:bool)
            n332 = case shown="\"Start Task 1\", Default" w825 {
              tunnel: [w842 State_Type_Definitions."True Stop" ("Enum")] -> w828
              tunnel: [w840 w858] -> w827
              tunnel: w830 -> [w839 w855]
              tunnel: w829 -> [w833 _]
              tunnel: [State_Type_Definitions."Idle" ("t") State_Type_Definitions."Shutdown" ("Enum")] -> w826
              tunnel: w814 -> [w832 _]
              frame "Start Task 1", Default {
                # ">> Manual override forces program to true stop >>"
                # ">>If ENABLE or Trigger is set to true>>"
                n333 = Or(x=w832, y=w833) -> (x .or. y?=w838:bool)
                n334 = case shown="False" w832 {
                  tunnel: [w845 w850] -> w840
                  tunnel: w839 -> [w843 w849]
                  frame False {
                    n335 = for {
                      shift-right: [w847] -> w845
                      shift-left: w843 -> [w848]
                      tunnel: string[] ["RIGHT", "READ NAVX", "READ ENCODERS", "READ ULTRASONIC"] ("element") -> [w846] mode=indexing
                      n336 = Enqueue Element(queue=w848, element=w846) -> (queue out=w847:refnum<queue>)  [unwired: 2 in, 2 out]
                    }
                  }
                  frame True {
                    n337 = for {
                      shift-right: [w853] -> w850
                      shift-left: w849 -> [w854]
                      tunnel: string[] ["STOP", "RESET YAW", "RESET ENCODERS", "ARDUINO - ULTRASONIC"] -> [w852] mode=indexing
                      n338 = Enqueue Element(queue=w854, element=w852) -> (queue out=w853:refnum<queue>)  [unwired: 2 in, 2 out]
                    }
                  }
                }
                n339 = Select(t=State_Type_Definitions."True Stop" ("Enum"), s=w833, f=State_Type_Definitions."Task 4_D" ("Enum")) -> (s? t:f=w834:T16)
                n340 = Select(t=w834, s=w838, f=State_Type_Definitions."Task 4_C" ("Enum")) -> (s? t:f=w842:T16)
              }
              frame "Exit" {
                n341 = for {
                  shift-right: [w861] -> w858
                  shift-left: w855 -> [w862]
                  tunnel: string[] ["STOP", "RESET ENCODERS", "RESET YAW", ""] -> [w860] mode=indexing
                  n342 = Enqueue Element(queue=w862, element=w860) -> (queue out=w861:refnum<queue>)  [unwired: 2 in, 2 out]
                }
              }
            }
          }
          frame 15 {
            w883 = u8 20
            # ">> yDistance travelled>>"
            # ">> Path blocked >>"
            # ">>> yStepper command>>>"
            # ">> Manual override >>"
            n343 = Dequeue Element(queue=w874, timeout in ms (-1)=w873, error in (no error)=w872) -> (element=w884:T8)  [unwired: 3 out]
            n344 = Less?(x=w867, y=w883) -> (x < y?=w881:bool)
            n345 = Greater?(x=w871, y=200.0) -> (0:w879:bool)
            n346 = Less?(x=w866, y=w883) -> (x < y?=w882:bool)
            n347 = And(x=w882, y=w881) -> (x .and. y?=w878:bool)
            n348 = Or(x=w879, y=w878) -> (x .or. y?=w877:bool)
            n349 = case shown="\"Start Task 1\", Default" w884 {
              tunnel: [w895 State_Type_Definitions."True Stop" ("Enum")] -> w870
              tunnel: [w893 w911] -> w868
              tunnel: w875 -> [w892 w908]
              tunnel: w876 -> [w886 _]
              tunnel: [State_Type_Definitions."Idle" ("t") State_Type_Definitions."Shutdown" ("Enum")] -> w869
              tunnel: w877 -> [w885 _]
              frame "Start Task 1", Default {
                # ">> Manual override forces program to true stop >>"
                # ">>If ENABLE or Trigger is set to true>>"
                n350 = Or(x=w885, y=w886) -> (x .or. y?=w891:bool)
                n351 = case shown="True" w885 {
                  tunnel: [w898 w903] -> w893
                  tunnel: w892 -> [w896 w902]
                  frame False {
                    n352 = for {
                      shift-right: [w900] -> w898
                      shift-left: w896 -> [w901]
                      tunnel: string[] ["FORWARD", "READ NAVX", "READ ENCODERS", "READ ULTRASONIC"] ("element") -> [w899] mode=indexing
                      n353 = Enqueue Element(queue=w901, element=w899) -> (queue out=w900:refnum<queue>)  [unwired: 2 in, 2 out]
                    }
                  }
                  frame True {
                    n354 = for {
                      shift-right: [w906] -> w903
                      shift-left: w902 -> [w907]
                      tunnel: string[] ["STOP", "RESET YAW", "RESET ENCODERS", "RESET FLAGS"] -> [w905] mode=indexing
                      n355 = Enqueue Element(queue=w907, element=w905) -> (queue out=w906:refnum<queue>)  [unwired: 2 in, 2 out]
                    }
                  }
                }
                n356 = Select(t=State_Type_Definitions."True Stop" ("Enum"), s=w886, f=State_Type_Definitions."True Stop" ("Enum")) -> (s? t:f=w887:T16)
                n357 = Select(t=w887, s=w891, f=State_Type_Definitions."Task 4_D" ("Enum")) -> (s? t:f=w895:T16)
              }
              frame "Exit" {
                n358 = for {
                  shift-right: [w914] -> w911
                  shift-left: w908 -> [w915]
                  tunnel: string[] ["STOP", "RESET ENCODERS", "RESET YAW", ""] -> [w913] mode=indexing
                  n359 = Enqueue Element(queue=w915, element=w913) -> (queue out=w914:refnum<queue>)  [unwired: 2 in, 2 out]
                }
              }
            }
          }
          frame 15 {
            # ">>> yStepper command>>>"
            # ">> Manual override >>"
            n360 = Dequeue Element(queue=w926, timeout in ms (-1)=w925, error in (no error)=w927) -> (element=w924:T8)  [unwired: 3 out]
            n361 = Equal?(x=w923, y=u8 60) -> (x = y?=w921:bool)
            n362 = case shown="\"Start Task 1\", Default" w924 {
              tunnel: [w937 State_Type_Definitions."True Stop" ("Enum")] -> w928
              tunnel: [w940 w957] -> w929
              tunnel: [State_Type_Definitions."Idle" ("Enum") State_Type_Definitions."Shutdown" ("Enum")] -> w930
              tunnel: w921 -> [w936 _]
              tunnel: w920 -> [w935 _]
              tunnel: w919 -> [w931 w954]
              frame "Start Task 1", Default {
                # "Stays in Task 5_A until stepper reaches desired \nheight"
                # "T: Go back to idle, F: Continue with task\""
                # ">> Manual override >>"
                n363 = case shown="True" w936 {
                  tunnel: [w944 w950] -> w940
                  tunnel: w931 -> [w942 w948]
                  frame False {
                    n364 = for {
                      tunnel: string[] ["Z STEPPER CAM HEIGHT", "READ STEPPER VALUES"] ("element") -> [w945] mode=indexing
                      shift-right: [w947] -> w944
                      shift-left: w942 -> [w946]
                      n365 = Enqueue Element(queue=w946, element=w945) -> (queue out=w947:refnum<queue>)  [unwired: 2 in, 2 out]
                    }
                  }
                  frame True {
                    n366 = for {
                      shift-right: [w952] -> w950
                      shift-left: w948 -> [w953]
                      tunnel: string[] ["ARDUINO - ULTRASONIC", "READ ULTRASONIC", ""] -> [w951] mode=indexing
                      n367 = Enqueue Element(queue=w953, element=w951) -> (queue out=w952:refnum<queue>)  [unwired: 2 in, 2 out]
                    }
                  }
                }
                n368 = Or(x=w936, y=w935) -> (x .or. y?=w938:bool)
                n369 = Select(t=State_Type_Definitions."True Stop" ("Enum"), s=w935, f=State_Type_Definitions."Task 5B: MOVE TO BOX" ("Enum")) -> (s? t:f=w932:u16)
                n370 = Select(t=w932, s=w938, f=State_Type_Definitions."Task 5A: ARM CAM HEIGHT" ("Enum")) -> (s? t:f=w937:u16)
              }
              frame "Exit" {
                n371 = for {
                  shift-right: [w960] -> w957
                  shift-left: w954 -> [w961]
                  tunnel: string[] ["STOP", "RESET ENCODERS", "RESET YAW", "ARDUINO MODE 0"] -> [w959] mode=indexing
                  n372 = Enqueue Element(queue=w961, element=w959) -> (queue out=w960:refnum<queue>)  [unwired: 2 in, 2 out]
                }
              }
            }
          }
          frame 16 {
            w969 = u8 20 ("y")
            # ">>> yStepper command>>>"
            n373 = Less?(x=w966, y=w969) -> (x < y?=w967:bool)
            n374 = Dequeue Element(queue=w973, timeout in ms (-1)=w972, error in (no error)=w974) -> (element=w971:T8)  [unwired: 3 out]
            n375 = Less?(x=w965, y=w969) -> (x < y?=w968:bool)
            n376 = And(x=w968, y=w967) -> (x .and. y?=w964:bool)
            n377 = case shown="\"Start Task 1\", Default" w971 {
              tunnel: [w986 State_Type_Definitions."True Stop" ("Enum")] -> w976
              tunnel: [w989 w1006] -> w975
              tunnel: [State_Type_Definitions."Idle" ("Enum") State_Type_Definitions."Shutdown" ("Enum")] -> w977
              tunnel: w979 -> [w985 _]
              tunnel: w978 -> [w981 w1003]
              tunnel: w964 -> [w980 _]
              frame "Start Task 1", Default {
                # "Stays in Task 5_B to capture image over 5 seconds"
                # "T: Go back to idle, F: Continue with task\""
                # ">> Manual override >>"
                n378 = case shown="True" w980 {
                  tunnel: [w993 w999] -> w989
                  tunnel: w981 -> [w991 w997]
                  frame False {
                    n379 = for {
                      tunnel: string[] ["FORWARD", "READ ULTRASONIC", "READ NAVX"] ("element") -> [w994] mode=indexing
                      shift-right: [w996] -> w993
                      shift-left: w991 -> [w995]
                      n380 = Enqueue Element(queue=w995, element=w994) -> (queue out=w996:refnum<queue>)  [unwired: 2 in, 2 out]
                    }
                  }
                  frame True {
                    n381 = for {
                      shift-right: [w1001] -> w999
                      shift-left: w997 -> [w1002]
                      tunnel: string[] ["STOP", "RESET ENCODERS", "OPEN LOG CAM", "SET TIMER 5"] -> [w1000] mode=indexing
                      n382 = Enqueue Element(queue=w1002, element=w1000) -> (queue out=w1001:refnum<queue>)  [unwired: 2 in, 2 out]
                    }
                  }
                }
                n383 = Or(x=w980, y=w985) -> (x .or. y?=w987:bool)
                n384 = Select(t=State_Type_Definitions."True Stop" ("Enum"), s=w985, f=State_Type_Definitions."Task 5C: CAM BURST" ("Enum")) -> (s? t:f=w982:u16)
                n385 = Select(t=w982, s=w987, f=State_Type_Definitions."Task 5B: MOVE TO BOX" ("Enum")) -> (s? t:f=w986:u16)
              }
              frame "Exit" {
                n386 = for {
                  shift-right: [w1009] -> w1006
                  shift-left: w1003 -> [w1010]
                  tunnel: string[] ["STOP", "RESET ENCODERS", "RESET YAW", "ARDUINO MODE 0"] -> [w1008] mode=indexing
                  n387 = Enqueue Element(queue=w1010, element=w1008) -> (queue out=w1009:refnum<queue>)  [unwired: 2 in, 2 out]
                }
              }
            }
          }
          frame 17 {
            # ">>> Motor control cluster >>>"
            # ">>> yStepper command>>>"
            # ">> Manual override >>"
            n388 = Dequeue Element(queue=w1021, timeout in ms (-1)=w1020, error in (no error)=w1019) -> (element=w1018:T8)  [unwired: 3 out]
            n389 = case shown="\"Start Task 1\", Default" w1018 {
              tunnel: [w1030 State_Type_Definitions."True Stop" ("Enum")] -> w1023
              tunnel: [w1033 w1050] -> w1016
              tunnel: [State_Type_Definitions."Idle" ("Enum") State_Type_Definitions."Shutdown" ("Enum")] -> w1015
              tunnel: w1017 -> [w1024 _]
              tunnel: w1022 -> [w1029 w1047]
              tunnel: w1013 -> [w1028 _]
              frame "Start Task 1", Default {
                # ">> Is time up? >>"
                # "Determines if object is in range to pick up"
                # ">> Manual override >>"
                n390 = case shown="False" w1028 {
                  tunnel: [w1037 w1043] -> w1033
                  tunnel: w1029 -> [w1035 w1041]
                  frame False {
                    n391 = for {
                      tunnel: string[] ["CAM ACQ", "START TIMER"] ("element") -> [w1038] mode=indexing
                      shift-right: [w1040] -> w1037
                      shift-left: w1035 -> [w1039]
                      n392 = Enqueue Element(queue=w1039, element=w1038) -> (queue out=w1040:refnum<queue>)  [unwired: 2 in, 2 out]
                    }
                  }
                  frame True {
                    n393 = for {
                      shift-right: [w1045] -> w1043
                      shift-left: w1041 -> [w1046]
                      tunnel: string[] ["CAM CLOSE", "PROCESS IMAGE", "SET TIMER 5"] -> [w1044] mode=indexing
                      n394 = Enqueue Element(queue=w1046, element=w1044) -> (queue out=w1045:refnum<queue>)  [unwired: 2 in, 2 out]
                    }
                  }
                }
                n395 = Or(x=w1028, y=w1024) -> (x .or. y?=w1031:bool)
                n396 = Select(t=State_Type_Definitions."True Stop" ("Enum"), s=w1024, f=State_Type_Definitions."Task 5D: PROCESS IMAGE" ("Enum")) -> (s? t:f=w1026:u16)
                n397 = Select(t=w1026, s=w1031, f=State_Type_Definitions."Task 5C: CAM BURST" ("Enum")) -> (s? t:f=w1030:u16)
              }
              frame "Exit" {
                n398 = for {
                  shift-right: [w1053] -> w1050
                  shift-left: w1047 -> [w1054]
                  tunnel: string[] ["STOP", "RESET ENCODERS", "RESET YAW", "ARDUINO MODE 0"] -> [w1052] mode=indexing
                  n399 = Enqueue Element(queue=w1054, element=w1052) -> (queue out=w1053:refnum<queue>)  [unwired: 2 in, 2 out]
                }
              }
            }
          }
          frame 18 {
            # ">>> yStepper command>>>"
            n400 = Dequeue Element(queue=w1062, timeout in ms (-1)=w1061, error in (no error)=w1060) -> (element=w1059:T8)  [unwired: 3 out]
            n401 = case shown="\"Exit\"" w1059 {
              tunnel: [w1074 State_Type_Definitions."True Stop" ("Enum")] -> w1066
              tunnel: [w1077 w1094] -> w1065
              tunnel: [State_Type_Definitions."Idle" ("Enum") State_Type_Definitions."Shutdown" ("Enum")] -> w1067
              tunnel: w1063 -> [w1073 _]
              tunnel: w1064 -> [w1069 w1091]
              tunnel: w1057 -> [w1068 _]
              frame "Start Task 1", Default {
                # ">> T: Breaks out of state loop; F: Stays in loop>>"
                # ">> Manual override >>"
                # ">> Checks if time is up>>"
                # "Stays in Task 5D until the object is detected"
                # "T: Go back to idle, F: Continue with task\""
                # ">> Manual override >>"
                n402 = case shown="True" w1068 {
                  tunnel: [w1081 w1087] -> w1077
                  tunnel: w1069 -> [w1079 w1085]
                  frame False {
                    n403 = for {
                      tunnel: string[] ["START TIMER", "PROCESS IMAGE", ""] ("element") -> [w1082] mode=indexing
                      shift-right: [w1084] -> w1081
                      shift-left: w1079 -> [w1083]
                      n404 = Enqueue Element(queue=w1083, element=w1082) -> (queue out=w1084:refnum<queue>)  [unwired: 2 in, 2 out]
                    }
                  }
                  frame True {
                    n405 = for {
                      shift-right: [w1089] -> w1087
                      shift-left: w1085 -> [w1090]
                      tunnel: string[] ["CAM CLOSE", "", ""] -> [w1088] mode=indexing
                      n406 = Enqueue Element(queue=w1090, element=w1088) -> (queue out=w1089:refnum<queue>)  [unwired: 2 in, 2 out]
                    }
                  }
                }
                n407 = Or(x=w1068, y=w1073) -> (x .or. y?=w1075:bool)
                n408 = Select(t=State_Type_Definitions."True Stop" ("Enum"), s=w1073, f=State_Type_Definitions."Task 5E: POSITION ARM" ("Enum")) -> (s? t:f=w1070:T16)
                n409 = Select(t=w1070, s=w1075, f=State_Type_Definitions."Task 5D: PROCESS IMAGE" ("Enum")) -> (s? t:f=w1074:u16)
              }
              frame "Exit" {
                n410 = for {
                  shift-right: [w1097] -> w1094
                  shift-left: w1091 -> [w1098]
                  tunnel: string[] ["STOP", "RESET ENCODERS", "RESET YAW", "ARDUINO MODE 0"] -> [w1096] mode=indexing
                  n411 = Enqueue Element(queue=w1098, element=w1096) -> (queue out=w1097:refnum<queue>)  [unwired: 2 in, 2 out]
                }
              }
            }
          }
          frame 20 {
            # ">>> yStepper command>>>"
            n412 = Dequeue Element(queue=w1112, timeout in ms (-1)=w1113, error in (no error)=w1114) -> (element=w1116:T8)  [unwired: 3 out]
            n413 = formula code="if (pos < 100)\ny = 41;\n\nelse if (pos >= 100 && pos <= 140)\ny = 30;\n\nelse if (pos >= 141 && pos <= 170)\ny = 25;\n\nelse if (pos >= 171 &&pos <= 180) \ny = 20;\n\nelse if (pos >= 181&& pos <= 200)\ny = 15;\n\nelse if (pos >= 201 && pos <= 230)\ny = 10;\n\nelse if (pos >= 231 && pos <= 320)\ny = 8;\n\nelse if (pos > 320)\ny = 0;"("pos"=w1104) -> ("y"=w1107:dbl)
            n414 = To Unsigned Byte Integer(number=w1107) -> (unsigned 8bit integer=w1102:u8)
            n415 = Equal?(x=w1103, y=w1102) -> (x = y?=w1101:bool)
            n416 = case shown="\"Start Task 1\", Default" w1116 {
              tunnel: [w1123 State_Type_Definitions."True Stop" ("Enum")] -> w1110
              tunnel: [w1126 w1143] -> w1108
              tunnel: [State_Type_Definitions."Idle" ("Enum") State_Type_Definitions."Shutdown" ("Enum")] -> w1109
              tunnel: w1115 -> [w1122 _]
              tunnel: w1111 -> [w1118 w1140]
              tunnel: w1101 -> [w1117 _]
              frame "Start Task 1", Default {
                # ">> T: Breaks out of state loop; F: Stays in loop>>"
                # ">> Manual override >>"
                # ">> Checks if time is up>>"
                # "Stays in Task 5D until the object is detected"
                # "T: Go back to idle, F: Continue with task\""
                # ">> Manual override >>"
                n417 = case shown="False" w1117 {
                  tunnel: [w1130 w1136] -> w1126
                  tunnel: w1118 -> [w1128 w1134]
                  frame False {
                    n418 = for {
                      tunnel: string[] ["READ STEPPER VALUES", "Y STEPPER CONTROL", ""] ("element") -> [w1131] mode=indexing
                      shift-right: [w1133] -> w1130
                      shift-left: w1128 -> [w1132]
                      n419 = Enqueue Element(queue=w1132, element=w1131) -> (queue out=w1133:refnum<queue>)  [unwired: 2 in, 2 out]
                    }
                  }
                  frame True {
                    n420 = for {
                      shift-right: [w1138] -> w1136
                      shift-left: w1134 -> [w1139]
                      tunnel: string[] ["CAM CLOSE", "DISPOSE BUFFERS", ""] -> [w1137] mode=indexing
                      n421 = Enqueue Element(queue=w1139, element=w1137) -> (queue out=w1138:refnum<queue>)  [unwired: 2 in, 2 out]
                    }
                  }
                }
                n422 = Or(x=w1117, y=w1122) -> (x .or. y?=w1124:bool)
                n423 = Select(t=State_Type_Definitions."True Stop" ("Enum"), s=w1122, f=State_Type_Definitions."Task 5F: ARM GRAB HEIGHT" ("Enum")) -> (s? t:f=w1119:T16)
                n424 = Select(t=w1119, s=w1124, f=State_Type_Definitions."Task 5E: POSITION ARM" ("Enum")) -> (s? t:f=w1123:T16)
              }
              frame "Exit" {
                n425 = for {
                  shift-right: [w1146] -> w1143
                  shift-left: w1140 -> [w1147]
                  tunnel: string[] ["STOP", "RESET ENCODERS", "RESET YAW", "ARDUINO MODE 0"] -> [w1145] mode=indexing
                  n426 = Enqueue Element(queue=w1147, element=w1145) -> (queue out=w1146:refnum<queue>)  [unwired: 2 in, 2 out]
                }
              }
            }
            n427 = Bundle By Name(cluster=w1106, "yStepper desired"=w1102) -> (w1105:T18)
          }
          frame 21 {
            # ">>> Motor control cluster >>>"
            # ">>> yStepper command>>>"
            # ">> Manual override >>"
            n428 = Dequeue Element(queue=w1158, timeout in ms (-1)=w1157, error in (no error)=w1159) -> (element=w1156:T8)  [unwired: 3 out]
            n429 = Equal?(x=w1155, y=u8 1) -> (x = y?=w1153:bool)
            n430 = case shown="\"Start Task 1\", Default" w1156 {
              tunnel: [w1169 State_Type_Definitions."True Stop" ("Enum")] -> w1160
              tunnel: [w1172 w1189] -> w1161
              tunnel: [State_Type_Definitions."Idle" ("Enum") State_Type_Definitions."Shutdown" ("Enum")] -> w1162
              tunnel: w1153 -> [w1168 _]
              tunnel: w1152 -> [w1167 _]
              tunnel: w1151 -> [w1163 w1186]
              frame "Start Task 1", Default {
                # "Stays in Task 5F until stepper reaches desired \nheight"
                # "T: Go back to idle, F: Continue with task\""
                # ">> Manual override >>"
                n431 = case shown="True" w1168 {
                  tunnel: [w1176 w1182] -> w1172
                  tunnel: w1163 -> [w1174 w1180]
                  frame False {
                    n432 = for {
                      tunnel: string[] ["Z STEPPER GRAB HEIGHT", "READ STEPPER VALUES"] ("element") -> [w1177] mode=indexing
                      shift-right: [w1179] -> w1176
                      shift-left: w1174 -> [w1178]
                      n433 = Enqueue Element(queue=w1178, element=w1177) -> (queue out=w1179:refnum<queue>)  [unwired: 2 in, 2 out]
                    }
                  }
                  frame True {
                    n434 = for {
                      shift-right: [w1184] -> w1182
                      shift-left: w1180 -> [w1185]
                      tunnel: string[] ["SET TIMER 5", "CLOSE CLAW", ""] -> [w1183] mode=indexing
                      n435 = Enqueue Element(queue=w1185, element=w1183) -> (queue out=w1184:refnum<queue>)  [unwired: 2 in, 2 out]
                    }
                  }
                }
                n436 = Or(x=w1168, y=w1167) -> (x .or. y?=w1170:bool)
                n437 = Select(t=State_Type_Definitions."True Stop" ("Enum"), s=w1167, f=State_Type_Definitions."Task 5G: CLOSE CLAW" ("Enum")) -> (s? t:f=w1164:T16)
                n438 = Select(t=w1164, s=w1170, f=State_Type_Definitions."Task 5F: ARM GRAB HEIGHT" ("Enum")) -> (s? t:f=w1169:T16)
              }
              frame "Exit" {
                n439 = for {
                  shift-right: [w1192] -> w1189
                  shift-left: w1186 -> [w1193]
                  tunnel: string[] ["STOP", "RESET ENCODERS", "RESET YAW", "ARDUINO MODE 0"] -> [w1191] mode=indexing
                  n440 = Enqueue Element(queue=w1193, element=w1191) -> (queue out=w1192:refnum<queue>)  [unwired: 2 in, 2 out]
                }
              }
            }
          }
          frame 22 {
            # ">>> yStepper command>>>"
            # ">> Manual override >>"
            n441 = Dequeue Element(queue=w1204, timeout in ms (-1)=w1203, error in (no error)=w1202) -> (element=w1201:T8)  [unwired: 3 out]
            n442 = case shown="\"Start Task 1\", Default" w1201 {
              tunnel: [w1213 State_Type_Definitions."True Stop" ("Enum")] -> w1206
              tunnel: [w1216 w1233] -> w1199
              tunnel: [State_Type_Definitions."Idle" ("Enum") State_Type_Definitions."Shutdown" ("Enum")] -> w1198
              tunnel: w1200 -> [w1207 _]
              tunnel: w1205 -> [w1212 w1230]
              tunnel: w1196 -> [w1211 _]
              frame "Start Task 1", Default {
                # ">> Is time up? >>"
                # "Determines if object is in range to pick up"
                # ">> Manual override >>"
                n443 = case shown="True" w1211 {
                  tunnel: [w1220 w1226] -> w1216
                  tunnel: w1212 -> [w1218 w1224]
                  frame False {
                    n444 = for {
                      tunnel: string[] ["CLOSE CLAW", "START TIMER"] ("element") -> [w1221] mode=indexing
                      shift-right: [w1223] -> w1220
                      shift-left: w1218 -> [w1222]
                      n445 = Enqueue Element(queue=w1222, element=w1221) -> (queue out=w1223:refnum<queue>)  [unwired: 2 in, 2 out]
                    }
                  }
                  frame True {
                    n446 = for {
                      shift-right: [w1228] -> w1226
                      shift-left: w1224 -> [w1229]
                      tunnel: string[] ["READ STEPPER VALUES", "", ""] -> [w1227] mode=indexing
                      n447 = Enqueue Element(queue=w1229, element=w1227) -> (queue out=w1228:refnum<queue>)  [unwired: 2 in, 2 out]
                    }
                  }
                }
                n448 = Or(x=w1211, y=w1207) -> (x .or. y?=w1214:bool)
                n449 = Select(t=State_Type_Definitions."True Stop" ("Enum"), s=w1207, f=State_Type_Definitions."Task 5H: RAISE ARM" ("Enum")) -> (s? t:f=w1209:T16)
                n450 = Select(t=w1209, s=w1214, f=State_Type_Definitions."Task 5G: CLOSE CLAW" ("Enum")) -> (s? t:f=w1213:T16)
              }
              frame "Exit" {
                n451 = for {
                  shift-right: [w1236] -> w1233
                  shift-left: w1230 -> [w1237]
                  tunnel: string[] ["STOP", "RESET ENCODERS", "RESET YAW", "ARDUINO MODE 0"] -> [w1235] mode=indexing
                  n452 = Enqueue Element(queue=w1237, element=w1235) -> (queue out=w1236:refnum<queue>)  [unwired: 2 in, 2 out]
                }
              }
            }
          }
          frame 23 {
            # ">>> yStepper command>>>"
            # ">> Manual override >>"
            n453 = Dequeue Element(queue=w1248, timeout in ms (-1)=w1247, error in (no error)=w1249) -> (element=w1246:T8)  [unwired: 3 out]
            n454 = Equal?(x=w1245, y=u8 60) -> (x = y?=w1243:bool)
            n455 = case shown="\"Start Task 1\", Default" w1246 {
              tunnel: [w1259 State_Type_Definitions."True Stop" ("Enum")] -> w1250
              tunnel: [w1262 w1279] -> w1251
              tunnel: [State_Type_Definitions."Idle" ("Enum") State_Type_Definitions."Shutdown" ("Enum")] -> w1252
              tunnel: w1243 -> [w1258 _]
              tunnel: w1242 -> [w1257 _]
              tunnel: w1241 -> [w1253 w1276]
              frame "Start Task 1", Default {
                # "Stays in Task 5_A until stepper reaches desired \nheight"
                # "T: Go back to idle, F: Continue with task\""
                # ">> Manual override >>"
                n456 = case shown="False" w1258 {
                  tunnel: [w1266 w1272] -> w1262
                  tunnel: w1253 -> [w1264 w1270]
                  frame False {
                    n457 = for {
                      tunnel: string[] ["Z STEPPER CAM HEIGHT", "READ STEPPER VALUES"] ("element") -> [w1267] mode=indexing
                      shift-right: [w1269] -> w1266
                      shift-left: w1264 -> [w1268]
                      n458 = Enqueue Element(queue=w1268, element=w1267) -> (queue out=w1269:refnum<queue>)  [unwired: 2 in, 2 out]
                    }
                  }
                  frame True {
                    n459 = for {
                      shift-right: [w1274] -> w1272
                      shift-left: w1270 -> [w1275]
                      tunnel: string[] ["ARDUINO - ULTRASONIC", "READ ULTRASONIC", ""] -> [w1273] mode=indexing
                      n460 = Enqueue Element(queue=w1275, element=w1273) -> (queue out=w1274:refnum<queue>)  [unwired: 2 in, 2 out]
                    }
                  }
                }
                n461 = Or(x=w1258, y=w1257) -> (x .or. y?=w1260:bool)
                n462 = Select(t=State_Type_Definitions."True Stop" ("Enum"), s=w1257, f=State_Type_Definitions."True Stop" ("Enum")) -> (s? t:f=w1254:T16)
                n463 = Select(t=w1254, s=w1260, f=State_Type_Definitions."Task 5H: RAISE ARM" ("Enum")) -> (s? t:f=w1259:T16)
              }
              frame "Exit" {
                n464 = for {
                  shift-right: [w1282] -> w1279
                  shift-left: w1276 -> [w1283]
                  tunnel: string[] ["STOP", "RESET ENCODERS", "RESET YAW", "ARDUINO MODE 0"] -> [w1281] mode=indexing
                  n465 = Enqueue Element(queue=w1283, element=w1281) -> (queue out=w1282:refnum<queue>)  [unwired: 2 in, 2 out]
                }
              }
            }
          }
          frame 24 {
            # ">>> yStepper command>>>"
            n466 = Dequeue Element(queue=w1293, timeout in ms (-1)=w1292, error in (no error)=w1291) -> (element=w1298:T8)  [unwired: 3 out]
            n467 = Equal?(x=w1289, y=u8 60) -> (x = y?=w1288:bool)
            n468 = case shown="\"Start Task 1\", Default" w1298 {
              tunnel: [w1305 State_Type_Definitions."True Stop" ("Enum")] -> w1296
              tunnel: [w1304 w1322] -> w1295
              tunnel: [State_Type_Definitions."Idle" ("Enum") State_Type_Definitions."Shutdown" ("Enum")] -> w1297
              tunnel: w1294 -> [w1300 _]
              tunnel: w1290 -> [w1302 _]
              tunnel: w1288 -> [w1299 _]
              frame "Start Task 1", Default {
                n469 = case shown="False" w1299 {
                  tunnel: [w1310 w1316] -> w1304
                  tunnel: w1302 -> [w1308 w1314]
                  frame False {
                    n470 = for {
                      tunnel: string[] ["Z STEPPER CAM HEIGHT", "READ STEPPER VALUES"] ("element") -> [w1311] mode=indexing
                      shift-right: [w1313] -> w1310
                      shift-left: w1308 -> [w1312]
                      n471 = Enqueue Element(queue=w1312, element=w1311) -> (queue out=w1313:refnum<queue>)  [unwired: 2 in, 2 out]
                    }
                  }
                  frame True {
                    n472 = for {
                      shift-right: [w1318] -> w1316
                      shift-left: w1314 -> [w1319]
                      tunnel: string[] ["CAM ACQ", "OPEN LOG CAM"] -> [w1317] mode=indexing
                      n473 = Enqueue Element(queue=w1319, element=w1317) -> (queue out=w1318:refnum<queue>)  [unwired: 2 in, 2 out]
                    }
                  }
                }
                n474 = Or(x=w1299, y=w1300) -> (x .or. y?=w1301:bool)
                n475 = Select(t=State_Type_Definitions."Task 6_B" ("Enum"), s=w1301, f=State_Type_Definitions."Task 6_A" ("Enum")) -> (s? t:f=w1305:T16)
              }
              frame "Exit" {
                n476 = for {
                  shift-right: [w1325] -> w1322
                  shift-left: _ -> [w1326]
                  tunnel: string[] ["STOP", "RESET ENCODERS", "RESET YAW", "ARDUINO MODE 0"] -> [w1324] mode=indexing
                  n477 = Enqueue Element(queue=w1326, element=w1324) -> (queue out=w1325:refnum<queue>)  [unwired: 2 in, 2 out]
                }
              }
            }
          }
          frame 25 {
            # ">>> yStepper command>>>"
            n478 = Dequeue Element(queue=w1338, timeout in ms (-1)=w1336, error in (no error)=w1337) -> (element=w1335:T8)  [unwired: 3 out]
            n479 = case shown="\"Start Task 1\", Default" w1335 {
              tunnel: [w1345 State_Type_Definitions."True Stop" ("Enum")] -> w1331
              tunnel: [w1344 w1363] -> w1339
              tunnel: [State_Type_Definitions."Idle" ("Enum") State_Type_Definitions."Shutdown" ("Enum")] -> w1332
              tunnel: w1334 -> [w1340 _]
              tunnel: w1333 -> [w1342 _]
              tunnel: w1330 -> [w1341 w1360]
              frame "Start Task 1", Default {
                # ">> Manual override >>"
                n480 = case shown="True" w1342 {
                  tunnel: [w1350 w1356] -> w1344
                  tunnel: w1341 -> [w1349 w1354]
                  frame False {
                    n481 = for {
                      shift-right: [w1353] -> w1350
                      shift-left: w1349 -> [w1352]
                      tunnel: string[] ["CAM ACQ", "PROCESS IMAGE", "OPEN CLAW"] -> [w1351] mode=indexing
                      n482 = Enqueue Element(queue=w1352, element=w1351) -> (queue out=w1353:refnum<queue>)  [unwired: 2 in, 2 out]
                    }
                  }
                  frame True {
                    n483 = for {
                      shift-right: [w1358] -> w1356
                      shift-left: w1354 -> [w1359]
                      tunnel: string[] ["CAM ACQ", "PROCESS IMAGE", "CLOSE CLAW"] -> [w1357] mode=indexing
                      n484 = Enqueue Element(queue=w1359, element=w1357) -> (queue out=w1358:refnum<queue>)  [unwired: 2 in, 2 out]
                    }
                  }
                }
                n485 = Select(t=State_Type_Definitions."True Stop" ("Enum"), s=w1340, f=State_Type_Definitions."Task 6_B" ("Enum")) -> (s? t:f=w1345:T16)
              }
              frame "Exit" {
                # ">> State after true stop >>"
                # ">> Goes to true stop >>"
                n486 = for {
                  shift-right: [w1366] -> w1363
                  shift-left: w1360 -> [w1367]
                  tunnel: string[] ["STOP", "RESET ENCODERS", "RESET YAW", ""] -> [w1365] mode=indexing
                  n487 = Enqueue Element(queue=w1367, element=w1365) -> (queue out=w1366:refnum<queue>)  [unwired: 2 in, 2 out]
                }
              }
            }
          }
          frame 26 {
          }
          frame 27 {
            # ">>> Motor control cluster >>>"
            # ">>> yStepper command>>>"
            # ">> Manual override >>"
            n488 = Dequeue Element(queue=w1384, timeout in ms (-1)=w1383, error in (no error)=w1385) -> (element=w1382:T8)  [unwired: 3 out]
            n489 = Equal?(x=w1381, y=u8 60) -> (x = y?=w1379:bool)
            n490 = case shown="\"Start Task 1\", Default" w1382 {
              tunnel: [w1395 State_Type_Definitions."True Stop" ("Enum")] -> w1386
              tunnel: [w1398 w1415] -> w1387
              tunnel: [State_Type_Definitions."Idle" ("Enum") State_Type_Definitions."Shutdown" ("Enum")] -> w1388
              tunnel: w1379 -> [w1394 _]
              tunnel: w1378 -> [w1393 _]
              tunnel: w1377 -> [w1389 w1412]
              frame "Start Task 1", Default {
                # "Stays in Task 5_A until stepper reaches desired \nheight"
                # "T: Go back to idle, F: Continue with task\""
                # ">> Manual override >>"
                n491 = case shown="False" w1394 {
                  tunnel: [w1402 w1408] -> w1398
                  tunnel: w1389 -> [w1400 w1406]
                  frame False {
                    n492 = for {
                      tunnel: string[] ["Z STEPPER CAM HEIGHT", "READ STEPPER VALUES"] ("element") -> [w1403] mode=indexing
                      shift-right: [w1405] -> w1402
                      shift-left: w1400 -> [w1404]
                      n493 = Enqueue Element(queue=w1404, element=w1403) -> (queue out=w1405:refnum<queue>)  [unwired: 2 in, 2 out]
                    }
                  }
                  frame True {
                    n494 = for {
                      shift-right: [w1410] -> w1408
                      shift-left: w1406 -> [w1411]
                      tunnel: string[] ["ARDUINO - ULTRASONIC", "READ ULTRASONIC", ""] -> [w1409] mode=indexing
                      n495 = Enqueue Element(queue=w1411, element=w1409) -> (queue out=w1410:refnum<queue>)  [unwired: 2 in, 2 out]
                    }
                  }
                }
                n496 = Or(x=w1394, y=w1393) -> (x .or. y?=w1396:bool)
                n497 = Select(t=State_Type_Definitions."True Stop" ("Enum"), s=w1393, f=State_Type_Definitions."Task 8B: MOVE TO BOX" ("Enum")) -> (s? t:f=w1390:T16)
                n498 = Select(t=w1390, s=w1396, f=State_Type_Definitions."Task 8A: RAISE ARM" ("Enum")) -> (s? t:f=w1395:T16)
              }
              frame "Exit" {
                n499 = for {
                  shift-right: [w1418] -> w1415
                  shift-left: w1412 -> [w1419]
                  tunnel: string[] ["STOP", "RESET ENCODERS", "RESET YAW", "ARDUINO MODE 0"] -> [w1417] mode=indexing
                  n500 = Enqueue Element(queue=w1419, element=w1417) -> (queue out=w1418:refnum<queue>)  [unwired: 2 in, 2 out]
                }
              }
            }
          }
          frame 28 {
            w1427 = u8 15 ("y")
            # ">>> yStepper command>>>"
            n501 = Less?(x=w1424, y=w1427) -> (x < y?=w1425:bool)
            n502 = Dequeue Element(queue=w1431, timeout in ms (-1)=w1430, error in (no error)=w1432) -> (element=w1429:T8)  [unwired: 3 out]
            n503 = Less?(x=w1423, y=w1427) -> (x < y?=w1426:bool)
            n504 = And(x=w1426, y=w1425) -> (x .and. y?=w1422:bool)
            n505 = case shown="\"Start Task 1\", Default" w1429 {
              tunnel: [w1444 State_Type_Definitions."True Stop" ("Enum")] -> w1434
              tunnel: [w1447 w1464] -> w1433
              tunnel: [State_Type_Definitions."Idle" ("Enum") State_Type_Definitions."Shutdown" ("Enum")] -> w1435
              tunnel: w1437 -> [w1443 _]
              tunnel: w1436 -> [w1439 w1461]
              tunnel: w1422 -> [w1438 _]
              frame "Start Task 1", Default {
                # "Stays in Task 5_B to capture image over 5 seconds"
                # "T: Go back to idle, F: Continue with task\""
                # ">> Manual override >>"
                n506 = case shown="True" w1438 {
                  tunnel: [w1451 w1457] -> w1447
                  tunnel: w1439 -> [w1449 w1455]
                  frame False {
                    n507 = for {
                      tunnel: string[] ["FORWARD", "READ ULTRASONIC", "READ NAVX"] ("element") -> [w1452] mode=indexing
                      shift-right: [w1454] -> w1451
                      shift-left: w1449 -> [w1453]
                      n508 = Enqueue Element(queue=w1453, element=w1452) -> (queue out=w1454:refnum<queue>)  [unwired: 2 in, 2 out]
                    }
                  }
                  frame True {
                    n509 = for {
                      shift-right: [w1459] -> w1457
                      shift-left: w1455 -> [w1460]
                      tunnel: string[] ["STOP", "RESET ENCODERS", "OPEN LOG CAM", "SET TIMER 2", "OPEN IMAQ REF"] -> [w1458] mode=indexing
                      n510 = Enqueue Element(queue=w1460, element=w1458) -> (queue out=w1459:refnum<queue>)  [unwired: 2 in, 2 out]
                    }
                  }
                }
                n511 = Or(x=w1438, y=w1443) -> (x .or. y?=w1445:bool)
                n512 = Select(t=State_Type_Definitions."True Stop" ("Enum"), s=w1443, f=State_Type_Definitions."Task 8C: CAM BURST" ("Enum")) -> (s? t:f=w1440:T16)
                n513 = Select(t=w1440, s=w1445, f=State_Type_Definitions."Task 8B: MOVE TO BOX" ("Enum")) -> (s? t:f=w1444:T16)
              }
              frame "Exit" {
                n514 = for {
                  shift-right: [w1467] -> w1464
                  shift-left: w1461 -> [w1468]
                  tunnel: string[] ["STOP", "RESET ENCODERS", "RESET YAW", "ARDUINO MODE 0"] -> [w1466] mode=indexing
                  n515 = Enqueue Element(queue=w1468, element=w1466) -> (queue out=w1467:refnum<queue>)  [unwired: 2 in, 2 out]
                }
              }
            }
          }
          frame 29 {
            # ">>> Motor control cluster >>>"
            # ">>> yStepper command>>>"
            # ">> Manual override >>"
            n516 = Dequeue Element(queue=w1479, timeout in ms (-1)=w1478, error in (no error)=w1477) -> (element=w1476:T8)  [unwired: 3 out]
            n517 = case shown="\"Start Task 1\", Default" w1476 {
              tunnel: [w1488 State_Type_Definitions."True Stop" ("Enum")] -> w1481
              tunnel: [w1491 w1508] -> w1474
              tunnel: [State_Type_Definitions."Idle" ("Enum") State_Type_Definitions."Shutdown" ("Enum")] -> w1473
              tunnel: w1475 -> [w1482 _]
              tunnel: w1480 -> [w1487 w1505]
              tunnel: w1471 -> [w1486 _]
              frame "Start Task 1", Default {
                # ">> Is time up? >>"
                # "Determines if object is in range to pick up"
                # ">> Manual override >>"
                n518 = case shown="True" w1486 {
                  tunnel: [w1495 w1501] -> w1491
                  tunnel: w1487 -> [w1493 w1499]
                  frame False {
                    n519 = for {
                      tunnel: string[] ["CAM ACQ", "START TIMER"] ("element") -> [w1496] mode=indexing
                      shift-right: [w1498] -> w1495
                      shift-left: w1493 -> [w1497]
                      n520 = Enqueue Element(queue=w1497, element=w1496) -> (queue out=w1498:refnum<queue>)  [unwired: 2 in, 2 out]
                    }
                  }
                  frame True {
                    n521 = for {
                      shift-right: [w1503] -> w1501
                      shift-left: w1499 -> [w1504]
                      tunnel: string[] ["CAM CLOSE", "PROCESS IMAGE", "SET TIMER 5"] -> [w1502] mode=indexing
                      n522 = Enqueue Element(queue=w1504, element=w1502) -> (queue out=w1503:refnum<queue>)  [unwired: 2 in, 2 out]
                    }
                  }
                }
                n523 = Or(x=w1486, y=w1482) -> (x .or. y?=w1489:bool)
                n524 = Select(t=State_Type_Definitions."True Stop" ("Enum"), s=w1482, f=State_Type_Definitions."Task 8D: PROCESS IMAGE" ("Enum")) -> (s? t:f=w1484:T16)
                n525 = Select(t=w1484, s=w1489, f=State_Type_Definitions."Task 8C: CAM BURST" ("Enum")) -> (s? t:f=w1488:T16)
              }
              frame "Exit" {
                n526 = for {
                  shift-right: [w1511] -> w1508
                  shift-left: w1505 -> [w1512]
                  tunnel: string[] ["STOP", "RESET ENCODERS", "RESET YAW", "ARDUINO MODE 0"] -> [w1510] mode=indexing
                  n527 = Enqueue Element(queue=w1512, element=w1510) -> (queue out=w1511:refnum<queue>)  [unwired: 2 in, 2 out]
                }
              }
            }
          }
          frame 30 {
            # ">>> yStepper command>>>"
            n528 = Dequeue Element(queue=w1520, timeout in ms (-1)=w1519, error in (no error)=w1518) -> (element=w1517:T8)  [unwired: 3 out]
            n529 = case shown="\"Start Task 1\", Default" w1517 {
              tunnel: [w1532 State_Type_Definitions."True Stop" ("Enum")] -> w1524
              tunnel: [w1535 w1552] -> w1523
              tunnel: [State_Type_Definitions."Idle" ("Enum") State_Type_Definitions."Shutdown" ("Enum")] -> w1525
              tunnel: w1521 -> [w1531 _]
              tunnel: w1522 -> [w1527 w1549]
              tunnel: w1515 -> [w1526 _]
              frame "Start Task 1", Default {
                # ">> T: Breaks out of state loop; F: Stays in loop>>"
                # ">> Manual override >>"
                # ">> Checks if time is up>>"
                # "Stays in Task 5D until the object is detected"
                # "T: Go back to idle, F: Continue with task\""
                # ">> Manual override >>"
                n530 = case shown="True" w1526 {
                  tunnel: [w1539 w1545] -> w1535
                  tunnel: w1527 -> [w1537 w1543]
                  frame False {
                    n531 = for {
                      tunnel: string[] ["START TIMER", "PROCESS IMAGE", ""] ("element") -> [w1540] mode=indexing
                      shift-right: [w1542] -> w1539
                      shift-left: w1537 -> [w1541]
                      n532 = Enqueue Element(queue=w1541, element=w1540) -> (queue out=w1542:refnum<queue>)  [unwired: 2 in, 2 out]
                    }
                  }
                  frame True {
                    n533 = for {
                      shift-right: [w1547] -> w1545
                      shift-left: w1543 -> [w1548]
                      tunnel: string[] ["RESET ENCODERS", "", ""] -> [w1546] mode=indexing
                      n534 = Enqueue Element(queue=w1548, element=w1546) -> (queue out=w1547:refnum<queue>)  [unwired: 2 in, 2 out]
                    }
                  }
                }
                n535 = Or(x=w1526, y=w1531) -> (x .or. y?=w1533:bool)
                n536 = Select(t=State_Type_Definitions."True Stop" ("Enum"), s=w1531, f=State_Type_Definitions."Task 8E: ROBOT ADJUST" ("Enum")) -> (s? t:f=w1528:T16)
                n537 = Select(t=w1528, s=w1533, f=State_Type_Definitions."Task 8D: PROCESS IMAGE" ("Enum")) -> (s? t:f=w1532:T16)
              }
              frame "Exit" {
                n538 = for {
                  shift-right: [w1555] -> w1552
                  shift-left: w1549 -> [w1556]
                  tunnel: string[] ["STOP", "RESET ENCODERS", "RESET YAW", "ARDUINO MODE 0"] -> [w1554] mode=indexing
                  n539 = Enqueue Element(queue=w1556, element=w1554) -> (queue out=w1555:refnum<queue>)  [unwired: 2 in, 2 out]
                }
              }
            }
          }
          frame 31 {
            # ">>> Motor control cluster >>>"
            # ">>> yStepper command>>>"
            n540 = Dequeue Element(queue=w1573, timeout in ms (-1)=w1572, error in (no error)=w1571) -> (element=w1570:T8)  [unwired: 3 out]
            n541 = Subtract(x=w1568, y=300.0) -> (x-y=w1566:dbl)
            "x-y" <- w1566
            n542 = formula code="if (error <= -61&&error > -300){\ndistance = -15;\nxSpeed = -30;\n}\n\nelse if (error <= -51 && error >= -60){\ndistance = -10;\nxSpeed = -30;\n}\n\nelse if (error >= -50 && error <= 50){\ndistance = 0;\nxSpeed = 0;\n}\n\nelse if (error >= 51 && error <= 80){\ndistance = 10;\nxSpeed = 30;\n}\n\nelse if (error >= 81 && error <= 100){\ndistance = 15;\nxSpeed = 30;\n}\n\nelse if (error >= 101 && error <= 120){\ndistance = 20;\nxSpeed = 30;\n}\n\nelse if (error >= 121 && error < 300){\ndistance = 25;\nxSpeed = 30;\n}\n\nelse{\ndistance = 0;\nxSpeed = 0;\n}"("error"=w1566) -> ("distance"=w1561:dbl, "xSpeed"=w1563:dbl)
            n543 = formula code="if (target > 0){\nif (current  >= target)\noutput = 1;\n\nelse if (current != target)\noutput = 0;\n}\n\nelse if (target == 0){\nif (current == target)\noutput = 1;\n\nelse if (current != target)\noutput = 0;\n}\n\nelse if (target < 0){\nif (current <= target)\noutput = 1;\n\nelse if (current != target)\noutput = 0;\n}\n\nelse if (current != target)\noutput = 0;"("target"=w1561, "current"=w1562) -> ("output"=w1560:dbl)
            n544 = Bundle By Name(cluster=w1565, "xSpeed"=w1563) -> (w1564:T17)
            n545 = Equal?(x=w1560, y=1.0) -> (x = y?=w1558:bool)
            n546 = case shown="\"Start Task 1\", Default" w1570 {
              tunnel: [w1585 State_Type_Definitions."True Stop" ("Enum")] -> w1577
              tunnel: [w1588 w1605] -> w1576
              tunnel: [State_Type_Definitions."Idle" ("Enum") State_Type_Definitions."Shutdown" ("Enum")] -> w1578
              tunnel: w1574 -> [w1584 _]
              tunnel: w1575 -> [w1580 w1602]
              tunnel: w1558 -> [w1579 _]
              frame "Start Task 1", Default {
                # ">> T: Breaks out of state loop; F: Stays in loop>>"
                # ">> Manual override >>"
                # ">> Checks if time is up>>"
                # "Stays in Task 5D until the object is detected"
                # "T: Go back to idle, F: Continue with task\""
                # ">> Manual override >>"
                n547 = case shown="True" w1579 {
                  tunnel: [w1592 w1598] -> w1588
                  tunnel: w1580 -> [w1590 w1596]
                  frame False {
                    n548 = for {
                      tunnel: string[] ["X AXIS - SLOW", "READ ENCODERS", "READ NAVX"] ("element") -> [w1593] mode=indexing
                      shift-right: [w1595] -> w1592
                      shift-left: w1590 -> [w1594]
                      n549 = Enqueue Element(queue=w1594, element=w1593) -> (queue out=w1595:refnum<queue>)  [unwired: 2 in, 2 out]
                    }
                  }
                  frame True {
                    n550 = for {
                      shift-right: [w1600] -> w1598
                      shift-left: w1596 -> [w1601]
                      tunnel: string[] ["SET TIMER 2", "STOP", "READ STEPPER VALUES", ""] -> [w1599] mode=indexing
                      n551 = Enqueue Element(queue=w1601, element=w1599) -> (queue out=w1600:refnum<queue>)  [unwired: 2 in, 2 out]
                    }
                  }
                }
                n552 = Or(x=w1579, y=w1584) -> (x .or. y?=w1586:bool)
                n553 = Select(t=State_Type_Definitions."True Stop" ("Enum"), s=w1584, f=State_Type_Definitions."Task 8H: ARM ADJUST" ("Enum")) -> (s? t:f=w1581:T16)
                n554 = Select(t=w1581, s=w1586, f=State_Type_Definitions."Task 8E: ROBOT ADJUST" ("Enum")) -> (s? t:f=w1585:T16)
              }
              frame "Exit" {
                n555 = for {
                  shift-right: [w1608] -> w1605
                  shift-left: w1602 -> [w1609]
                  tunnel: string[] ["STOP", "RESET ENCODERS", "RESET YAW", "ARDUINO MODE 0"] -> [w1607] mode=indexing
                  n556 = Enqueue Element(queue=w1609, element=w1607) -> (queue out=w1608:refnum<queue>)  [unwired: 2 in, 2 out]
                }
              }
            }
          }
          frame 32 {
            # ">>> Motor control cluster >>>"
            # ">>> yStepper command>>>"
            # ">> Manual override >>"
            n557 = Dequeue Element(queue=w1620, timeout in ms (-1)=w1619, error in (no error)=w1618) -> (element=w1617:T8)  [unwired: 3 out]
            n558 = case shown="\"Start Task 1\", Default" w1617 {
              tunnel: [w1629 State_Type_Definitions."True Stop" ("Enum")] -> w1622
              tunnel: [w1632 w1649] -> w1615
              tunnel: [State_Type_Definitions."Idle" ("Enum") State_Type_Definitions."Shutdown" ("Enum")] -> w1614
              tunnel: w1616 -> [w1623 _]
              tunnel: w1621 -> [w1628 w1646]
              tunnel: w1612 -> [w1627 _]
              frame "Start Task 1", Default {
                # ">> Is time up? >>"
                # "Determines if object is in range to pick up"
                # ">> Manual override >>"
                n559 = case shown="False" w1627 {
                  tunnel: [w1636 w1642] -> w1632
                  tunnel: w1628 -> [w1634 w1640]
                  frame False {
                    n560 = for {
                      tunnel: string[] ["CAM ACQ", "START TIMER"] ("element") -> [w1637] mode=indexing
                      shift-right: [w1639] -> w1636
                      shift-left: w1634 -> [w1638]
                      n561 = Enqueue Element(queue=w1638, element=w1637) -> (queue out=w1639:refnum<queue>)  [unwired: 2 in, 2 out]
                    }
                  }
                  frame True {
                    n562 = for {
                      shift-right: [w1644] -> w1642
                      shift-left: w1640 -> [w1645]
                      tunnel: string[] ["CAM CLOSE", "PROCESS IMAGE", "SET TIMER 3"] -> [w1643] mode=indexing
                      n563 = Enqueue Element(queue=w1645, element=w1643) -> (queue out=w1644:refnum<queue>)  [unwired: 2 in, 2 out]
                    }
                  }
                }
                n564 = Or(x=w1627, y=w1623) -> (x .or. y?=w1630:bool)
                n565 = Select(t=State_Type_Definitions."True Stop" ("Enum"), s=w1623, f=State_Type_Definitions."Task 8G: PROCESS IMAGE 2" ("Enum")) -> (s? t:f=w1625:T16)
                n566 = Select(t=w1625, s=w1630, f=State_Type_Definitions."Task 8F: CAM BURST 2" ("Enum")) -> (s? t:f=w1629:T16)
              }
              frame "Exit" {
                n567 = for {
                  shift-right: [w1652] -> w1649
                  shift-left: w1646 -> [w1653]
                  tunnel: string[] ["STOP", "RESET ENCODERS", "RESET YAW", "ARDUINO MODE 0"] -> [w1651] mode=indexing
                  n568 = Enqueue Element(queue=w1653, element=w1651) -> (queue out=w1652:refnum<queue>)  [unwired: 2 in, 2 out]
                }
              }
            }
          }
          frame 33 {
            # ">>> yStepper command>>>"
            n569 = Dequeue Element(queue=w1661, timeout in ms (-1)=w1660, error in (no error)=w1659) -> (element=w1658:T8)  [unwired: 3 out]
            n570 = case shown="\"Start Task 1\", Default" w1658 {
              tunnel: [w1673 State_Type_Definitions."True Stop" ("Enum")] -> w1665
              tunnel: [w1676 w1693] -> w1664
              tunnel: [State_Type_Definitions."Idle" ("Enum") State_Type_Definitions."Shutdown" ("Enum")] -> w1666
              tunnel: w1662 -> [w1672 _]
              tunnel: w1663 -> [w1668 w1690]
              tunnel: w1656 -> [w1667 _]
              frame "Start Task 1", Default {
                # ">> T: Breaks out of state loop; F: Stays in loop>>"
                # ">> Manual override >>"
                # ">> Checks if time is up>>"
                # "Stays in Task 5D until the object is detected"
                # "T: Go back to idle, F: Continue with task\""
                # ">> Manual override >>"
                n571 = case shown="False" w1667 {
                  tunnel: [w1680 w1686] -> w1676
                  tunnel: w1668 -> [w1678 w1684]
                  frame False {
                    n572 = for {
                      tunnel: string[] ["START TIMER", "PROCESS IMAGE", ""] ("element") -> [w1681] mode=indexing
                      shift-right: [w1683] -> w1680
                      shift-left: w1678 -> [w1682]
                      n573 = Enqueue Element(queue=w1682, element=w1681) -> (queue out=w1683:refnum<queue>)  [unwired: 2 in, 2 out]
                    }
                  }
                  frame True {
                    n574 = for {
                      shift-right: [w1688] -> w1686
                      shift-left: w1684 -> [w1689]
                      tunnel: string[] ["READ STEPPER VALUES", "Y STEPPER CONTROL", ""] -> [w1687] mode=indexing
                      n575 = Enqueue Element(queue=w1689, element=w1687) -> (queue out=w1688:refnum<queue>)  [unwired: 2 in, 2 out]
                    }
                  }
                }
                n576 = Or(x=w1667, y=w1672) -> (x .or. y?=w1674:bool)
                n577 = Select(t=State_Type_Definitions."True Stop" ("Enum"), s=w1672, f=State_Type_Definitions."Task 8H: ARM ADJUST" ("Enum")) -> (s? t:f=w1669:T16)
                n578 = Select(t=w1669, s=w1674, f=State_Type_Definitions."Task 8G: PROCESS IMAGE 2" ("Enum")) -> (s? t:f=w1673:T16)
              }
              frame "Exit" {
                n579 = for {
                  shift-right: [w1696] -> w1693
                  shift-left: w1690 -> [w1697]
                  tunnel: string[] ["STOP", "RESET ENCODERS", "RESET YAW", "ARDUINO MODE 0"] -> [w1695] mode=indexing
                  n580 = Enqueue Element(queue=w1697, element=w1695) -> (queue out=w1696:refnum<queue>)  [unwired: 2 in, 2 out]
                }
              }
            }
          }
          frame 34 {
            # ">>> yStepper command>>>"
            n581 = Dequeue Element(queue=w1711, timeout in ms (-1)=w1712, error in (no error)=w1713) -> (element=w1715:T8)  [unwired: 3 out]
            n582 = formula code="if (pos < 70)\ny = 43;\n\nelse if (pos >= 71 &&pos <= 80)\ny = 40;\n\nelse if (pos >= 81 && pos <= 90)\ny = 38;\n\nelse if (pos >= 91 &&pos <= 120)\ny = 35;\n\nelse if (pos >= 121 && pos <= 140)\ny = 30;\n\nelse if (pos >= 141 && pos <= 170)\ny = 26;\n\nelse if (pos >= 171 &&pos <= 220) \ny = 20;\n\nelse if (pos >= 221&& pos <= 240)\ny = 15;\n\nelse if (pos >= 241 && pos <= 250)\ny = 10;\n\nelse if (pos >= 251)\ny = 0;"("pos"=w1703) -> ("y"=w1706:dbl)
            n583 = To Unsigned Byte Integer(number=w1706) -> (unsigned 8bit integer=w1701:u8)
            "Correcte stepper" <- w1701
            n584 = Equal?(x=w1702, y=w1701) -> (x = y?=w1700:bool)
            n585 = case shown="\"Start Task 1\", Default" w1715 {
              tunnel: [w1722 State_Type_Definitions."True Stop" ("Enum")] -> w1709
              tunnel: [w1725 w1742] -> w1707
              tunnel: [State_Type_Definitions."Idle" ("Enum") State_Type_Definitions."Shutdown" ("Enum")] -> w1708
              tunnel: w1714 -> [w1721 _]
              tunnel: w1710 -> [w1717 w1739]
              tunnel: w1700 -> [w1716 _]
              frame "Start Task 1", Default {
                # ">> T: Breaks out of state loop; F: Stays in loop>>"
                # ">> Manual override >>"
                # ">> Checks if time is up>>"
                # "Stays in Task 5D until the object is detected"
                # "T: Go back to idle, F: Continue with task\""
                # ">> Manual override >>"
                n586 = case shown="False" w1716 {
                  tunnel: [w1729 w1735] -> w1725
                  tunnel: w1717 -> [w1727 w1733]
                  frame False {
                    n587 = for {
                      tunnel: string[] ["READ STEPPER VALUES", "Y STEPPER CONTROL", ""] ("element") -> [w1730] mode=indexing
                      shift-right: [w1732] -> w1729
                      shift-left: w1727 -> [w1731]
                      n588 = Enqueue Element(queue=w1731, element=w1730) -> (queue out=w1732:refnum<queue>)  [unwired: 2 in, 2 out]
                    }
                  }
                  frame True {
                    n589 = for {
                      shift-right: [w1737] -> w1735
                      shift-left: w1733 -> [w1738]
                      tunnel: string[] ["DISPOSE BUFFERS", "READ STEPPER VALUES", ""] -> [w1736] mode=indexing
                      n590 = Enqueue Element(queue=w1738, element=w1736) -> (queue out=w1737:refnum<queue>)  [unwired: 2 in, 2 out]
                    }
                  }
                }
                n591 = Or(x=w1716, y=w1721) -> (x .or. y?=w1723:bool)
                n592 = Select(t=State_Type_Definitions."True Stop" ("Enum"), s=w1721, f=State_Type_Definitions."Task 8I: ARM GRAB HEIGHT" ("Enum")) -> (s? t:f=w1718:T16)
                n593 = Select(t=w1718, s=w1723, f=State_Type_Definitions."Task 8H: ARM ADJUST" ("Enum")) -> (s? t:f=w1722:T16)
              }
              frame "Exit" {
                n594 = for {
                  shift-right: [w1745] -> w1742
                  shift-left: w1739 -> [w1746]
                  tunnel: string[] ["STOP", "RESET ENCODERS", "RESET YAW", "ARDUINO MODE 0"] -> [w1744] mode=indexing
                  n595 = Enqueue Element(queue=w1746, element=w1744) -> (queue out=w1745:refnum<queue>)  [unwired: 2 in, 2 out]
                }
              }
            }
            n596 = Bundle By Name(cluster=w1705, "yStepper desired"=w1701) -> (w1704:T18)
          }
          frame 35 {
            # ">>> Motor control cluster >>>"
            # ">>> yStepper command>>>"
            # ">> Manual override >>"
            n597 = Dequeue Element(queue=w1757, timeout in ms (-1)=w1756, error in (no error)=w1758) -> (element=w1755:T8)  [unwired: 3 out]
            n598 = Equal?(x=w1754, y=u8 1) -> (x = y?=w1752:bool)
            n599 = case shown="\"Start Task 1\", Default" w1755 {
              tunnel: [w1768 State_Type_Definitions."True Stop" ("Enum")] -> w1759
              tunnel: [w1771 w1788] -> w1760
              tunnel: [State_Type_Definitions."Idle" ("Enum") State_Type_Definitions."Shutdown" ("Enum")] -> w1761
              tunnel: w1752 -> [w1767 _]
              tunnel: w1751 -> [w1766 _]
              tunnel: w1750 -> [w1762 w1785]
              frame "Start Task 1", Default {
                # "Stays in Task 5F until stepper reaches desired \nheight"
                # "T: Go back to idle, F: Continue with task\""
                # ">> Manual override >>"
                n600 = case shown="True" w1767 {
                  tunnel: [w1775 w1781] -> w1771
                  tunnel: w1762 -> [w1773 w1779]
                  frame False {
                    n601 = for {
                      tunnel: string[] ["Z STEPPER GRAB HEIGHT", "READ STEPPER VALUES"] ("element") -> [w1776] mode=indexing
                      shift-right: [w1778] -> w1775
                      shift-left: w1773 -> [w1777]
                      n602 = Enqueue Element(queue=w1777, element=w1776) -> (queue out=w1778:refnum<queue>)  [unwired: 2 in, 2 out]
                    }
                  }
                  frame True {
                    n603 = for {
                      shift-right: [w1783] -> w1781
                      shift-left: w1779 -> [w1784]
                      tunnel: string[] ["SET TIMER 2", "CLOSE CLAW", ""] -> [w1782] mode=indexing
                      n604 = Enqueue Element(queue=w1784, element=w1782) -> (queue out=w1783:refnum<queue>)  [unwired: 2 in, 2 out]
                    }
                  }
                }
                n605 = Or(x=w1767, y=w1766) -> (x .or. y?=w1769:bool)
                n606 = Select(t=State_Type_Definitions."True Stop" ("Enum"), s=w1766, f=State_Type_Definitions."Task 8J: CLOSE CLAW" ("Enum")) -> (s? t:f=w1763:T16)
                n607 = Select(t=w1763, s=w1769, f=State_Type_Definitions."Task 8I: ARM GRAB HEIGHT" ("Enum")) -> (s? t:f=w1768:T16)
              }
              frame "Exit" {
                n608 = for {
                  shift-right: [w1791] -> w1788
                  shift-left: w1785 -> [w1792]
                  tunnel: string[] ["STOP", "RESET ENCODERS", "RESET YAW", "ARDUINO MODE 0"] -> [w1790] mode=indexing
                  n609 = Enqueue Element(queue=w1792, element=w1790) -> (queue out=w1791:refnum<queue>)  [unwired: 2 in, 2 out]
                }
              }
            }
          }
          frame 36 {
            # ">>> yStepper command>>>"
            # ">> Manual override >>"
            n610 = Dequeue Element(queue=w1803, timeout in ms (-1)=w1802, error in (no error)=w1801) -> (element=w1800:T8)  [unwired: 3 out]
            n611 = case shown="\"Start Task 1\", Default" w1800 {
              tunnel: [w1812 State_Type_Definitions."True Stop" ("Enum")] -> w1805
              tunnel: [w1815 w1832] -> w1798
              tunnel: [State_Type_Definitions."Idle" ("Enum") State_Type_Definitions."Shutdown" ("Enum")] -> w1797
              tunnel: w1799 -> [w1806 _]
              tunnel: w1804 -> [w1811 w1829]
              tunnel: w1795 -> [w1810 _]
              frame "Start Task 1", Default {
                # ">> Is time up? >>"
                # "Determines if object is in range to pick up"
                # ">> Manual override >>"
                n612 = case shown="True" w1810 {
                  tunnel: [w1819 w1825] -> w1815
                  tunnel: w1811 -> [w1817 w1823]
                  frame False {
                    n613 = for {
                      tunnel: string[] ["CLOSE CLAW", "START TIMER"] ("element") -> [w1820] mode=indexing
                      shift-right: [w1822] -> w1819
                      shift-left: w1817 -> [w1821]
                      n614 = Enqueue Element(queue=w1821, element=w1820) -> (queue out=w1822:refnum<queue>)  [unwired: 2 in, 2 out]
                    }
                  }
                  frame True {
                    n615 = for {
                      shift-right: [w1827] -> w1825
                      shift-left: w1823 -> [w1828]
                      tunnel: string[] ["READ STEPPER VALUES", "", ""] -> [w1826] mode=indexing
                      n616 = Enqueue Element(queue=w1828, element=w1826) -> (queue out=w1827:refnum<queue>)  [unwired: 2 in, 2 out]
                    }
                  }
                }
                n617 = Or(x=w1810, y=w1806) -> (x .or. y?=w1813:bool)
                n618 = Select(t=State_Type_Definitions."True Stop" ("Enum"), s=w1806, f=State_Type_Definitions."Task 8K: RAISE MY SWORD" ("Enum")) -> (s? t:f=w1808:T16)
                n619 = Select(t=w1808, s=w1813, f=State_Type_Definitions."Task 8J: CLOSE CLAW" ("Enum")) -> (s? t:f=w1812:T16)
              }
              frame "Exit" {
                n620 = for {
                  shift-right: [w1835] -> w1832
                  shift-left: w1829 -> [w1836]
                  tunnel: string[] ["STOP", "RESET ENCODERS", "RESET YAW", "ARDUINO MODE 0"] -> [w1834] mode=indexing
                  n621 = Enqueue Element(queue=w1836, element=w1834) -> (queue out=w1835:refnum<queue>)  [unwired: 2 in, 2 out]
                }
              }
            }
          }
          frame 37 {
            # ">>> yStepper command>>>"
            # ">> Manual override >>"
            n622 = Dequeue Element(queue=w1847, timeout in ms (-1)=w1846, error in (no error)=w1848) -> (element=w1845:T8)  [unwired: 3 out]
            n623 = Equal?(x=w1844, y=u8 60) -> (x = y?=w1842:bool)
            n624 = case shown="\"Start Task 1\", Default" w1845 {
              tunnel: [w1858 State_Type_Definitions."True Stop" ("Enum")] -> w1849
              tunnel: [w1861 w1878] -> w1850
              tunnel: [State_Type_Definitions."Idle" ("Enum") State_Type_Definitions."Shutdown" ("Enum")] -> w1851
              tunnel: w1842 -> [w1857 _]
              tunnel: w1841 -> [w1856 _]
              tunnel: w1840 -> [w1852 w1875]
              frame "Start Task 1", Default {
                # "Stays in Task 5_A until stepper reaches desired \nheight"
                # "T: Go back to idle, F: Continue with task\""
                # ">> Manual override >>"
                n625 = case shown="True" w1857 {
                  tunnel: [w1865 w1871] -> w1861
                  tunnel: w1852 -> [w1863 w1869]
                  frame False {
                    n626 = for {
                      tunnel: string[] ["Z STEPPER CAM HEIGHT", "READ STEPPER VALUES"] ("element") -> [w1866] mode=indexing
                      shift-right: [w1868] -> w1865
                      shift-left: w1863 -> [w1867]
                      n627 = Enqueue Element(queue=w1867, element=w1866) -> (queue out=w1868:refnum<queue>)  [unwired: 2 in, 2 out]
                    }
                  }
                  frame True {
                    n628 = for {
                      shift-right: [w1873] -> w1871
                      shift-left: w1869 -> [w1874]
                      tunnel: string[] ["CAM CLOSE", "DISPOSE CAM BUFFERS", "DISPOSE PROC BUFFERS", "RESET ENCODERS"] -> [w1872] mode=indexing
                      n629 = Enqueue Element(queue=w1874, element=w1872) -> (queue out=w1873:refnum<queue>)  [unwired: 2 in, 2 out]
                    }
                  }
                }
                n630 = Or(x=w1857, y=w1856) -> (x .or. y?=w1859:bool)
                n631 = Select(t=State_Type_Definitions."True Stop" ("Enum"), s=w1856, f=State_Type_Definitions."True Stop" ("Enum")) -> (s? t:f=w1853:T16)
                n632 = Select(t=w1853, s=w1859, f=State_Type_Definitions."Task 8K: RAISE MY SWORD" ("Enum")) -> (s? t:f=w1858:T16)
              }
              frame "Exit" {
                n633 = for {
                  shift-right: [w1881] -> w1878
                  shift-left: w1875 -> [w1882]
                  tunnel: string[] ["STOP", "RESET ENCODERS", "RESET YAW", "ARDUINO MODE 0"] -> [w1880] mode=indexing
                  n634 = Enqueue Element(queue=w1882, element=w1880) -> (queue out=w1881:refnum<queue>)  [unwired: 2 in, 2 out]
                }
              }
            }
          }
          frame 38 {
            # ">>> Motor control cluster >>>"
            # ">> Stepper height reeached >>"
            # ">>> yStepper command>>>"
            # ">> Manual override >>"
            n635 = Dequeue Element(queue=w1894, timeout in ms (-1)=w1889, error in (no error)=w1893) -> (element=w1897:T8)  [unwired: 3 out]
            n636 = Equal?(x=w1891, y=u8 40) -> (x = y?=w1895:bool)
            n637 = case shown="\"Start Task 1\", Default" w1897 {
              tunnel: [w1908 State_Type_Definitions."True Stop" ("Enum")] -> w1887
              tunnel: [w1906 w1923] -> w1886
              tunnel: w1890 -> [w1905 _]
              tunnel: w1892 -> [w1899 _]
              tunnel: [State_Type_Definitions."Idle" ("Enum") State_Type_Definitions."Shutdown" ("Enum")] -> w1888
              tunnel: w1895 -> [w1898 _]
              frame "Start Task 1", Default {
                # ">> WIill proceed to part ii if not manual override >>"
                # ">>If ENABLE or Trigger is set to true>>"
                n638 = Or(x=w1898, y=w1899) -> (x .or. y?=w1900:bool)
                n639 = case shown="True" w1898 {
                  tunnel: [w1911 w1917] -> w1906
                  tunnel: w1905 -> [w1910 w1916]
                  frame False {
                    n640 = for {
                      shift-right: [w1913] -> w1911
                      shift-left: w1910 -> [w1914]
                      tunnel: string[] ["Z STEPPER BOX HEIGHT", "READ STEPPER VALUES"] ("element") -> [w1912] mode=indexing
                      n641 = Enqueue Element(queue=w1914, element=w1912) -> (queue out=w1913:refnum<queue>)  [unwired: 2 in, 2 out]
                    }
                  }
                  frame True {
                    n642 = for {
                      shift-right: [w1919] -> w1917
                      shift-left: w1916 -> [w1920]
                      tunnel: string[] ["ARDUINO - ULTRASONIC", "READ NAVX", "RESET FLAGS", "", "", ""] -> [w1918] mode=indexing
                      n643 = Enqueue Element(queue=w1920, element=w1918) -> (queue out=w1919:refnum<queue>)  [unwired: 2 in, 2 out]
                    }
                  }
                }
                n644 = Select(t=State_Type_Definitions."True Stop" ("Enum"), s=w1899, f=State_Type_Definitions."Task 9B: Rotate to Angle" ("Enum")) -> (s? t:f=w1902:T16)
                n645 = Select(t=w1902, s=w1900, f=State_Type_Definitions."Task 9A: Raise Arm" ("Enum")) -> (s? t:f=w1908:T16)
              }
              frame "Exit" {
                n646 = for {
                  shift-right: [w1926] -> w1923
                  shift-left: _ -> [w1927]
                  tunnel: string[] ["STOP", "RESET ENCODERS", "RESET YAW", ""] -> [w1925] mode=indexing
                  n647 = Enqueue Element(queue=w1927, element=w1925) -> (queue out=w1926:refnum<queue>)  [unwired: 2 in, 2 out]
                }
              }
            }
          }
          frame 39 {
            # ">>> Motor control cluster >>>"
            # ">>> yStepper command>>>"
            n648 = Dequeue Element(queue=w1941, timeout in ms (-1)=w1940, error in (no error)=w1939) -> (element=w1943:T8)  [unwired: 3 out]
            n649 = In Range and Coerce(upper limit=65.0, x=w1933, lower limit=55.0) -> (In Range?=w1930:bool)  [unwired: 1 out]
            n650 = case shown="\"Start Task 1\", Default" w1943 {
              tunnel: w1934 -> [w1946 _]
              tunnel: [w1954 State_Type_Definitions."True Stop" ("Enum")] -> w1936
              tunnel: w1942 -> [w1952 w1970]
              tunnel: [w1951 w1969] -> w1935
              tunnel: [State_Type_Definitions."Idle" ("Enum") State_Type_Definitions."Shutdown" ("Enum")] -> w1937
              tunnel: w1930 -> [w1944 _]
              frame "Start Task 1", Default {
                n651 = Or(x=w1944, y=w1946) -> (x .or. y?=w1945:bool)
                n652 = case shown="True" w1944 {
                  tunnel: w1952 -> [w1957 w1963]
                  tunnel: [w1956 w1961] -> w1951
                  frame False {
                    n653 = for {
                      shift-right: [w1959] -> w1956
                      shift-left: w1957 -> [w1960]
                      tunnel: string[] ["READ NAVX", "R-CW", "READ ULTRASONIC"] ("element") -> [w1958] mode=indexing
                      n654 = Enqueue Element(queue=w1960, element=w1958) -> (queue out=w1959:refnum<queue>)  [unwired: 2 in, 2 out]
                    }
                  }
                  frame True {
                    n655 = for {
                      shift-right: [w1965] -> w1961
                      shift-left: w1963 -> [w1966]
                      tunnel: string[] ["STOP", "RESET ENCODERS", "RESET YAW", "ARDUINO - ULTRASONIC", ""] -> [w1964] mode=indexing
                      n656 = Enqueue Element(queue=w1966, element=w1964) -> (queue out=w1965:refnum<queue>)  [unwired: 2 in, 2 out]
                    }
                  }
                }
                n657 = Select(t=State_Type_Definitions."True Stop" ("Enum"), s=w1946, f=State_Type_Definitions."Task 9C: Detect Box") -> (s? t:f=w1948:T16)
                n658 = Select(t=w1948, s=w1945, f=State_Type_Definitions."Task 9B: Rotate to Angle" ("Enum")) -> (s? t:f=w1954:T16)
              }
              frame "Exit" {
                n659 = for {
                  shift-right: [w1973] -> w1969
                  shift-left: w1970 -> [w1974]
                  tunnel: string[] ["STOP", "RESET ENCODERS", "RESET YAW", ""] -> [w1972] mode=indexing
                  n660 = Enqueue Element(queue=w1974, element=w1972) -> (queue out=w1973:refnum<queue>)  [unwired: 2 in, 2 out]
                }
              }
            }
          }
          frame 40 {
            # ">>> Motor control cluster >>>"
            # ">>Line Detected>>"
            # ">>Action Queue>>"
            # ">>> yStepper command>>>"
            n661 = Dequeue Element(queue=w1986, timeout in ms (-1)=w1985, error in (no error)=w1984) -> (element=w1987:T8)  [unwired: 3 out]
            n662 = case shown="\"Start Task 1\", Default" w1987 {
              tunnel: w1982 -> [w1988 _]
              tunnel: [w1998 State_Type_Definitions."True Stop" ("Enum")] -> w1979
              tunnel: w1983 -> [w1996 w2014]
              tunnel: [w1995 w2013] -> w1978
              tunnel: [State_Type_Definitions."Idle" ("Enum") State_Type_Definitions."Shutdown" ("Enum")] -> w1981
              tunnel: w1976 -> [w1989 _]
              frame "Start Task 1", Default {
                n663 = Or(x=w1988, y=w1989) -> (x .or. y?=w1990:bool)
                n664 = case shown="True" w1989 {
                  tunnel: w1996 -> [w2001 w2007]
                  tunnel: [w2000 w2005] -> w1995
                  frame False {
                    n665 = for {
                      shift-right: [w2003] -> w2000
                      shift-left: w2001 -> [w2004]
                      tunnel: string[] ["READ IR", "READ LINE SENSOR", "FORWARD - IR ASSIST"] ("element") -> [w2002] mode=indexing
                      n666 = Enqueue Element(queue=w2004, element=w2002) -> (queue out=w2003:refnum<queue>)  [unwired: 2 in, 2 out]
                    }
                  }
                  frame True {
                    n667 = for {
                      shift-right: [w2009] -> w2005
                      shift-left: w2007 -> [w2010]
                      tunnel: string[] ["STOP", "RESET ENCODERS", "RESET YAW", ""] -> [w2008] mode=indexing
                      n668 = Enqueue Element(queue=w2010, element=w2008) -> (queue out=w2009:refnum<queue>)  [unwired: 2 in, 2 out]
                    }
                  }
                }
                n669 = Select(t=State_Type_Definitions."True Stop" ("Enum"), s=w1988, f=State_Type_Definitions."Task 9D: MOVE FORWARD") -> (s? t:f=w1992:T16)
                n670 = Select(t=w1992, s=w1990, f=State_Type_Definitions."Task 9C: Detect Box" ("Enum")) -> (s? t:f=w1998:T16)
              }
              frame "Exit" {
                n671 = for {
                  shift-right: [w2017] -> w2013
                  shift-left: w2014 -> [w2018]
                  tunnel: string[] ["STOP", "RESET ENCODERS", "RESET YAW", ""] -> [w2016] mode=indexing
                  n672 = Enqueue Element(queue=w2018, element=w2016) -> (queue out=w2017:refnum<queue>)  [unwired: 2 in, 2 out]
                }
              }
            }
          }
          frame 41 {
            w2022 = u8 35 ("y")
            # ">> Wall detected >>"
            # ">> Manual override >>"
            # ">>Table Detected>>"
            # ">>> Motor control cluster >>>"
            # ">>Table or wall detectected>>"
            # ">>Action Queue>>"
            # ">>> yStepper command>>>"
            n673 = Less?(x=w2026, y=w2022) -> (x < y?=w2024:bool)
            n674 = Less?(x=w2025, y=w2022) -> (x < y?=w2023:bool)
            n675 = Less Or Equal?(x=w2028, y=15.0) -> (x <= y?=w2019:bool)
            n676 = And(x=w2024, y=w2023) -> (x .and. y?=w2021:bool)
            "Front Wall detected" <- w2021
            n677 = Dequeue Element(queue=w2039, timeout in ms (-1)=w2038, error in (no error)=w2037) -> (element=w2040:T8)  [unwired: 3 out]
            n678 = Or(x=w2019, y=w2021) -> (x .or. y?=w2020:bool)
            n679 = case shown="\"Start Task 1\", Default" w2040 {
              tunnel: w2035 -> [w2041 _]
              tunnel: [w2051 State_Type_Definitions."True Stop" ("Enum")] -> w2032
              tunnel: w2036 -> [w2049 w2067]
              tunnel: [w2048 w2066] -> w2031
              tunnel: [State_Type_Definitions."Idle" ("Enum") State_Type_Definitions."Shutdown" ("Enum")] -> w2034
              tunnel: w2020 -> [w2042 _]
              frame "Start Task 1", Default {
                n680 = Or(x=w2041, y=w2042) -> (x .or. y?=w2043:bool)
                n681 = case shown="False" w2042 {
                  tunnel: w2049 -> [w2054 w2060]
                  tunnel: [w2053 w2058] -> w2048
                  frame False {
                    n682 = for {
                      shift-right: [w2056] -> w2053
                      shift-left: w2054 -> [w2057]
                      tunnel: string[] ["READ IR", "FORWARD - IR ASSIST", "READ ULTRASONIC"] ("element") -> [w2055] mode=indexing
                      n683 = Enqueue Element(queue=w2057, element=w2055) -> (queue out=w2056:refnum<queue>)  [unwired: 2 in, 2 out]
                    }
                  }
                  frame True {
                    n684 = for {
                      shift-right: [w2062] -> w2058
                      shift-left: w2060 -> [w2063]
                      tunnel: string[] ["STOP", "RESET ENCODERS", "RESET YAW", ""] -> [w2061] mode=indexing
                      n685 = Enqueue Element(queue=w2063, element=w2061) -> (queue out=w2062:refnum<queue>)  [unwired: 2 in, 2 out]
                    }
                  }
                }
                n686 = Select(t=State_Type_Definitions."True Stop" ("Enum"), s=w2041, f=State_Type_Definitions."True Stop") -> (s? t:f=w2045:T16)
                n687 = Select(t=w2045, s=w2043, f=State_Type_Definitions."Task 9D: MOVE FORWARD" ("Enum")) -> (s? t:f=w2051:T16)
              }
              frame "Exit" {
                n688 = for {
                  shift-right: [w2070] -> w2066
                  shift-left: w2067 -> [w2071]
                  tunnel: string[] ["STOP", "RESET ENCODERS", "RESET YAW", ""] -> [w2069] mode=indexing
                  n689 = Enqueue Element(queue=w2071, element=w2069) -> (queue out=w2070:refnum<queue>)  [unwired: 2 in, 2 out]
                }
              }
            }
          }
          frame 42 {
            # ">> Item Selection Bias >>"
            # ">> Line detected? >>"
            # ">> Manual override >>"
            # ">>> Motor control cluster >>>"
            # ">>Action Queue>>"
            # ">>> yStepper command>>>"
            n690 = Dequeue Element(queue=w2083, timeout in ms (-1)=w2082, error in (no error)=w2081) -> (element=w2084:T8)  [unwired: 3 out]
            n691 = case shown="\"Start Task 1\", Default" w2084 {
              tunnel: w2079 -> [w2085 _]
              tunnel: [w2095 State_Type_Definitions."True Stop" ("Enum")] -> w2076
              tunnel: w2080 -> [w2093 w2111]
              tunnel: [w2092 w2110] -> w2075
              tunnel: [State_Type_Definitions."Idle" ("Enum") State_Type_Definitions."Shutdown" ("Enum")] -> w2078
              tunnel: w2072 -> [w2086 _]
              frame "Start Task 1", Default {
                n692 = Or(x=w2085, y=w2086) -> (x .or. y?=w2087:bool)
                n693 = case shown="False" w2086 {
                  tunnel: w2093 -> [w2098 w2104]
                  tunnel: [w2097 w2102] -> w2092
                  frame False {
                    n694 = for {
                      shift-right: [w2100] -> w2097
                      shift-left: w2098 -> [w2101]
                      tunnel: string[] ["LEFT", "READ NAVX", "READ LINE SENSOR", ""] ("element") -> [w2099] mode=indexing
                      n695 = Enqueue Element(queue=w2101, element=w2099) -> (queue out=w2100:refnum<queue>)  [unwired: 2 in, 2 out]
                    }
                  }
                  frame True {
                    n696 = for {
                      shift-right: [w2106] -> w2102
                      shift-left: w2104 -> [w2107]
                      tunnel: string[] ["STOP", "RESET ENCODERS", "RESET YAW", "RESET FLAGS", "OPEN LIFE CAM", "SET TIMER 2"] -> [w2105] mode=indexing
                      n697 = Enqueue Element(queue=w2107, element=w2105) -> (queue out=w2106:refnum<queue>)  [unwired: 2 in, 2 out]
                    }
                  }
                }
                n698 = Select(t=State_Type_Definitions."True Stop" ("Enum"), s=w2085, f=State_Type_Definitions."Task 9F: SCAN IMAGE") -> (s? t:f=w2089:T16)
                n699 = Select(t=w2089, s=w2087, f=State_Type_Definitions."Task 9E: MOVE LEFT" ("Enum")) -> (s? t:f=w2095:T16)
              }
              frame "Exit" {
                n700 = for {
                  shift-right: [w2114] -> w2110
                  shift-left: w2111 -> [w2115]
                  tunnel: string[] ["STOP", "RESET ENCODERS", "RESET YAW", ""] -> [w2113] mode=indexing
                  n701 = Enqueue Element(queue=w2115, element=w2113) -> (queue out=w2114:refnum<queue>)  [unwired: 2 in, 2 out]
                }
              }
            }
          }
          frame 43 {
            # ">>> Motor control cluster >>>"
            # ">>Time up? >>"
            # ">>> yStepper command>>>"
            # ">> Manual override >>"
            n702 = Dequeue Element(queue=w2127, timeout in ms (-1)=w2123, error in (no error)=w2126) -> (element=w2128:T8)  [unwired: 3 out]
            n703 = case shown="\"Start Task 1\", Default" w2128 {
              tunnel: [w2139 State_Type_Definitions."True Stop" ("Enum")] -> w2121
              tunnel: [w2137 w2155] -> w2120
              tunnel: w2124 -> [w2136 w2152]
              tunnel: w2125 -> [w2130 _]
              tunnel: [State_Type_Definitions."Idle" ("Enum") State_Type_Definitions."Shutdown" ("Enum")] -> w2122
              tunnel: w2116 -> [w2129 _]
              frame "Start Task 1", Default {
                # ">> WIill proceed to part ii if not manual override >>"
                # ">>If ENABLE or Trigger is set to true>>"
                n704 = Or(x=w2129, y=w2130) -> (x .or. y?=w2131:bool)
                n705 = case shown="True" w2129 {
                  tunnel: [w2142 w2148] -> w2137
                  tunnel: w2136 -> [w2141 w2147]
                  frame False {
                    n706 = for {
                      shift-right: [w2144] -> w2142
                      shift-left: w2141 -> [w2145]
                      tunnel: string[] ["CAM ACQ", "START TIMER"] ("element") -> [w2143] mode=indexing
                      n707 = Enqueue Element(queue=w2145, element=w2143) -> (queue out=w2144:refnum<queue>)  [unwired: 2 in, 2 out]
                    }
                  }
                  frame True {
                    n708 = for {
                      shift-right: [w2150] -> w2148
                      shift-left: w2147 -> [w2151]
                      tunnel: string[] ["CLOSE CAM", "SET TIMER 5", "", "", "", ""] -> [w2149] mode=indexing
                      n709 = Enqueue Element(queue=w2151, element=w2149) -> (queue out=w2150:refnum<queue>)  [unwired: 2 in, 2 out]
                    }
                  }
                }
                n710 = Select(t=State_Type_Definitions."True Stop" ("Enum"), s=w2130, f=State_Type_Definitions."Task 9G: PROCESS COLOUR" ("Enum")) -> (s? t:f=w2133:T16)
                n711 = Select(t=w2133, s=w2131, f=State_Type_Definitions."Task 9F: SCAN IMAGE" ("Enum")) -> (s? t:f=w2139:T16)
              }
              frame "Exit" {
                n712 = for {
                  shift-right: [w2158] -> w2155
                  shift-left: w2152 -> [w2159]
                  tunnel: string[] ["STOP", "RESET ENCODERS", "RESET YAW", ""] -> [w2157] mode=indexing
                  n713 = Enqueue Element(queue=w2159, element=w2157) -> (queue out=w2158:refnum<queue>)  [unwired: 2 in, 2 out]
                }
              }
            }
          }
          frame 44 {
            # ">>> Motor control cluster >>>"
            # ">>> yStepper command>>>"
            # ">>Object detected>>"
            n714 = Less Or Equal?(x=w2163, y=30.0) -> (x <= y?=w2161:bool)
            "Table obstruct" <- w2161
            n715 = Dequeue Element(queue=w2169, timeout in ms (-1)=w2168, error in (no error)=w2167) -> (element=w2174:T8)  [unwired: 3 out]
            n716 = case shown="\"Start Task 1\", Default" w2174 {
              tunnel: w2161 -> [w2177 _]
              tunnel: [w2184 State_Type_Definitions."True Stop" ("Enum")] -> w2173
              tunnel: w2166 -> [w2176 _]
              tunnel: w2170 -> [w2183 w2200]
              tunnel: [w2182 w2201] -> w2172
              tunnel: [State_Type_Definitions."Idle" ("Enum") State_Type_Definitions."Shutdown" ("Enum")] -> w2171
              frame "Start Task 1", Default {
                n717 = case shown="True" w2177 {
                  tunnel: w2183 -> [w2187 w2194]
                  tunnel: [w2188 w2193] -> w2182
                  frame False {
                    n718 = for {
                      tunnel: string[] ["START TIMER", "COLOUR PROCESSING", ""] ("element") -> [w2189] mode=indexing
                      shift-right: [w2191] -> w2188
                      shift-left: w2187 -> [w2190]
                      n719 = Enqueue Element(queue=w2190, element=w2189) -> (queue out=w2191:refnum<queue>)  [unwired: 2 in, 2 out]
                    }
                  }
                  frame True {
                    n720 = for {
                      shift-right: [w2196] -> w2193
                      shift-left: w2194 -> [w2197]
                      tunnel: string[] ["DISPOSE BUFFERS", "CLOSE CAM", "RESET ENCODERS", "RESET YAW", "RESET FLAGS"] -> [w2195] mode=indexing
                      n721 = Enqueue Element(queue=w2197, element=w2195) -> (queue out=w2196:refnum<queue>)  [unwired: 2 in, 2 out]
                    }
                  }
                }
                n722 = Or(x=w2177, y=w2176) -> (x .or. y?=w2175:bool)
                n723 = Select(t=State_Type_Definitions."True Stop" ("Enum"), s=w2176, f=State_Type_Definitions."Task 9H: MOVE RIGHT" ("Enum")) -> (s? t:f=w2178:T16)
                n724 = Select(t=w2178, s=w2175, f=State_Type_Definitions."Task 9G: PROCESS COLOUR" ("Enum")) -> (s? t:f=w2184:T16)
              }
              frame "Exit" {
                n725 = for {
                  shift-right: [w2204] -> w2201
                  shift-left: w2200 -> [w2205]
                  tunnel: string[] ["STOP", "RESET ENCODERS", "RESET YAW", "ARDUINO MODE 0"] -> [w2203] mode=indexing
                  n726 = Enqueue Element(queue=w2205, element=w2203) -> (queue out=w2204:refnum<queue>)  [unwired: 2 in, 2 out]
                }
              }
            }
          }
          frame 45 {
            # ">> Item Selection Bias >>"
            # ">>> Motor control cluster >>>"
            # ">>> yStepper command>>>"
            n727 = Dequeue Element(queue=w2215, timeout in ms (-1)=w2216, error in (no error)=w2217) -> (element=w2219:T8)  [unwired: 3 out]
            n728 = Greater?(x=w2207, y=50.0) -> (0:w2208:bool)
            n729 = And(x=w2209, y=w2208) -> (x .and. y?=w2210:bool)
            n730 = case shown="\"Start Task 1\", Default" w2219 {
              tunnel: w2210 -> [w2225 _]
              tunnel: [w2232 State_Type_Definitions."True Stop" ("Enum")] -> w2212
              tunnel: w2218 -> [w2224 _]
              tunnel: w2214 -> [w2231 w2248]
              tunnel: [w2230 w2249] -> w2213
              tunnel: [State_Type_Definitions."Idle" ("Enum") State_Type_Definitions."Shutdown" ("Enum")] -> w2211
              frame "Start Task 1", Default {
                n731 = case shown="False" w2225 {
                  tunnel: w2231 -> [w2235 w2242]
                  tunnel: [w2236 w2241] -> w2230
                  frame False {
                    n732 = for {
                      tunnel: string[] ["READ LINE SENSOR", "READ NAVX", "RIGHT", "READ ENCODERS"] ("element") -> [w2237] mode=indexing
                      shift-right: [w2239] -> w2236
                      shift-left: w2235 -> [w2238]
                      n733 = Enqueue Element(queue=w2238, element=w2237) -> (queue out=w2239:refnum<queue>)  [unwired: 2 in, 2 out]
                    }
                  }
                  frame True {
                    n734 = for {
                      shift-right: [w2244] -> w2241
                      shift-left: w2242 -> [w2245]
                      tunnel: string[] ["STOP", "RESET ENCODERS", "RESET YAW", "OPEN LIFE CAM", "SET TIMER 2", "RESET FLAGS"] -> [w2243] mode=indexing
                      n735 = Enqueue Element(queue=w2245, element=w2243) -> (queue out=w2244:refnum<queue>)  [unwired: 2 in, 2 out]
                    }
                  }
                }
                n736 = Or(x=w2225, y=w2224) -> (x .or. y?=w2223:bool)
                n737 = Select(t=State_Type_Definitions."True Stop" ("Enum"), s=w2224, f=State_Type_Definitions."Task 9I: SCAN IMAGE" ("Enum")) -> (s? t:f=w2226:T16)
                n738 = Select(t=w2226, s=w2223, f=State_Type_Definitions."Task 9H: MOVE RIGHT" ("Enum")) -> (s? t:f=w2232:T16)
              }
              frame "Exit" {
                n739 = for {
                  shift-right: [w2252] -> w2249
                  shift-left: w2248 -> [w2253]
                  tunnel: string[] ["STOP", "RESET ENCODERS", "RESET YAW", "ARDUINO MODE 0"] -> [w2251] mode=indexing
                  n740 = Enqueue Element(queue=w2253, element=w2251) -> (queue out=w2252:refnum<queue>)  [unwired: 2 in, 2 out]
                }
              }
            }
          }
          frame 46 {
            # ">> Item Selection Bias >>"
            n741 = Dequeue Element(queue=w2255, timeout in ms (-1)=w2256, error in (no error)=w2257) -> (element=w2263:T8)  [unwired: 3 out]
            n742 = case shown="\"Start Task 1\", Default" w2263 {
              tunnel: w2254 -> [w2269 _]
              tunnel: [w2276 State_Type_Definitions."True Stop" ("Enum")] -> w2260
              tunnel: w2258 -> [w2268 _]
              tunnel: w2262 -> [w2275 w2292]
              tunnel: [w2274 w2293] -> w2261
              tunnel: [State_Type_Definitions."Idle" ("Enum") State_Type_Definitions."Shutdown" ("Enum")] -> w2259
              frame "Start Task 1", Default {
                n743 = case shown="True" w2269 {
                  tunnel: w2275 -> [w2279 w2286]
                  tunnel: [w2280 w2285] -> w2274
                  frame False {
                    n744 = for {
                      tunnel: string[] ["START TIMER", "CAM ACQ", ""] ("element") -> [w2281] mode=indexing
                      shift-right: [w2283] -> w2280
                      shift-left: w2279 -> [w2282]
                      n745 = Enqueue Element(queue=w2282, element=w2281) -> (queue out=w2283:refnum<queue>)  [unwired: 2 in, 2 out]
                    }
                  }
                  frame True {
                    n746 = for {
                      shift-right: [w2288] -> w2285
                      shift-left: w2286 -> [w2289]
                      tunnel: string[] ["CLOSE CAM", "SET TIMER 5", "", "", "", ""] -> [w2287] mode=indexing
                      n747 = Enqueue Element(queue=w2289, element=w2287) -> (queue out=w2288:refnum<queue>)  [unwired: 2 in, 2 out]
                    }
                  }
                }
                n748 = Or(x=w2269, y=w2268) -> (x .or. y?=w2267:bool)
                n749 = Select(t=State_Type_Definitions."True Stop" ("Enum"), s=w2268, f=State_Type_Definitions."Task 9J: PROCESS COLOUR" ("Enum")) -> (s? t:f=w2270:T16)
                n750 = Select(t=w2270, s=w2267, f=State_Type_Definitions."Task 9I: SCAN IMAGE" ("Enum")) -> (s? t:f=w2276:T16)
              }
              frame "Exit" {
                n751 = for {
                  shift-right: [w2296] -> w2293
                  shift-left: w2292 -> [w2297]
                  tunnel: string[] ["STOP", "RESET ENCODERS", "RESET YAW", "ARDUINO MODE 0"] -> [w2295] mode=indexing
                  n752 = Enqueue Element(queue=w2297, element=w2295) -> (queue out=w2296:refnum<queue>)  [unwired: 2 in, 2 out]
                }
              }
            }
          }
          frame 47 {
            # ">> Item Selection Bias >>"
            n753 = Dequeue Element(queue=w2303, timeout in ms (-1)=w2304, error in (no error)=w2305) -> (element=w2307:T8)  [unwired: 3 out]
            n754 = case shown="\"Start Task 1\", Default" w2307 {
              tunnel: w2298 -> [w2313 _]
              tunnel: [w2320 State_Type_Definitions."True Stop" ("Enum")] -> w2301
              tunnel: w2306 -> [w2312 _]
              tunnel: w2302 -> [w2319 w2336]
              tunnel: [w2318 w2337] -> w2300
              tunnel: [State_Type_Definitions."Idle" ("Enum") State_Type_Definitions."Shutdown" ("Enum")] -> w2299
              frame "Start Task 1", Default {
                n755 = case shown="True" w2313 {
                  tunnel: w2319 -> [w2323 w2330]
                  tunnel: [w2324 w2329] -> w2318
                  frame False {
                    n756 = for {
                      tunnel: string[] ["START TIMER", "COLOUR PROCESSING", ""] ("element") -> [w2325] mode=indexing
                      shift-right: [w2327] -> w2324
                      shift-left: w2323 -> [w2326]
                      n757 = Enqueue Element(queue=w2326, element=w2325) -> (queue out=w2327:refnum<queue>)  [unwired: 2 in, 2 out]
                    }
                  }
                  frame True {
                    n758 = for {
                      shift-right: [w2332] -> w2329
                      shift-left: w2330 -> [w2333]
                      tunnel: string[] ["CLOSE CAM", "DISPOSE BUFFERS", "RESET ENCODERS", "RESET YAW", "RESET FLAGS", ""] -> [w2331] mode=indexing
                      n759 = Enqueue Element(queue=w2333, element=w2331) -> (queue out=w2332:refnum<queue>)  [unwired: 2 in, 2 out]
                    }
                  }
                }
                n760 = Or(x=w2313, y=w2312) -> (x .or. y?=w2311:bool)
                n761 = Select(t=State_Type_Definitions."True Stop" ("Enum"), s=w2312, f=State_Type_Definitions."Task 9K: ROTATE 90 CW" ("Enum")) -> (s? t:f=w2314:T16)
                n762 = Select(t=w2314, s=w2311, f=State_Type_Definitions."Task 9J: PROCESS COLOUR" ("Enum")) -> (s? t:f=w2320:T16)
              }
              frame "Exit" {
                n763 = for {
                  shift-right: [w2340] -> w2337
                  shift-left: w2336 -> [w2341]
                  tunnel: string[] ["STOP", "RESET ENCODERS", "RESET YAW", "ARDUINO MODE 0"] -> [w2339] mode=indexing
                  n764 = Enqueue Element(queue=w2341, element=w2339) -> (queue out=w2340:refnum<queue>)  [unwired: 2 in, 2 out]
                }
              }
            }
          }
          frame 48 {
            # ">>> Motor control cluster >>>"
            # ">>> yStepper command>>>"
            # ">> Item Selection Bias >>"
            n765 = Less?(x=w2345, y=-38.0) -> (x < y?=w2343:bool)
            n766 = Dequeue Element(queue=w2351, timeout in ms (-1)=w2350, error in (no error)=w2349) -> (element=w2353:T8)  [unwired: 3 out]
            n767 = case shown="\"Start Task 1\", Default" w2353 {
              tunnel: w2343 -> [w2359 _]
              tunnel: [w2366 State_Type_Definitions."True Stop" ("Enum")] -> w2347
              tunnel: w2348 -> [w2358 _]
              tunnel: w2352 -> [w2365 w2382]
              tunnel: [w2364 w2383] -> w2342
              tunnel: [State_Type_Definitions."Idle" ("Enum") State_Type_Definitions."Shutdown" ("Enum")] -> w2346
              frame "Start Task 1", Default {
                n768 = case shown="True" w2359 {
                  tunnel: w2365 -> [w2369 w2376]
                  tunnel: [w2370 w2375] -> w2364
                  frame False {
                    n769 = for {
                      tunnel: string[] ["READ ENCODERS", "R-CW"] ("element") -> [w2371] mode=indexing
                      shift-right: [w2373] -> w2370
                      shift-left: w2369 -> [w2372]
                      n770 = Enqueue Element(queue=w2372, element=w2371) -> (queue out=w2373:refnum<queue>)  [unwired: 2 in, 2 out]
                    }
                  }
                  frame True {
                    n771 = for {
                      shift-right: [w2378] -> w2375
                      shift-left: w2376 -> [w2379]
                      tunnel: string[] ["STOP", "RESET ENCODERS", "RESET FLAGS", "RESET YAW", "READ IR", "ARDUINO - ULTRASONIC"] -> [w2377] mode=indexing
                      n772 = Enqueue Element(queue=w2379, element=w2377) -> (queue out=w2378:refnum<queue>)  [unwired: 2 in, 2 out]
                    }
                  }
                }
                n773 = Or(x=w2359, y=w2358) -> (x .or. y?=w2357:bool)
                n774 = Select(t=State_Type_Definitions."True Stop" ("Enum"), s=w2358, f=State_Type_Definitions."Task 9L: MOVE FORWARD" ("Enum")) -> (s? t:f=w2360:T16)
                n775 = Select(t=w2360, s=w2357, f=State_Type_Definitions."Task 9K: ROTATE 90 CW" ("Enum")) -> (s? t:f=w2366:T16)
              }
              frame "Exit" {
                n776 = for {
                  shift-right: [w2386] -> w2383
                  shift-left: w2382 -> [w2387]
                  tunnel: string[] ["STOP", "RESET ENCODERS", "RESET YAW", "ARDUINO MODE 0"] -> [w2385] mode=indexing
                  n777 = Enqueue Element(queue=w2387, element=w2385) -> (queue out=w2386:refnum<queue>)  [unwired: 2 in, 2 out]
                }
              }
            }
          }
          frame 49 {
            w2400 = u8 50 ("y")
            # ">>> Motor control cluster >>>"
            # ">>> yStepper command>>>"
            # ">> Item Selection Bias >>"
            n778 = Less?(x=w2402, y=w2400) -> (x < y?=w2395:bool)
            n779 = Dequeue Element(queue=w2406, timeout in ms (-1)=w2405, error in (no error)=w2404) -> (element=w2410:T8)  [unwired: 3 out]
            n780 = Less?(x=w2401, y=w2400) -> (x < y?=w2396:bool)
            n781 = And(x=w2396, y=w2395) -> (x .and. y?=w2388:bool)
            n782 = Less Or Equal?(x=w2399, y=15.0) -> (x <= y?=w2394:bool)
            n783 = Greater?(x=w2393, y=100.0) -> (0:w2392:bool)
            n784 = Or(x=w2394, y=w2388) -> (x .or. y?=w2390:bool)
            n785 = And(x=w2392, y=w2390) -> (x .and. y?=w2391:bool)
            "Stop?" <- w2391
            n786 = case shown="\"Start Task 1\", Default" w2410 {
              tunnel: w2391 -> [w2416 _]
              tunnel: [w2423 State_Type_Definitions."True Stop" ("Enum")] -> w2408
              tunnel: w2403 -> [w2415 _]
              tunnel: w2407 -> [w2422 w2439]
              tunnel: [w2421 w2440] -> w2397
              tunnel: [State_Type_Definitions."Idle" ("Enum") State_Type_Definitions."Shutdown" ("Enum")] -> w2409
              frame "Start Task 1", Default {
                n787 = case shown="True" w2416 {
                  tunnel: w2422 -> [w2426 w2433]
                  tunnel: [w2427 w2432] -> w2421
                  frame False {
                    n788 = for {
                      tunnel: string[] ["READ IR", "FORWARD", "READ NAVX", "READ ENCODERS"] ("element") -> [w2428] mode=indexing
                      shift-right: [w2430] -> w2427
                      shift-left: w2426 -> [w2429]
                      n789 = Enqueue Element(queue=w2429, element=w2428) -> (queue out=w2430:refnum<queue>)  [unwired: 2 in, 2 out]
                    }
                  }
                  frame True {
                    n790 = for {
                      shift-right: [w2435] -> w2432
                      shift-left: w2433 -> [w2436]
                      tunnel: string[] ["STOP", "RESET ENCODERS", "RESET FLAGS", "RESET YAW", "", ""] -> [w2434] mode=indexing
                      n791 = Enqueue Element(queue=w2436, element=w2434) -> (queue out=w2435:refnum<queue>)  [unwired: 2 in, 2 out]
                    }
                  }
                }
                n792 = Or(x=w2416, y=w2415) -> (x .or. y?=w2414:bool)
                n793 = Select(t=State_Type_Definitions."True Stop" ("Enum"), s=w2415, f=State_Type_Definitions."True Stop" ("Enum")) -> (s? t:f=w2417:T16)
                n794 = Select(t=w2417, s=w2414, f=State_Type_Definitions."Task 9L: MOVE FORWARD" ("Enum")) -> (s? t:f=w2423:T16)
              }
              frame "Exit" {
                n795 = for {
                  shift-right: [w2443] -> w2440
                  shift-left: w2439 -> [w2444]
                  tunnel: string[] ["STOP", "RESET ENCODERS", "RESET YAW", "ARDUINO MODE 0"] -> [w2442] mode=indexing
                  n796 = Enqueue Element(queue=w2444, element=w2442) -> (queue out=w2443:refnum<queue>)  [unwired: 2 in, 2 out]
                }
              }
            }
          }
          frame 50 {
            # ">> Item Selection Bias >>"
            n797 = Dequeue Element(queue=w2449, timeout in ms (-1)=w2448, error in (no error)=w2447) -> (element=w2454:T8)  [unwired: 3 out]
            n798 = case shown="\"Start Task 1\", Default" w2454 {
              tunnel: w2445 -> [w2460 _]
              tunnel: [w2467 State_Type_Definitions."True Stop" ("Enum")] -> w2452
              tunnel: w2446 -> [w2459 _]
              tunnel: w2450 -> [w2466 w2483]
              tunnel: [w2465 w2484] -> w2451
              tunnel: [State_Type_Definitions."Idle" ("Enum") State_Type_Definitions."Shutdown" ("Enum")] -> w2453
              frame "Start Task 1", Default {
                n799 = case shown="False" w2460 {
                  tunnel: w2466 -> [w2470 w2477]
                  tunnel: [w2471 w2476] -> w2465
                  frame False {
                    n800 = for {
                      tunnel: string[] ["READ LINE SENSOR", "READ NAVX", "RIGHT", "READ ENCODERS"] ("element") -> [w2472] mode=indexing
                      shift-right: [w2474] -> w2471
                      shift-left: w2470 -> [w2473]
                      n801 = Enqueue Element(queue=w2473, element=w2472) -> (queue out=w2474:refnum<queue>)  [unwired: 2 in, 2 out]
                    }
                  }
                  frame True {
                    n802 = for {
                      shift-right: [w2479] -> w2476
                      shift-left: w2477 -> [w2480]
                      tunnel: string[] ["STOP", "RESET ENCODERS", "RESET YAW", "OPEN LIFE CAM", "SET TIMER 2", "RESET FLAGS"] -> [w2478] mode=indexing
                      n803 = Enqueue Element(queue=w2480, element=w2478) -> (queue out=w2479:refnum<queue>)  [unwired: 2 in, 2 out]
                    }
                  }
                }
                n804 = Or(x=w2460, y=w2459) -> (x .or. y?=w2458:bool)
                n805 = Select(t=State_Type_Definitions."True Stop" ("Enum"), s=w2459, f=State_Type_Definitions."Task 9N: SCAN IMAGE" ("Enum")) -> (s? t:f=w2461:T16)
                n806 = Select(t=w2461, s=w2458, f=State_Type_Definitions."Task 9M: MOVE RIGHT" ("Enum")) -> (s? t:f=w2467:T16)
              }
              frame "Exit" {
                n807 = for {
                  shift-right: [w2487] -> w2484
                  shift-left: w2483 -> [w2488]
                  tunnel: string[] ["STOP", "RESET ENCODERS", "RESET YAW", "ARDUINO MODE 0"] -> [w2486] mode=indexing
                  n808 = Enqueue Element(queue=w2488, element=w2486) -> (queue out=w2487:refnum<queue>)  [unwired: 2 in, 2 out]
                }
              }
            }
          }
          frame 51 {
            # ">> Manual override >>"
            n809 = Dequeue Element(queue=w2497, timeout in ms (-1)=w2496, error in (no error)=w2495) -> (element=w2498:T8)  [unwired: 3 out]
            n810 = case shown="\"Start Task 1\", Default" w2498 {
              tunnel: [w2512 State_Type_Definitions."True Stop" ("Enum")] -> w2490
              tunnel: [w2510 w2528] -> w2489
              tunnel: w2493 -> [w2509 w2525]
              tunnel: w2494 -> [w2503 _]
              tunnel: [State_Type_Definitions."Idle" ("Enum") State_Type_Definitions."Shutdown" ("Enum")] -> w2491
              tunnel: w2492 -> [w2502 _]
              frame "Start Task 1", Default {
                # ">> WIill proceed to part ii if not manual override >>"
                # ">>If ENABLE or Trigger is set to true>>"
                n811 = Or(x=w2502, y=w2503) -> (x .or. y?=w2504:bool)
                n812 = case shown="False" w2502 {
                  tunnel: [w2515 w2521] -> w2510
                  tunnel: w2509 -> [w2514 w2520]
                  frame False {
                    n813 = for {
                      shift-right: [w2517] -> w2515
                      shift-left: w2514 -> [w2518]
                      tunnel: string[] ["CAM ACQ", "START TIMER"] ("element") -> [w2516] mode=indexing
                      n814 = Enqueue Element(queue=w2518, element=w2516) -> (queue out=w2517:refnum<queue>)  [unwired: 2 in, 2 out]
                    }
                  }
                  frame True {
                    n815 = for {
                      shift-right: [w2523] -> w2521
                      shift-left: w2520 -> [w2524]
                      tunnel: string[] ["CLOSE CAM", "SET TIMER 5", "", "", "", ""] -> [w2522] mode=indexing
                      n816 = Enqueue Element(queue=w2524, element=w2522) -> (queue out=w2523:refnum<queue>)  [unwired: 2 in, 2 out]
                    }
                  }
                }
                n817 = Select(t=State_Type_Definitions."True Stop" ("Enum"), s=w2503, f=State_Type_Definitions."Task 9O: PROCESS COLOUR" ("Enum")) -> (s? t:f=w2506:T16)
                n818 = Select(t=w2506, s=w2504, f=State_Type_Definitions."Task 9N: SCAN IMAGE" ("Enum")) -> (s? t:f=w2512:T16)
              }
              frame "Exit" {
                n819 = for {
                  shift-right: [w2531] -> w2528
                  shift-left: w2525 -> [w2532]
                  tunnel: string[] ["STOP", "RESET ENCODERS", "RESET YAW", ""] -> [w2530] mode=indexing
                  n820 = Enqueue Element(queue=w2532, element=w2530) -> (queue out=w2531:refnum<queue>)  [unwired: 2 in, 2 out]
                }
              }
            }
          }
          frame 52 {
            # ">> Item Selection Bias >>"
            n821 = Dequeue Element(queue=w2540, timeout in ms (-1)=w2539, error in (no error)=w2538) -> (element=w2542:T8)  [unwired: 3 out]
            n822 = case shown="\"Start Task 1\", Default" w2542 {
              tunnel: w2533 -> [w2548 _]
              tunnel: [w2555 State_Type_Definitions."True Stop" ("Enum")] -> w2536
              tunnel: w2537 -> [w2547 _]
              tunnel: w2541 -> [w2554 w2571]
              tunnel: [w2553 w2572] -> w2535
              tunnel: [State_Type_Definitions."Idle" ("Enum") State_Type_Definitions."Shutdown" ("Enum")] -> w2534
              frame "Start Task 1", Default {
                n823 = case shown="False" w2548 {
                  tunnel: w2554 -> [w2558 w2565]
                  tunnel: [w2559 w2564] -> w2553
                  frame False {
                    n824 = for {
                      tunnel: string[] ["START TIMER", "COLOUR PROCESSING", ""] ("element") -> [w2560] mode=indexing
                      shift-right: [w2562] -> w2559
                      shift-left: w2558 -> [w2561]
                      n825 = Enqueue Element(queue=w2561, element=w2560) -> (queue out=w2562:refnum<queue>)  [unwired: 2 in, 2 out]
                    }
                  }
                  frame True {
                    n826 = for {
                      shift-right: [w2567] -> w2564
                      shift-left: w2565 -> [w2568]
                      tunnel: string[] ["CLOSE CAM", "DISPOSE BUFFERS", "RESET ENCODERS", "RESET YAW", "RESET FLAGS", ""] -> [w2566] mode=indexing
                      n827 = Enqueue Element(queue=w2568, element=w2566) -> (queue out=w2567:refnum<queue>)  [unwired: 2 in, 2 out]
                    }
                  }
                }
                n828 = Or(x=w2548, y=w2547) -> (x .or. y?=w2546:bool)
                n829 = Select(t=State_Type_Definitions."True Stop" ("Enum"), s=w2547, f=State_Type_Definitions."Task 9P: MOVE RIGHT" ("Enum")) -> (s? t:f=w2549:T16)
                n830 = Select(t=w2549, s=w2546, f=State_Type_Definitions."Task 9O: PROCESS COLOUR" ("Enum")) -> (s? t:f=w2555:T16)
              }
              frame "Exit" {
                n831 = for {
                  shift-right: [w2575] -> w2572
                  shift-left: w2571 -> [w2576]
                  tunnel: string[] ["STOP", "RESET ENCODERS", "RESET YAW", "ARDUINO MODE 0"] -> [w2574] mode=indexing
                  n832 = Enqueue Element(queue=w2576, element=w2574) -> (queue out=w2575:refnum<queue>)  [unwired: 2 in, 2 out]
                }
              }
            }
          }
          frame 53 {
            # ">> Item Selection Bias >>"
            n833 = Dequeue Element(queue=w2582, timeout in ms (-1)=w2581, error in (no error)=w2580) -> (element=w2590:T8)  [unwired: 3 out]
            n834 = Greater?(x=w2578, y=50.0) -> (0:w2588:bool)
            n835 = And(x=w2577, y=w2588) -> (x .and. y?=w2589:bool)
            n836 = case shown="\"Start Task 1\", Default" w2590 {
              tunnel: w2589 -> [w2596 _]
              tunnel: [w2603 State_Type_Definitions."True Stop" ("Enum")] -> w2585
              tunnel: w2579 -> [w2595 _]
              tunnel: w2583 -> [w2602 w2619]
              tunnel: [w2601 w2620] -> w2584
              tunnel: [State_Type_Definitions."Idle" ("Enum") State_Type_Definitions."Shutdown" ("Enum")] -> w2586
              frame "Start Task 1", Default {
                n837 = case shown="False" w2596 {
                  tunnel: w2602 -> [w2606 w2613]
                  tunnel: [w2607 w2612] -> w2601
                  frame False {
                    n838 = for {
                      tunnel: string[] ["READ LINE SENSOR", "READ NAVX", "RIGHT", "READ ENCODERS"] ("element") -> [w2608] mode=indexing
                      shift-right: [w2610] -> w2607
                      shift-left: w2606 -> [w2609]
                      n839 = Enqueue Element(queue=w2609, element=w2608) -> (queue out=w2610:refnum<queue>)  [unwired: 2 in, 2 out]
                    }
                  }
                  frame True {
                    n840 = for {
                      shift-right: [w2615] -> w2612
                      shift-left: w2613 -> [w2616]
                      tunnel: string[] ["STOP", "RESET ENCODERS", "RESET YAW", "OPEN LIFE CAM", "SET TIMER 2", "RESET FLAGS"] -> [w2614] mode=indexing
                      n841 = Enqueue Element(queue=w2616, element=w2614) -> (queue out=w2615:refnum<queue>)  [unwired: 2 in, 2 out]
                    }
                  }
                }
                n842 = Or(x=w2596, y=w2595) -> (x .or. y?=w2594:bool)
                n843 = Select(t=State_Type_Definitions."True Stop" ("Enum"), s=w2595, f=State_Type_Definitions."Task 9Q: SCAN IMAGE" ("Enum")) -> (s? t:f=w2597:T16)
                n844 = Select(t=w2597, s=w2594, f=State_Type_Definitions."Task 9P: MOVE RIGHT" ("Enum")) -> (s? t:f=w2603:T16)
              }
              frame "Exit" {
                n845 = for {
                  shift-right: [w2623] -> w2620
                  shift-left: w2619 -> [w2624]
                  tunnel: string[] ["STOP", "RESET ENCODERS", "RESET YAW", "ARDUINO MODE 0"] -> [w2622] mode=indexing
                  n846 = Enqueue Element(queue=w2624, element=w2622) -> (queue out=w2623:refnum<queue>)  [unwired: 2 in, 2 out]
                }
              }
            }
          }
          frame 54 {
            # ">> Manual override >>"
            n847 = Dequeue Element(queue=w2633, timeout in ms (-1)=w2632, error in (no error)=w2631) -> (element=w2634:T8)  [unwired: 3 out]
            n848 = case shown="\"Start Task 1\", Default" w2634 {
              tunnel: [w2648 State_Type_Definitions."True Stop" ("Enum")] -> w2626
              tunnel: [w2646 w2664] -> w2625
              tunnel: w2629 -> [w2645 w2661]
              tunnel: w2630 -> [w2639 _]
              tunnel: [State_Type_Definitions."Idle" ("Enum") State_Type_Definitions."Shutdown" ("Enum")] -> w2627
              tunnel: w2628 -> [w2638 _]
              frame "Start Task 1", Default {
                # ">> WIill proceed to part ii if not manual override >>"
                # ">>If ENABLE or Trigger is set to true>>"
                n849 = Or(x=w2638, y=w2639) -> (x .or. y?=w2640:bool)
                n850 = case shown="False" w2638 {
                  tunnel: [w2651 w2657] -> w2646
                  tunnel: w2645 -> [w2650 w2656]
                  frame False {
                    n851 = for {
                      shift-right: [w2653] -> w2651
                      shift-left: w2650 -> [w2654]
                      tunnel: string[] ["CAM ACQ", "START TIMER"] ("element") -> [w2652] mode=indexing
                      n852 = Enqueue Element(queue=w2654, element=w2652) -> (queue out=w2653:refnum<queue>)  [unwired: 2 in, 2 out]
                    }
                  }
                  frame True {
                    n853 = for {
                      shift-right: [w2659] -> w2657
                      shift-left: w2656 -> [w2660]
                      tunnel: string[] ["CLOSE CAM", "SET TIMER 5", "", "", "", ""] -> [w2658] mode=indexing
                      n854 = Enqueue Element(queue=w2660, element=w2658) -> (queue out=w2659:refnum<queue>)  [unwired: 2 in, 2 out]
                    }
                  }
                }
                n855 = Select(t=State_Type_Definitions."True Stop" ("Enum"), s=w2639, f=State_Type_Definitions."Task 9R: PROCESS COLOUR" ("Enum")) -> (s? t:f=w2642:T16)
                n856 = Select(t=w2642, s=w2640, f=State_Type_Definitions."Task 9Q: SCAN IMAGE" ("Enum")) -> (s? t:f=w2648:T16)
              }
              frame "Exit" {
                n857 = for {
                  shift-right: [w2667] -> w2664
                  shift-left: w2661 -> [w2668]
                  tunnel: string[] ["STOP", "RESET ENCODERS", "RESET YAW", ""] -> [w2666] mode=indexing
                  n858 = Enqueue Element(queue=w2668, element=w2666) -> (queue out=w2667:refnum<queue>)  [unwired: 2 in, 2 out]
                }
              }
            }
          }
          frame 55 {
            # ">> Item Selection Bias >>"
            # ">>> Motor control cluster >>>"
            # ">>> yStepper command>>>"
            n859 = Dequeue Element(queue=w2674, timeout in ms (-1)=w2675, error in (no error)=w2676) -> (element=w2678:T8)  [unwired: 3 out]
            n860 = case shown="\"Start Task 1\", Default" w2678 {
              tunnel: w2672 -> [w2684 _]
              tunnel: [w2691 State_Type_Definitions."True Stop" ("Enum")] -> w2670
              tunnel: w2677 -> [w2683 _]
              tunnel: w2673 -> [w2690 w2707]
              tunnel: [w2689 w2708] -> w2669
              tunnel: [State_Type_Definitions."Idle" ("Enum") State_Type_Definitions."Shutdown" ("Enum")] -> w2671
              frame "Start Task 1", Default {
                n861 = case shown="False" w2684 {
                  tunnel: w2690 -> [w2694 w2701]
                  tunnel: [w2695 w2700] -> w2689
                  frame False {
                    n862 = for {
                      tunnel: string[] ["START TIMER", "COLOUR PROCESSING", ""] ("element") -> [w2696] mode=indexing
                      shift-right: [w2698] -> w2695
                      shift-left: w2694 -> [w2697]
                      n863 = Enqueue Element(queue=w2697, element=w2696) -> (queue out=w2698:refnum<queue>)  [unwired: 2 in, 2 out]
                    }
                  }
                  frame True {
                    n864 = for {
                      shift-right: [w2703] -> w2700
                      shift-left: w2701 -> [w2704]
                      tunnel: string[] ["CLOSE CAM", "DISPOSE BUFFERS", "RESET ENCODERS", "RESET YAW", "RESET FLAGS", ""] -> [w2702] mode=indexing
                      n865 = Enqueue Element(queue=w2704, element=w2702) -> (queue out=w2703:refnum<queue>)  [unwired: 2 in, 2 out]
                    }
                  }
                }
                n866 = Or(x=w2684, y=w2683) -> (x .or. y?=w2682:bool)
                n867 = Select(t=State_Type_Definitions."True Stop" ("Enum"), s=w2683, f=State_Type_Definitions."True Stop" ("Enum")) -> (s? t:f=w2685:T16)
                n868 = Select(t=w2685, s=w2682, f=State_Type_Definitions."Task 9R: PROCESS COLOUR" ("Enum")) -> (s? t:f=w2691:T16)
              }
              frame "Exit" {
                n869 = for {
                  shift-right: [w2711] -> w2708
                  shift-left: w2707 -> [w2712]
                  tunnel: string[] ["STOP", "RESET ENCODERS", "RESET YAW", "ARDUINO MODE 0"] -> [w2710] mode=indexing
                  n870 = Enqueue Element(queue=w2712, element=w2710) -> (queue out=w2711:refnum<queue>)  [unwired: 2 in, 2 out]
                }
              }
            }
          }
        }
        "Object Detection" <- w300
        "Ultrasonic sensors" <- w323
        "Encoder values" <- w312
        "Stepper position values" <- w296
        "NAVX Values" <- w294
        "Time up" <- w292
        "IR Sensors" <- w286
        "Line sensors" <- w281
      }
    }
    "Object recognition mode" <- w212
    n871 = local write "Green LED"(w222) -> ()
  }
  n872 = while {
    stop <- w3475 stop-if-true
    n873 = call "MOTOR CONTROL WITH PID AE.vi"("AE Mode"=MOTOR_CONTROL_WITH_PID_AE_DATA_MODE_TYPE_DEF."Read from AE") -> ("Speed & distance"=→"Speed & distance":T13)  [unwired: 3 in]
    n874 = call "FGV Bool.vi"("Init/Read/Write State"=States_for_Action_Engine."Read") -> ("Output node"=w3475:bool)  [unwired: 2 in, 1 out]
    n875 = Wait (ms)(milliseconds to wait=u32 5) -> ()  [unwired: 1 out]
  }
  n876 = call <vilib>:"DIO Close.vi"("error in (no error)"=w22, "DIO Info In"=w25) -> ()  [unwired: 9 in, 1 out]
  n877 = call <vilib>:"DIO Close.vi"("error in (no error)"=w32, "DIO Info In"=w34) -> ()  [unwired: 9 in, 1 out]
  n878 = call <vilib>:"NavX Close.vi"("error in (no error)"=w9, "NavX Info In"=w8) -> ()  [unwired: 9 in, 1 out]
  n879 = call <vilib>:"DIO Close.vi"("error in (no error)"=w27, "DIO Info In"=w29) -> ()  [unwired: 9 in, 1 out]
  n880 = call <vilib>:"DIO Close.vi"("error in (no error)"=w16, "DIO Info In"=w17) -> ()  [unwired: 9 in, 1 out]
  n881 = call <vilib>:"DIO Close.vi"("error in (no error)"=w11, "DIO Info In"=w12) -> ()  [unwired: 9 in, 1 out]
  n882 = Merge Errors "Merge Errors"(w62, w61) -> (w44:errorcluster)
  n883 = Merge Errors(w48, w44) -> (w43:errorcluster)
  n884 = Destroy User Event(user event=w66, error in=w43) -> ()  [unwired: 1 out]
  n885 = Release Queue(queue=w39, error in (no error)=w43) -> (error out=→"Queue Errors":errorcluster)  [unwired: 1 in, 2 out]
  n886 = Release Queue(queue=w56, error in (no error)=w43) -> ()  [unwired: 1 in, 3 out]
  n887 = Destroy User Event(user event=w65, error in=w43) -> ()  [unwired: 1 out]
  n888 = Unregister For Events(event registration refnum=w57, error in=w43) -> ()  [unwired: 1 out]
